vi "1820_TC_GUI.vi"() -> ()   [LabVIEW 2016]
uses:
  Leiden-TC/trunk/1. Sources TC/lib/Lib.llb/CS.lvclass
  Leiden-TC/trunk/1. Sources TC/lib/Lib.llb/TCS.lvclass
  C:/user/patrick/Leiden-TC/1. Sources TC/lib/Lib.llb/CS.lvclass
  Leiden-TC/trunk/1. Sources TC/lib/Lib.llb/QCS.lvclass
  Leiden-TC/trunk/1. Sources TC/lib/Lib.llb/CS Emulation.lvclass
  Leiden-TC/trunk/1. Sources TC/lib/Lib.llb/PCS.lvclass
panel:
  out "Name":string
  out "SetControl":T1
  out "ControlNames":string[](array[string])
  out "VIRef":T2 {"Array DataType" format="%.0x"; "WaveForm Type" format="%.0x"; "RefNum Type" format="%.0x"; "DataType" format="%.0x"}
  out "Scan Parameters":cluster{string, "Freq":dbl, "V_exc":dbl}
  out "zConfig":path=path "C:/Users/Sasha/Dropbox/Labview/LC Software/ImpSoft-V5.2.2-multithreaded/ImpBridgeLabview/ImpBridgeDll.dll"
  out "TempStabilized":refnum<user-event>
  out "Actual I":dbl[](array[numeric])
  out "VI called?":bool=TRUE
  out "Error code":u8
  out "UpdateChannelInfo":refnum<user-event>
  out "zBridge set nr.":u8
  out "zDll":path=path "C:/Users/Sasha/Dropbox/Labview/LC Software/ImpSoft-V5.2.2-multithreaded/ImpBridgeLabview/ImpBridgeDll.dll"
  in  "String":string="^ Click the Run button to start the program "
  in  "Toolbar":enum32{"Page 1", "Page 2"}(tab)
  in  "Load config":bool
  in  "Start":bool
  in  "Load Data":bool
  in  "Pause":bool
  in  "Stop":bool
  in  "Copy to Clipboard":bool
  in  "Save to Cal Log":bool
  in  "Save config":bool
  in  "Save Data":bool
  in  "Clear all plots":bool
  in  "ColorBox":enum32{"Page 1", "Page 2"}(tab)
  in  "Colors":picture
  out "Color":u32(colorbox)
  in  "LogFileCreationTime":timestamp=timestamp(2742897600 s since 1904-01-01)
  out "UpdateLogFilePath":refnum<user-event>
  out "Calib path":path=path "C:/avs-47/aaaa"
  out "Log path":path
  out "TCS port":i32(ring)=3 items=["COM1", "COM2", "COM3", "COM4", "COM5", "COM6", "COM7", "COM8", "COM9", "PRN1", "PRN2", "PRN3", "PRN4"]
  out "UpdateCalibrations":refnum<user-event>
  out "AVS VISA session":refnum<visa-resource-name>="COM3"
  in  "Minimize 2":bool
  out "Revision":string="TC" caption="V"
  in  "Minimize":bool
  out "Current1flow":bool
  out "Current2flow":bool
  in  "Tab Control":enum32{"AVS"}(tab)
  in  "Channel Controls":T3(tab)=enum."All"
  out "T0":dbl=nan caption="T" format="%#.2p"
  out "R0":dbl caption="R" format="%.3p"
  out "R-Plot 0":cluster{dbl[], dbl[]}(graph) caption="R-Plot"
  out "T1":dbl=nan caption="T" format="%#.2p"
  out "R1":dbl caption="R" format="%.3p"
  out "R-Plot 1":cluster{dbl[], dbl[]}(graph) caption="R-Plot"
  out "T2":dbl=nan caption="T" format="%#.2p"
  out "R2":dbl caption="R" format="%.3p"
  out "R-Plot 2":cluster{dbl[], dbl[]}(graph) caption="R-Plot"
  out "T3":dbl=nan caption="T" format="%#.2p"
  out "R3":dbl caption="R" format="%.3p"
  out "R-Plot 3":cluster{dbl[], dbl[]}(graph) caption="R-Plot"
  out "T4":dbl=nan caption="T" format="%#.2p"
  out "R4":dbl caption="R" format="%.3p"
  out "R-Plot 4":cluster{dbl[], dbl[]}(graph) caption="R-Plot"
  out "T5":dbl=nan caption="T" format="%#.2p"
  out "R5":dbl caption="R" format="%.3p"
  out "R-Plot 5":cluster{dbl[], dbl[]}(graph) caption="R-Plot"
  out "T6":dbl=nan caption="T" format="%#.2p"
  out "R6":dbl caption="R" format="%.3p"
  out "R-Plot 6":cluster{dbl[], dbl[]}(graph) caption="R-Plot"
  out "T7":dbl=nan caption="T" format="%#.2p"
  out "R7":dbl caption="R" format="%.3p"
  out "R-Plot 7":cluster{dbl[], dbl[]}(graph) caption="R-Plot"
  out "T8":dbl=nan caption="T" format="%#.2p"
  out "R8":dbl caption="R" format="%.3p"
  out "R-Plot 8":cluster{dbl[], dbl[]}(graph) caption="R-Plot"
  out "T9":dbl=nan caption="T" format="%#.2p"
  out "R9":dbl caption="R" format="%.3p"
  out "R-Plot 9":cluster{dbl[], dbl[]}(graph) caption="R-Plot"
  out "T":T4 {"T0 3" format="%.2p"; "T0 2" format="%.2p"; "T0" format="%.2p"; "T0" format="%.2p"; "T0" format="%.2p"; "T0" format="%.2p"; "T0" format="%.2p"; "T0" format="%.2p"; "T0" format="%.2p"; "T0" format="%.2p"}
  in  "AVS names":T5={"AVS Name 0"="3K", "AVS Name 1"="Still", "AVS Name 2"="50 mK", "AVS Name 3"="MC", "AVS Name 4"="MC", "AVS Name 5"="", "AVS Name 6"="", "AVS Name 7"="", "AVS Name 8"="", "AVS Name 9"=""}
  in  "Edit Calibrations":T6
  in  "Thermometer":T7 {"Select sensor 10" items=["No Calibration.vi"]; "Select sensor 9" items=["No Calibration.vi"]; "Select sensor 8" items=["No Calibration.vi"]; "Select sensor 7" items=["No Calibration.vi"]; "Select sensor 6" items=["No Calibration.vi"]; "Select sensor 5" items=["No Calibration.vi"]; "Select sensor 4" items=["No Calibration.vi"]; "Select sensor 3" items=["No Calibration.vi"]; "Select sensor 2" items=["No Calibration.vi"]; "Select sensor 1" items=["No Calibration.vi"]}
  out "Units":T5
  out "R":T8={"R0"=0.0, "R1"=0.0, "R2"=-0.0, "R3"=0.0, "R4"=0.0, "R5"=0.0, "R6"=0.0, "R7"=0.0, "R6 2"=0.0, "R7 2"=0.0} {"R7 2" format="%.3p"; "R6 2" format="%.3p"; "R7" format="%.3p"; "R6" format="%.3p"; "R5" format="%.3p"; "R4" format="%.3p"; "R3" format="%.3p"; "R2" format="%.3p"; "R1" format="%.3p"; "R0" format="%.3p"}
  in  "Scan Parameters":enum32{"Page 1", "Page 2"}(tab)
  in  "Exc&Ranges":T9={"Excitationl 0"=4, "Excitationl 0"=4, "Excitationl 0"=3, "Excitationl 0"=3, "Excitationl 0"=3, "Excitationl 0"=3, "Excitationl 0"=3, "Excitationl 0"=3, "Range 0"=5, "Range 0"=5, "Range 0"=5, "Range 0"=5, "Range 0"=5, "Range 0"=5, "Range 0"=5, "Range 0"=5} {"Range 0" items=["n.a."=-1, "open"=0, "2 Ohm"=1, "20 Ohm"=2, "200 Ohm"=3, "2k Ohm"=4, "20k Ohm"=5, "200k Ohm"=6, "2M Ohm"=7]; "Range 0" items=["n.a."=-1, "open"=0, "2 Ohm"=1, "20 Ohm"=2, "200 Ohm"=3, "2k Ohm"=4, "20k Ohm"=5, "200k Ohm"=6, "2M Ohm"=7]; "Range 0" items=["n.a."=-1, "open"=0, "2 Ohm"=1, "20 Ohm"=2, "200 Ohm"=3, "2k Ohm"=4, "20k Ohm"=5, "200k Ohm"=6, "2M Ohm"=7]; "Range 0" items=["n.a."=-1, "open"=0, "2 Ohm"=1, "20 Ohm"=2, "200 Ohm"=3, "2k Ohm"=4, "20k Ohm"=5, "200k Ohm"=6, "2M Ohm"=7]; "Range 0" items=["n.a."=-1, "open"=0, "2 Ohm"=1, "20 Ohm"=2, "200 Ohm"=3, "2k Ohm"=4, "20k Ohm"=5, "200k Ohm"=6, "2M Ohm"=7]; "Range 0" items=["n.a."=-1, "open"=0, "2 Ohm"=1, "20 Ohm"=2, "200 Ohm"=3, "2k Ohm"=4, "20k Ohm"=5, "200k Ohm"=6, "2M Ohm"=7]; "Range 0" items=["n.a."=-1, "open"=0, "2 Ohm"=1, "20 Ohm"=2, "200 Ohm"=3, "2k Ohm"=4, "20k Ohm"=5, "200k Ohm"=6, "2M Ohm"=7]; "Range 0" items=["n.a."=-1, "open"=0, "2 Ohm"=1, "20 Ohm"=2, "200 Ohm"=3, "2k Ohm"=4, "20k Ohm"=5, "200k Ohm"=6, "2M Ohm"=7]; "Excitationl 0" items=["none", "3 µV", "10 µV", "30 µV", "100 µV", "300 µV", "1 mV", "3 mV"]; "Excitationl 0" items=["none", "3 µV", "10 µV", "30 µV", "100 µV", "300 µV", "1 mV", "3 mV"]; "Excitationl 0" items=["none", "3 µV", "10 µV", "30 µV", "100 µV", "300 µV", "1 mV", "3 mV"]; "Excitationl 0" items=["none", "3 µV", "10 µV", "30 µV", "100 µV", "300 µV", "1 mV", "3 mV"]; "Excitationl 0" items=["none", "3 µV", "10 µV", "30 µV", "100 µV", "300 µV", "1 mV", "3 mV"]; "Excitationl 0" items=["none", "3 µV", "10 µV", "30 µV", "100 µV", "300 µV", "1 mV", "3 mV"]; "Excitationl 0" items=["none", "3 µV", "10 µV", "30 µV", "100 µV", "300 µV", "1 mV", "3 mV"]; "Excitationl 0" items=["none", "3 µV", "10 µV", "30 µV", "100 µV", "300 µV", "1 mV", "3 mV"]}
  out "Status":T10
  out "zBridge params":T5
  out "uPlots":T11
  in  "Autorange":bool=TRUE
  out "Active":T12={"active Channel 0"=TRUE, "active Channel 1"=TRUE, "active Channel 2"=TRUE, "active Channel 3"=FALSE, "active Channel 4"=FALSE, "active Channel 5"=FALSE, "active Channel 6"=FALSE, "active Channel 7"=FALSE, "active Channel 8"=FALSE, "active Channel 9"=FALSE}
  out "PID-Plot":cluster{"Numeric":dbl, "R/T":dbl}(graph)
  in  "HW Address":u32
  in  "Edit calibration":bool
  in  "Convert":bool
  out "T7":dbl caption="T=" format="%#.2p"
  in  "QuickR":dbl caption="R=" format="%_6g"
  in  "Select sensor 1":u16(ring) items=["No Calibration.vi"]
  out "I_list[i]":dbl[](array[numeric]) min=-1.0
  out "I_in":dbl[](array[numeric]) min=-1.0
  in  "Tab Control 5":enum32{"Page 1", "Page 2"}(tab)
  in  "Data History":enum32{"History", "Settings"}(tab)=enum."Settings"
  in  "Mode Buttons":T13(radio)
  in  "Erase All":bool
  out "AVS names small":T5={"AVS Name 0"="3K", "AVS Name 1"="Still", "AVS Name 2"="50 mK", "AVS Name 3"="MC", "AVS Name 4"="MC", "AVS Name 5"="", "AVS Name 6"="", "AVS Name 7"="", "AVS Name 8"="", "AVS Name 9"=""}
  out "Active channel":T14
  out "Small T":T15 caption="T" {"R1" format="%#.2p"; "R1" format="%#.2p"; "R1" format="%#.2p"; "R1" format="%#.2p"; "R1" format="%#.2p"; "R1" format="%#.2p"; "R1" format="%#.2p"; "R1" format="%#.2p"; "R1" format="%#.2p"; "R1" format="%#.2p"}
  out "Small R":T16 caption="R" {"R1 2" format="%#_5p"; "R1 2" format="%#_5p"; "R1 2" format="%#_5p"; "R1 2" format="%#_5p"; "R1 2" format="%#_5p"; "R1 2" format="%#_5p"; "R1 2" format="%#_5p"; "R1 2" format="%#_5p"; "R1 2" format="%#_5p"; "R1 2" format="%#_5p"}
  out "Time":dbl format="%<%X\n%x>T"
  in  "AVS Runtime Settings":T17={"Read AVS channels from"=0, "Last Channel"=7, "Delay Between Scans"=0, "Stabilisation Delay"=0.5, "Averages"=2, "Data Memory"=5000, "Filter graphs:"=FALSE, "Y_min"=0.0, "Y_max"=2000000.0, "Plot type"=enum."T vs Time", "Allow neg R"=TRUE, "Data Memory 2"=30.0} {"Data Memory 2" min=0.0; "Delay Between Scans" format="%.0f s"; "Averages" min=1 max=1000; "Stabilisation Delay" min=0.5; "Last Channel" min=0 max=7 step=1; "Read AVS channels from" min=0 max=7 step=1; "Y_max" format="%#_6f"; "Y_min" min=0.0 format="%#_6f"; "Data Memory" min=3 max=30000}
  out "I":dbl[](array[numeric])
  in  "Data":cluster{"R":dbl[], "T":dbl[], "Time":dbl[]}[](array[cluster])=[{"R"=[], "T"=[], "Time"=[]}, {"R"=[0.0, 2.0], "T"=[], "Time"=[]}]
  out "Int":dbl=10.0 format="%#.2f"
  out "T_array":dbl[](array[numeric])
  in  "Data array":dbl[](array[numeric])
  out "I3_SetPnt":dbl
  out "Currents changed":bool
  in  "Excitations":T18={"Excitationl 0"=4, "Excitation 1"=4, "Excitation 2"=3, "Excitation 3"=3, "Excitation 4"=3, "Excitation 5"=3, "Excitation 6"=3, "Excitation 7"=3} {"Excitation 7" items=["none", "3 µV", "10 µV", "30 µV", "100 µV", "300 µV", "1 mV", "3 mV"]; "Excitation 6" items=["none", "3 µV", "10 µV", "30 µV", "100 µV", "300 µV", "1 mV", "3 mV"]; "Excitation 5" items=["none", "3 µV", "10 µV", "30 µV", "100 µV", "300 µV", "1 mV", "3 mV"]; "Excitation 4" items=["none", "3 µV", "10 µV", "30 µV", "100 µV", "300 µV", "1 mV", "3 mV"]; "Excitation 3" items=["none", "3 µV", "10 µV", "30 µV", "100 µV", "300 µV", "1 mV", "3 mV"]; "Excitation 2" items=["none", "3 µV", "10 µV", "30 µV", "100 µV", "300 µV", "1 mV", "3 mV"]; "Excitation 1" items=["none", "3 µV", "10 µV", "30 µV", "100 µV", "300 µV", "1 mV", "3 mV"]; "Excitationl 0" items=["none", "3 µV", "10 µV", "30 µV", "100 µV", "300 µV", "1 mV", "3 mV"]}
  in  "Ranges":T18={"Excitationl 0"=5, "Excitation 1"=5, "Excitation 2"=5, "Excitation 3"=5, "Excitation 4"=5, "Excitation 5"=5, "Excitation 6"=5, "Excitation 7"=5} {"Excitation 7" items=["n.a."=-1, "open"=0, "2 Ohm"=1, "20 Ohm"=2, "200 Ohm"=3, "2k Ohm"=4, "20k Ohm"=5, "200k Ohm"=6, "2M Ohm"=7]; "Excitation 6" items=["n.a."=-1, "open"=0, "2 Ohm"=1, "20 Ohm"=2, "200 Ohm"=3, "2k Ohm"=4, "20k Ohm"=5, "200k Ohm"=6, "2M Ohm"=7]; "Excitation 5" items=["n.a."=-1, "open"=0, "2 Ohm"=1, "20 Ohm"=2, "200 Ohm"=3, "2k Ohm"=4, "20k Ohm"=5, "200k Ohm"=6, "2M Ohm"=7]; "Excitation 4" items=["n.a."=-1, "open"=0, "2 Ohm"=1, "20 Ohm"=2, "200 Ohm"=3, "2k Ohm"=4, "20k Ohm"=5, "200k Ohm"=6, "2M Ohm"=7]; "Excitation 3" items=["n.a."=-1, "open"=0, "2 Ohm"=1, "20 Ohm"=2, "200 Ohm"=3, "2k Ohm"=4, "20k Ohm"=5, "200k Ohm"=6, "2M Ohm"=7]; "Excitation 2" items=["n.a."=-1, "open"=0, "2 Ohm"=1, "20 Ohm"=2, "200 Ohm"=3, "2k Ohm"=4, "20k Ohm"=5, "200k Ohm"=6, "2M Ohm"=7]; "Excitation 1" items=["n.a."=-1, "open"=0, "2 Ohm"=1, "20 Ohm"=2, "200 Ohm"=3, "2k Ohm"=4, "20k Ohm"=5, "200k Ohm"=6, "2M Ohm"=7]; "Excitationl 0" items=["n.a."=-1, "open"=0, "2 Ohm"=1, "20 Ohm"=2, "200 Ohm"=3, "2k Ohm"=4, "20k Ohm"=5, "200k Ohm"=6, "2M Ohm"=7]}
  out "CS ref":refnum<class "CS.lvclass">
  out "start 2":bool
  in  "Current indicators":enum32{"Page 1", "Page 2"}(tab)
  out "Automatic mode 0":bool
  out "Automatic mode 1":bool
  out "Map Channel 0 to 2":T19(ring) caption="Output to"
  in  "uA 0":u32
  in  "CS Names":T20={"CS Name 0"="N.C.", "CS Name 1"="3K", "CS Name 2"="Still", "CS Name 3"="MC"}
  out "I0":T21={"uA"="000", "ON"=FALSE, "Gated"=FALSE, "current flows"=FALSE, "Error"=FALSE} caption="Ch0 -"
  in  "uA 3":u32
  in  "uA 2":u32
  in  "uA 1":u32
  out "Automatic mode 3":bool
  out "Automatic mode 2":bool
  out "I3":T21={"uA"="000", "ON"=FALSE, "Gated"=FALSE, "current flows"=FALSE, "Error"=FALSE} caption="Chn 3"
  out "I2":T21={"uA"="000", "ON"=FALSE, "Gated"=FALSE, "current flows"=FALSE, "Error"=FALSE} caption="Chn 2"
  out "I1":T21={"uA"="000", "ON"=FALSE, "Gated"=FALSE, "current flows"=FALSE, "Error"=FALSE} caption="Chn 1"
  out "I_0":dbl=10.0
  out "vi reference":refnum<vi>
  in  "Show PID graph?":bool
  in  "Set Color":bool
  in  "Save Screen Data":bool
  in  "CS Ch3 mode":enum32{"Page 1", "Page 2"}(tab)=enum."Page 2"
  in  "T Sweep":T22={"Start value"=200.0, "End value"=250.0, "Step"=10.0, "Current"=0.0, "I_next"=FALSE, "I_prev"=FALSE, "Interrrupt Sweep"=FALSE, "Start"=FALSE, "Boolean"=TRUE} {"Step" min=0.0; "End value" min=0.0; "Start value" min=0.0}
  out "CallExtVI":refnum<user-event>
  out "Unit":string
  out "UpdateValuesAVS":refnum<user-event>
  out "DoPID":refnum<user-event>
  out "UpdateValuesZBridge":refnum<user-event>
  out "zBridge params/Error":string
  out "CurCalibrations":T23
  out "LMB Down":bool
  out "T controlled":dbl
  out "ResetPIDloop":refnum<user-event>
  in  "Tab Control 2":T24(tab)=enum."Current source control"
  in  "Refresh Calibrations":bool
  in  "Save Screen Data 2":bool
  out "ID":string
  out "Bridge status":errorcluster
  out "CS status":errorcluster
  out "General":errorcluster caption="General status"
  in  "Bridge settings":T25={"AVS type"=enum."AVS47A (GPIB interface)", "AVS_SPort"="COM5", "Address"="GPIB0::20::INSTR", "AVS_CalFolder"=path "E:/Dropbox/Labview/LC Software/All Calibrations"}
  in  "Current source settings":T26={"TCS_Port"="COM1", "TCS_Imax"=5, "CS type"=enum."TCS", "QCS/PCS Device"=0}
  in  "Data logging":T27={"AVS_Path"=path "C:/avs-47", "AVS_FName"="LogAVS", "CAL_FName"="calibration", "Filenames suffix"="_%Y-%m-%d-%H-%M-%S", "Delimeter"="\t", "NewFevery"=7, "Time Units"=enum."Days", "Date/Time Format"="%Y-%m-%d %H:%M:%S", "External VI path"=path "C:/Users/User1/Dropbox/Labview/LC Software/TempControl/OnTempStabilized Ext VI Laurens.vi", "VI state:"=enum."Bad", "Ask on start?"=FALSE, "Run description"="\n"}
  in  "I_list":dbl[][](array[numeric]) min=-1.0
  out "T Channel":bool[](array[boolean])
  in  "Trigger other running TC instances":bool
  in  "I_Clear":bool
  in  "I3 as temp":cluster{"I3 as temp 2":bool}
  in  "C_I3":T28={"Toggle ON/OFF"=FALSE, "Toggle Gated"=FALSE, "I"=0, "Range"=enum."x1 uA"} caption="I3" {"I" max=100000 step=1}
  in  "C_I2":T28={"Toggle ON/OFF"=FALSE, "Toggle Gated"=FALSE, "I"=0, "Range"=enum."x1 uA"} caption="I2" {"I" max=100000 step=1}
  in  "C_I1":T28={"Toggle ON/OFF"=FALSE, "Toggle Gated"=FALSE, "I"=0, "Range"=enum."x1 uA"} caption="I1" {"I" max=100000 step=1}
  in  "C_I0":T28={"Toggle ON/OFF"=FALSE, "Toggle Gated"=FALSE, "I"=0, "Range"=enum."x1 uA"} caption="I0" {"I" max=100000 step=1}
  in  "I0 output to":T29(ring) caption="Set QCS Channel 0 output to"
  in  "CS Mode":enum16{"Manual", "Automatic"}(ring) caption="CS control mode"
  in  "Write to log":bool
  in  "Load from file":bool
  in  "Save to file":bool
  in  "I_tofirst":bool
  in  "I_next":bool
  in  "I_prev":bool
  out "VI state:":T30(ring)
  out "I_selection":bool[](array[boolean])=[TRUE, FALSE, FALSE, FALSE, FALSE, FALSE, FALSE, FALSE, FALSE, FALSE]
  in  "Call external VI":bool
  out "Time Old":dbl format="%#_16g"
  in  "Automode Settings 2":T31={"AVS Channel"=0, "N averages"=10, "Delay Time"=10.0, "T stability"=0.3, "FB on"=enum."Temperature"} {"Delay Time" min=0.0 format="%#_g min"; "AVS Channel" min=-1 max=9 step=1}
  in  "Automode 2":bool=TRUE caption="Enable automatic sweeping/list iteration"
  in  "PID setup 2":T32={"Current limit, [uA]"=10000.0, "Proportional Gain"=3.0, "Integral Gain"=3.0, "Derivative Gain"=1.0, "SP tolerance"=0.1, "Feed Fwd Gain [uA/mK]"=0.0, "Integral Gain Bandwidth"=10.0, "Integral Gain Background"=1.0, "FB on 2"=enum."1"} {"Integral Gain Background" format="%#.6g"; "Integral Gain Bandwidth" format="%#.6g"; "Feed Fwd Gain [uA/mK]" format="%#.5g"; "SP tolerance" format="%#.5g"; "Derivative Gain" format="%#.6g"; "Integral Gain" format="%#.6g"; "Proportional Gain" format="%#.6g"; "Current limit, [uA]" format="%#.5g"}
  in  "Reset PID":bool
  in  "Next step":bool
  out "I_list_idx":i32=10 caption="Point #"
  out "I_list_idx_max":i32=10 caption="of"
  out "Timer":dbl format="%<%H:%M:%S>t"
  out "Slope":dbl format="%#_3g %"
  out "Error":dbl=10.0 format="%#_6f"
  out "SP reached?":bool
  # "Quick convert R->T:"
  # "Ohm"
  # "mK"
  # "Ch#"
  # "Miniplot"
  # "Channel parameters"
  # "Impedance"
  # "Unit"
  # "Type of sensor"
  # "T [mK]"
  # "Description"
  # "0"
  # "1"
  # "2"
  # "3"
  # "4"
  # "5"
  # "6"
  # "7"
  # "8"
  # "9"
  # "0"
  # "1"
  # "2"
  # "3"
  # "4"
  # "5"
  # "7"
  # "8"
  # "9"
  # "6"
  # "auto"
  # "auto"
  # "auto"
  # "auto"
  # "gated"
  # "gated"
  # "gated"
  # "gated"
  # "Ch3"
  # "Current source mode"
  # "Current source manual control"
  # "Automatic mode or current source"
  # "Currents List"
  # "Settings"
  # "I0"
  # "I1"
  # "I2"
  # "I3"
  # "Status"
  # "On temperature stabilized"
types:
  T1 = cluster{"Name":string, "Scalar":string, "Array":string[][]}
  T2 = cluster{"Control Ref ID":refnum<vi>[], "Full Name":string[], "ClassID":enum16{"<Null>", "1", "2", "Generic", "Decoration", "Text", "Control", "ColorBox", "Boolean", "RefNum", "Variant", "Path", "ListBox", "Table", "Array", "Picture", "ActiveXContainer", "Numeric", "Digital", "NamedNumeric", "ColorRamp", "Slide", "GraphOrChart", "WaveformChart", "WaveformGraph", "IntensityChart", "IntensityGraph", "String", "IOName", "ComboBox", "Cluster", "Panel", "Knob", "NumWithScale", "Ring", "Enum", "GObject", "Plot", "Cursor", "NumericText", "Scale", "ColorScale", "GraphScale", "ColorGraphScale", "TypedRefNum", "OldKnobScale", "MCListbox", "MeasureData", "BVTag", "DAQName", "VISAName", "IVIName", "SlideScale", "TabControl", "Page", "TabArrayTabControl", "ConPane", "57", "58", "59", "60", "61", "62", "63", "64", "SubPanel", "TreeControl", "67", "68", "69", "70", "71", "72", "73", "74", "75", "SplitterBar"}[], "Short Name":string[], "DataType":enum8{"<Null>", "I8", "I16", "I32", "I64", "U8", "U16", "U32", "U64", "SGL", "DBL", "EXT", "CSG", "CDB", "CXT", "0x0F", "0x10", "0x11", "0x12", "0x13", "0x14", "Enum U8", "Enum U16", "Enum U32", "Enum U64", "SGL PQ", "DBL PQ", "EXT PQ", "CSG PQ", "CDB PQ", "CXT PQ", "0x1F", "0x20", "Boolean", "0x22", "0x23", "0x24", "0x25", "0x26", "0x27", "0x28", "0x29", "0x2A", "0x2B", "0x2C", "0x2D", "0x2E", "0x2F", "String", "0x31", "Path", "Pict", "0x34", "0x35", "0x36", "DAQ", "0x38", "0x39", "0x3A", "0x3B", "0x3C", "0x3D", "0x3E", "0x3F", "Array", "0x41", "0x42", "0x43", "0x44", "0x45", "0x46", "0x47", "0x48", "0x49", "0x4A", "0x4B", "0x4C", "0x4D", "0x4E", "0x4F", "Cluster", "0x51", "0x52", "Variant", "Waveform", "0x55", "0x56", "0x57", "0x58", "0x59", "0x5A", "0x5B", "0x5C", "0x5D", "0x5E", "0x5F", "0x60", "0x61", "0x62", "0x63", "0x64", "0x65", "0x66", "0x67", "0x68", "0x69", "0x6A", "0x6B", "0x6C", "0x6D", "0x6E", "0x6F", "Refnum"}[], "RefNum Type":enum8{"Generic", "Datalog File Refnum", "Byte Stream File Refnum", "Device Refnum", "Occurence Refnum", "TCP Connection Refnum", "VISA Refnum (Obsolete)", "Automation Renum", "VI Server Refnum", "Menu Refnum", "IVI Refnum (Obsolete)", "IMAQ Session", "0x0C", "Datasocket Refnum", "VISA Resource", "IVI Logical Name", "UDP Connection Refnum", "Notifier Refnum", "Queue Refnum", "IrDA Refnum", "Hardware Plugin Refnum", "Hardware Plugin Tag Refnum", "DAQmx Refnum", "Event Registration Refnum", ".NET Refnum", "User Event Refnum", "0x1A", "Event Callback", "0x1C", "0x1D", "Only Used Internal to LabVIEW", "Bluetooth", "Data Value References", "RT FIFO", "TDM Streaming"}[], "WaveForm Type":enum8{"<Not a Waveform Type>", "0x01", "Analog 16-bit signed", "Analog Double-Precision", "0x04", "Analog Single Precision", "Timestamp", "Digital Data", "Digital Waveform", "Dynamic Data", "Analog Extended-Precision", "Analog 8-bit unsigned", "Analog 16-bit unsigned", "Analog 32-bit unsigned", "Analog 8-bit signed", "Analog 32-bit signed", "Analog Complex Single-Precision", "Analog Complex Double-Precision", "Analog Complex Extended Precision", "Analog 64-bit signed", "Analog 64-bit unsigned"}[], "Parent":i32[], "Array DataType":enum8{"<Null>", "I8", "I16", "I32", "I64", "U8", "U16", "U32", "U64", "SGL", "DBL", "EXT", "CSG", "CDB", "CXT", "0x0F", "0x10", "0x11", "0x12", "0x13", "0x14", "Enum U8", "Enum U16", "Enum U32", "Enum U64", "SGL PQ", "DBL PQ", "EXT PQ", "CSG PQ", "CDB PQ", "CXT PQ", "0x1F", "0x20", "Boolean", "0x22", "0x23", "0x24", "0x25", "0x26", "0x27", "0x28", "0x29", "0x2A", "0x2B", "0x2C", "0x2D", "0x2E", "0x2F", "String", "0x31", "Path", "Pict", "0x34", "0x35", "0x36", "DAQ", "0x38", "0x39", "0x3A", "0x3B", "0x3C", "0x3D", "0x3E", "0x3F", "Array", "0x41", "0x42", "0x43", "0x44", "0x45", "0x46", "0x47", "0x48", "0x49", "0x4A", "0x4B", "0x4C", "0x4D", "0x4E", "0x4F", "Cluster", "0x51", "0x52", "Variant", "Waveform", "0x55", "0x56", "0x57", "0x58", "0x59", "0x5A", "0x5B", "0x5C", "0x5D", "0x5E", "0x5F", "0x60", "0x61", "0x62", "0x63", "0x64", "0x65", "0x66", "0x67", "0x68", "0x69", "0x6A", "0x6B", "0x6C", "0x6D", "0x6E", "0x6F", "Refnum"}[], "Owning VI":refnum<vi>[], "Active?":bool[]}
  T3 = enum32{"0", "1", "2", "3", "4", "5", "6", "7", "8", "9", "All", "PID loop"}
  T4 = cluster{"T0":dbl, "T0":dbl, "T0":dbl, "T0":dbl, "T0":dbl, "T0":dbl, "T0":dbl, "T0":dbl, "T0 2":dbl, "T0 3":dbl}
  T5 = cluster{"AVS Name 0":string, "AVS Name 1":string, "AVS Name 2":string, "AVS Name 3":string, "AVS Name 4":string, "AVS Name 5":string, "AVS Name 6":string, "AVS Name 7":string, "AVS Name 8":string, "AVS Name 9":string}
  T6 = cluster{"Boolean":bool, "Boolean 2":bool, "Boolean 3":bool, "Boolean 4":bool, "Boolean 5":bool, "Boolean 6":bool, "Boolean 7":bool, "Boolean 8":bool, "Boolean 9":bool, "Boolean 10":bool}
  T7 = cluster{"Select sensor 1":u16, "Select sensor 2":u16, "Select sensor 3":u16, "Select sensor 4":u16, "Select sensor 5":u16, "Select sensor 6":u16, "Select sensor 7":u16, "Select sensor 8":u16, "Select sensor 9":u16, "Select sensor 10":u16}
  T8 = cluster{"R0":dbl, "R1":dbl, "R2":dbl, "R3":dbl, "R4":dbl, "R5":dbl, "R6":dbl, "R7":dbl, "R6 2":dbl, "R7 2":dbl}
  T9 = cluster{"Excitationl 0":i16, "Excitationl 0":i16, "Excitationl 0":i16, "Excitationl 0":i16, "Excitationl 0":i16, "Excitationl 0":i16, "Excitationl 0":i16, "Excitationl 0":i16, "Range 0":i16, "Range 0":i16, "Range 0":i16, "Range 0":i16, "Range 0":i16, "Range 0":i16, "Range 0":i16, "Range 0":i16}
  T10 = cluster{"Numeric":dbl, "Numeric":dbl, "Numeric":dbl, "Numeric":dbl, "Numeric":dbl, "Numeric":dbl, "Numeric":dbl, "Numeric":dbl, "Numeric":dbl, "Numeric":dbl}
  T11 = cluster{"uPlot 0":cluster{dbl[], dbl[]}, "uPlot 1":cluster{dbl[], dbl[]}, "uPlot 2":cluster{dbl[], dbl[]}, "uPlot 3":cluster{dbl[], dbl[]}, "uPlot 4":cluster{dbl[], dbl[]}, "uPlot 5":cluster{dbl[], dbl[]}, "uPlot 6":cluster{dbl[], dbl[]}, "uPlot 7":cluster{dbl[], dbl[]}, "uPlot 8":cluster{dbl[], dbl[]}, "uPlot 9":cluster{dbl[], dbl[]}}
  T12 = cluster{"active Channel 0":bool, "active Channel 1":bool, "active Channel 2":bool, "active Channel 3":bool, "active Channel 4":bool, "active Channel 5":bool, "active Channel 6":bool, "active Channel 7":bool, "active Channel 8":bool, "active Channel 9":bool}
  T13 = enum32{"No Selection", "Cursor Mode", "Erase point", "Erase Range"}
  T14 = cluster{"Boolean 5":bool, "Boolean 5":bool, "Boolean 5":bool, "Boolean 5":bool, "Boolean 5":bool, "Boolean 5":bool, "Boolean 5":bool, "Boolean 5":bool, "Boolean 5":bool, "Boolean 5":bool}
  T15 = cluster{"R1":dbl, "R1":dbl, "R1":dbl, "R1":dbl, "R1":dbl, "R1":dbl, "R1":dbl, "R1":dbl, "R1":dbl, "R1":dbl}
  T16 = cluster{"R1 2":dbl, "R1 2":dbl, "R1 2":dbl, "R1 2":dbl, "R1 2":dbl, "R1 2":dbl, "R1 2":dbl, "R1 2":dbl, "R1 2":dbl, "R1 2":dbl}
  T17 = cluster{"Read AVS channels from":i8, "Last Channel":i8, "Delay Between Scans":u32, "Stabilisation Delay":dbl, "Averages":u16, "Data Memory":u16, "Filter graphs:":bool, "Y_min":dbl, "Y_max":dbl, "Plot type":enum16{"R vs Time", "T vs Time"}, "Allow neg R":bool, "Data Memory 2":dbl}
  T18 = cluster{"Excitationl 0":i16, "Excitation 1":i16, "Excitation 2":i16, "Excitation 3":i16, "Excitation 4":i16, "Excitation 5":i16, "Excitation 6":i16, "Excitation 7":i16}
  T19 = enum16{"Chn 0", "Aux 0", "Aux 1", "Aux 2", "Aux 3"}
  T20 = cluster{"CS Name 0":string, "CS Name 1":string, "CS Name 2":string, "CS Name 3":string}
  T21 = cluster{"uA":string, "ON":bool, "Gated":bool, "current flows":bool, "Error":bool}
  T22 = cluster{"Start value":dbl, "End value":dbl, "Step":dbl, "Current":dbl, "I_next":bool, "I_prev":bool, "Interrrupt Sweep":bool, "Start":bool, "Boolean":bool}
  T23 = cluster{"[0]":string, "[1]":string, "[2]":string, "[3]":string, "[4]":string, "[5]":string, "[6]":string, "[7]":string, "[8]":string, "[9]":string}
  T24 = enum32{"Devices Settings", "Current source control"}
  T25 = cluster{"AVS type":enum16{"AVS47A (GPIB interface)", "AVS47B (RS232 interface)", "AVS48", "AVS Emulation", "Impedance Bridge", "Disabled"}, "AVS_SPort":refnum<visa-resource-name>, "Address":refnum<visa-resource-name>, "AVS_CalFolder":path}
  T26 = cluster{"TCS_Port":refnum<visa-resource-name>, "TCS_Imax":i32, "CS type":enum16{"TCS", "QCS v1", "PCS (n.a.)", "CS Emulation", "Disabled"}, "QCS/PCS Device":u16}
  T27 = cluster{"AVS_Path":path, "AVS_FName":string, "CAL_FName":string, "Filenames suffix":string, "Delimeter":string, "NewFevery":u32, "Time Units":enum16{"Minutes", "Hours", "Days"}, "Date/Time Format":string, "External VI path":path, "VI state:":enum32{"Bad", "Idle", "Run top level", "Running"}, "Ask on start?":bool, "Run description":string}
  T28 = cluster{"Toggle ON/OFF":bool, "Toggle Gated":bool, "I":u32, "Range":enum8{"Auto", "x1 uA", "x10 uA", "x100 uA", "x1 mA"}}
  T29 = enum16{"Channel 0", "Aux 0", "Aux 1", "Aux 2", "Aux 3"}
  T30 = enum32{"Bad", "Idle", "Run top level", "Running"}
  T31 = cluster{"AVS Channel":i32, "N averages":i32, "Delay Time":dbl, "T stability":dbl, "FB on":enum16{"Resistance", "Temperature"}}
  T32 = cluster{"Current limit, [uA]":dbl, "Proportional Gain":dbl, "Integral Gain":dbl, "Derivative Gain":dbl, "SP tolerance":dbl, "Feed Fwd Gain [uA/mK]":dbl, "Integral Gain Bandwidth":dbl, "Integral Gain Background":dbl, "FB on 2":enum16{"0", "1", "2", "3"}}
  T33 = cluster{"error":bool, "code":i32, "source":string}
  T34 = enum32{"No Selection", "Erase Data", "Erase Range", "Cursor Mode"}
  T35 = enum16{"AVS47A (GPIB interface)", "AVS47B (RS232 interface)", "AVS48", "AVS Emulation", "Impedance Bridge", "Disabled"}
  T36 = enum16{"TCS", "QCS v1", "PCS (n.a.)", "CS Emulation", "Disabled"}
  T37 = enum8{"Auto", "x1 uA", "x10 uA", "x100 uA", "x1 mA"}
  T38 = cluster{"Cluster":cluster{"Time":dbl[], "T":dbl[]}, "Cluster":cluster{"Time":dbl[], "T":dbl[]}, "Cluster":cluster{"Time":dbl[], "T":dbl[]}, "Cluster":cluster{"Time":dbl[], "T":dbl[]}, "Cluster":cluster{"Time":dbl[], "T":dbl[]}, "Cluster":cluster{"Time":dbl[], "T":dbl[]}, "Cluster":cluster{"Time":dbl[], "T":dbl[]}, "Cluster":cluster{"Time":dbl[], "T":dbl[]}, "Cluster":cluster{"Time":dbl[], "T":dbl[]}, "Cluster":cluster{"Time":dbl[], "T":dbl[]}}
  T39 = enum32{"HKEY_CLASSES_ROOT", "HKEY_CURRENT_USER", "HKEY_LOCAL_MACHINE", "HKEY_USERS", "HKEY_PERFORMANCE_DATA", "HKEY_CURRENT_CONFIG", "HKEY_DYN_DATA"}
  T40 = enum32{"invalid app kind", "Development System", "Run Time System", "Student Edition", "Embedded LabVIEW", "Evaluation", "Custom"}
  T41 = cluster{"[0]":dbl, "[1]":dbl, "[2]":dbl, "[3]":dbl, "[4]":dbl, "[5]":dbl, "[6]":dbl, "[7]":dbl, "[8]":dbl, "[9]":dbl}
  T42 = cluster{"Temperature[0]":dbl, "Temperature[1]":dbl, "Temperature[2]":dbl, "Temperature[3]":dbl, "Temperature[4]":dbl, "Temperature[5]":dbl, "Temperature[6]":dbl, "Temperature[7]":dbl, "Temperature[8]":dbl, "Temperature[9]":dbl}
  T43 = cluster{"type":string, "creator":string, "permissions":i32, "data size":i32, "res size":i32, "creation date":u32, "modification date":u32, "bFolder":bool, "bInvisible":bool, "location":cluster{"vertical":i16, "horizontal":i16}, "owner":string, "group":string}
  T44 = cluster{"Units[0]":string, "Units[1]":string, "Units[2]":string, "Units[3]":string, "Units[4]":string, "Units[5]":string, "Units[6]":string, "Units[7]":string, "Units[8]":string, "Units[9]":string}
  T45 = cluster{"zBridge params[0]":string, "zBridge params[1]":string, "zBridge params[2]":string, "zBridge params[3]":string, "zBridge params[4]":string, "zBridge params[5]":string, "zBridge params[6]":string, "zBridge params[7]":string, "zBridge params[8]":string, "zBridge params[9]":string}
  T46 = cluster{"date/time string":string, "Value":dbl[], "Value":dbl[], "Value":dbl[]}
  T47 = typedef "imagedata.ctl" = cluster{"image type":i32, "image depth":i32, "image":u8[], "mask":u8[], "colors":u32[], "Rectangle":cluster{"left":i16, "top":i16, "right":i16, "bottom":i16}}
  T48 = typedef "LVPoint32TypeDef.ctl" = cluster{"Horizontal":i32, "Vertical":i32}
  T49 = cluster{"Output Array":dbl[], "array w/ subset deleted":dbl[], "array w/ subset deleted":dbl[]}
  T50 = typedef "LVRectTypeDef.ctl" = cluster{"Left":i16, "Top":i16, "Right":i16, "Bottom":i16}
  T51 = cluster{"Excitationl 0":i16, "Excitation 1":i16, "Excitation 2":i16, "Excitation 3":i16, "Excitation 4":i16, "Excitation 5":i16, "Excitation 6":i16, "Excitation 7":i16, "Range 0":i16, "Range 1":i16, "Range 2":i16, "Range 3":i16, "Range 4":i16, "Range 5":i16, "Range 6":i16, "Range 7":i16}
  T52 = enum8{"Active", "Channel Type", "Channel No", "Reference No", "RLC select", "Save Data", "L Inverted", "Menu Active"}
  T53 = typedef "LVPositionTypeDef.ctl" = cluster{"Left":i32, "Top":i32}
  T54 = cluster{"Range 0":i16, "Range 1":i16, "Range 2":i16, "Range 3":i16, "Range 4":i16, "Range 7":i16, "Range 5":i16, "Range 6":i16}
  T55 = cluster{"Range 0":i16, "Range 1":i16, "Range 2":i16, "Range 3":i16, "Range 4":i16, "Range 5":i16, "Range 6":i16, "Range 7":i16}
  T56 = cluster{"RANGE 0":u16, "RANGE 1":u16, "RANGE 2":u16, "RANGE 3":u16, "RANGE 4":u16, "RANGE 5":u16, "RANGE 6":u16, "RANGE 7":u16}
  T57 = cluster{"Range":u8, "Current":dbl, "Current (string)":string, "On?":bool, "G?":bool, "I?":bool, "Err?":bool}
  T58 = cluster{"uA":string, " ON":bool, "Gated":bool, "current flows":bool, "Error":bool}
  T59 = cluster{"Toggle ON/OFF":bool, "Toggle Gated":bool}
  T60 = cluster{"Current":u32, "Range":enum16{"Auto", "x1 uA", "x10 uA", "x100 uA", "x1 mA"}}
  T61 = cluster{"Toggle ON/OFF":bool, "Toggle Gated":bool, "Current":u32, "Range":enum8{"Auto", "x1 uA", "x10 uA", "x100 uA", "x1 mA"}}
  T62 = cluster{"Status[0]":i32, "Status[1]":i32, "Status[2]":i32, "Status[3]":i32, "Status[4]":i32, "Status[5]":i32, "Status[6]":i32, "Status[7]":i32, "Status[8]":i32, "Status[9]":i32}
  T63 = cluster{"Active":bool, "Active":bool, "Active":bool, "Active":bool, "Active":bool, "Active":bool, "Active":bool, "Active":bool, "Active":bool, "Active":bool}
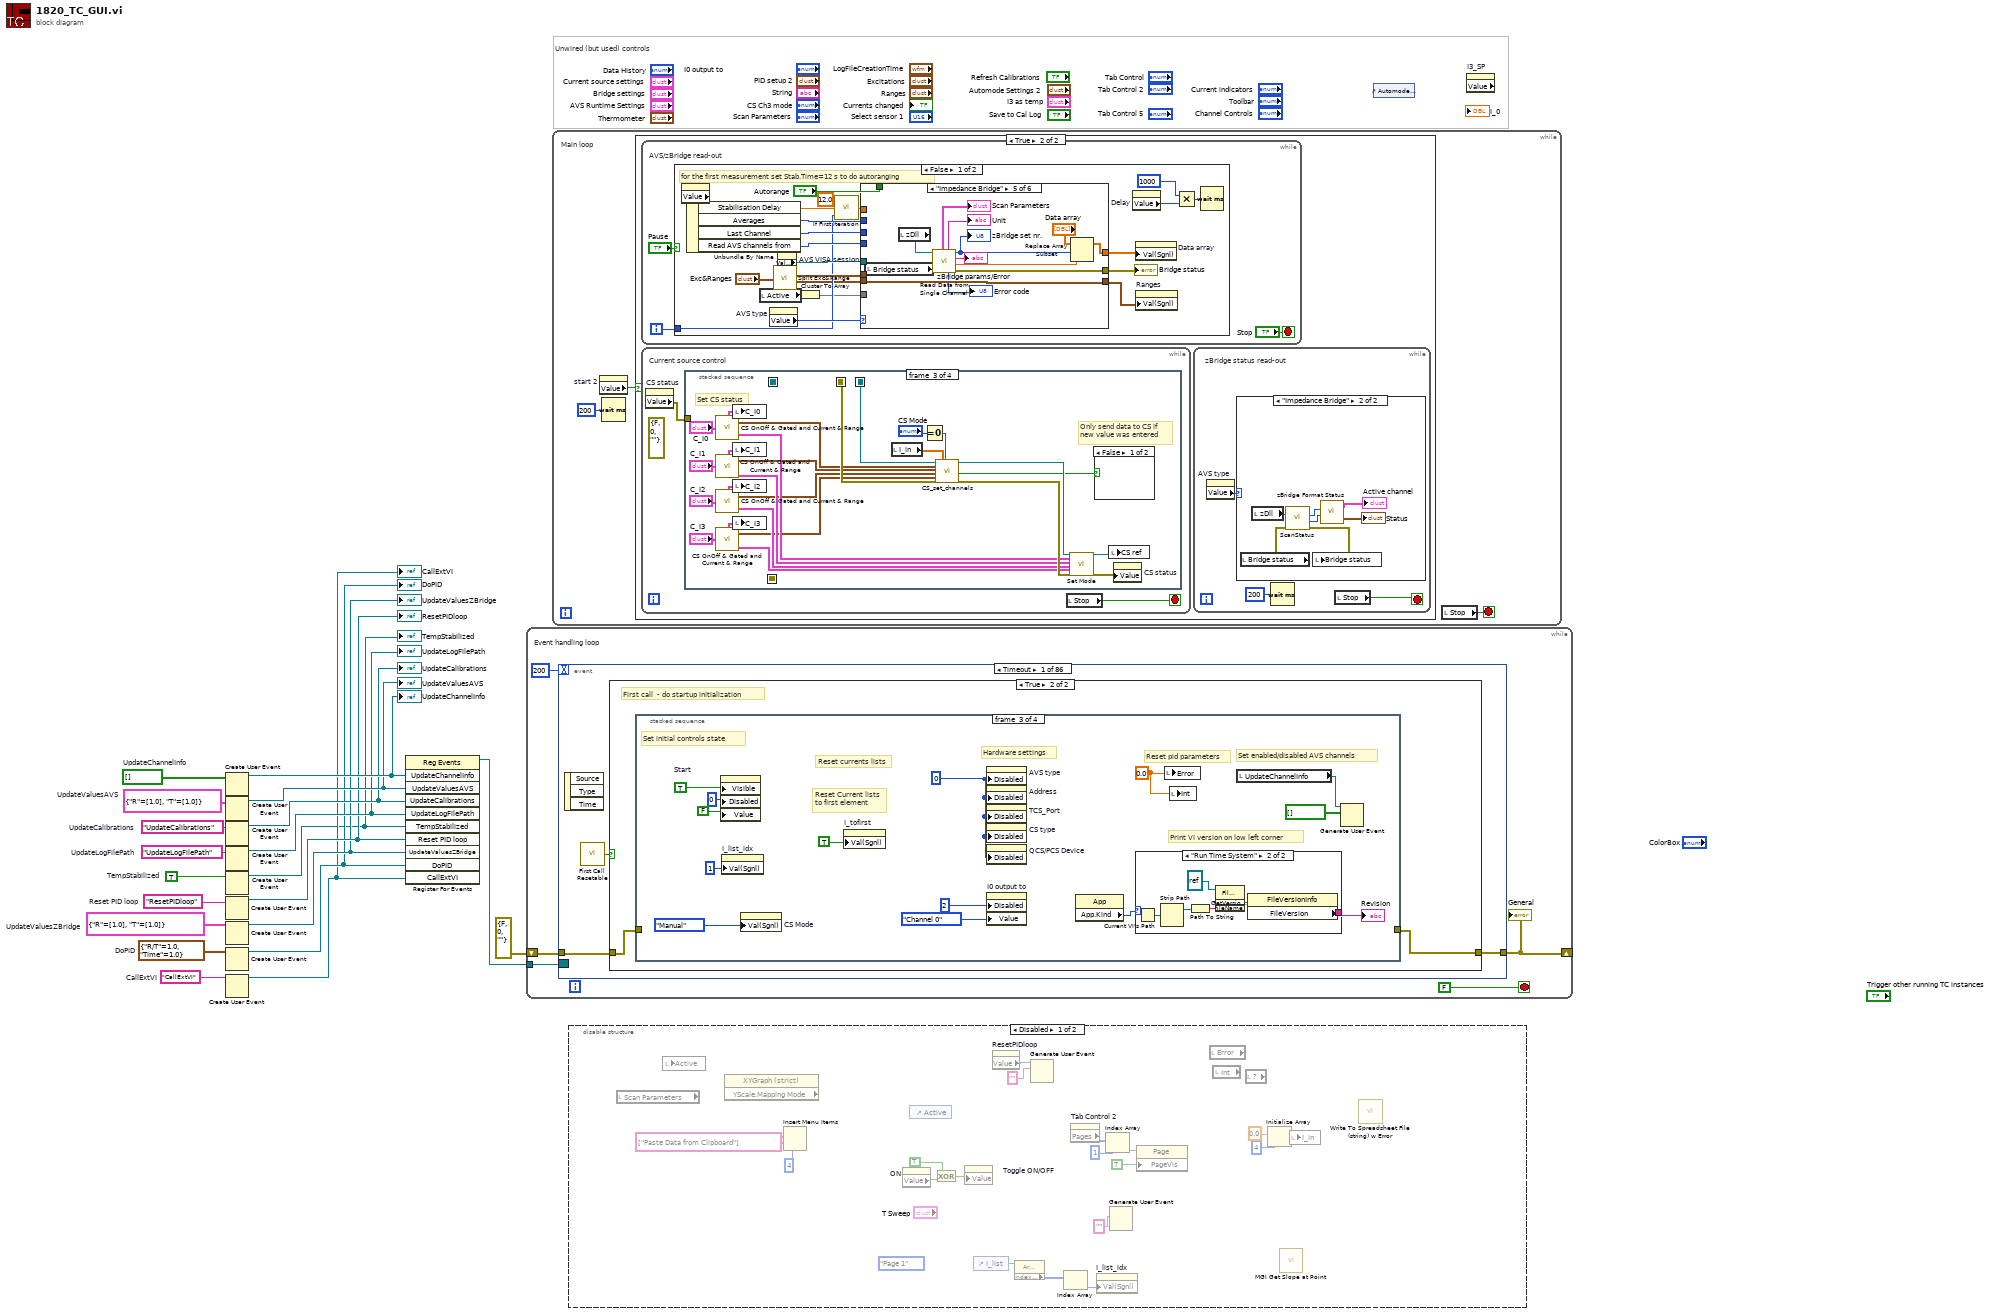
[diagram p0: block diagram]
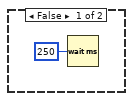
[diagram p3: hidden frame]
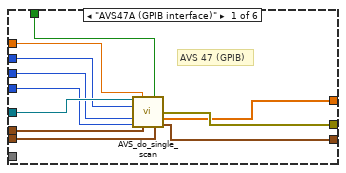
[diagram p5: hidden frame]
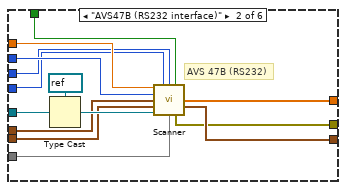
[diagram p6: hidden frame]
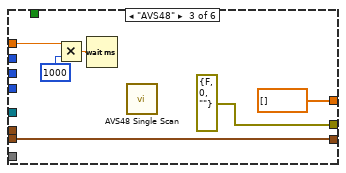
[diagram p7: hidden frame]
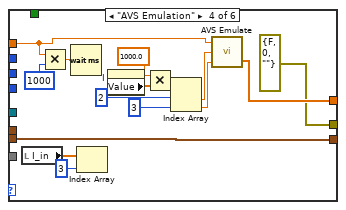
[diagram p8: hidden frame]
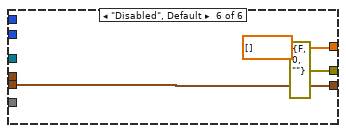
[diagram p9: hidden frame]
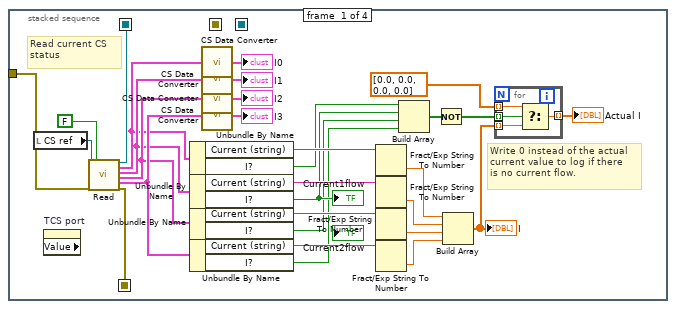
[diagram p11: hidden frame]
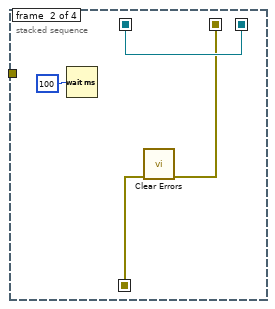
[diagram p12: hidden frame]
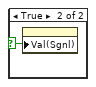
[diagram p13: hidden frame]
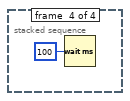
[diagram p14: hidden frame]
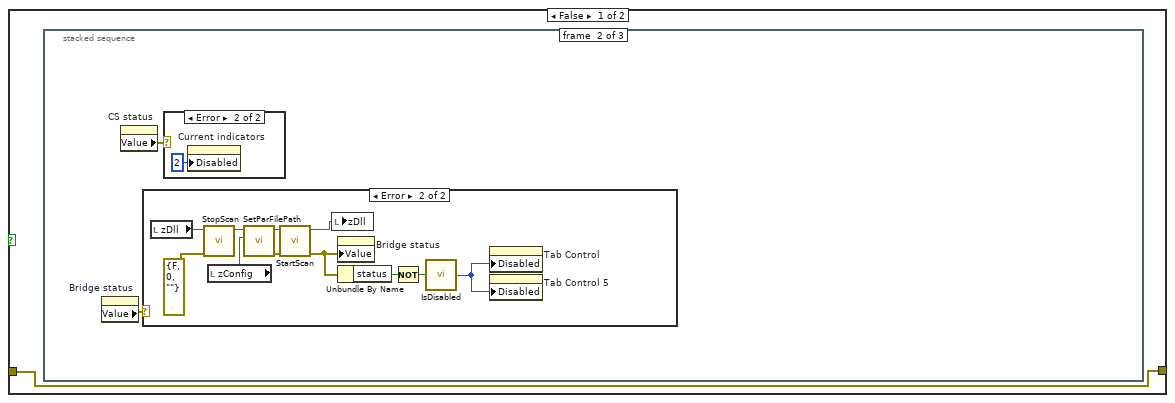
[diagram p15: hidden frame]
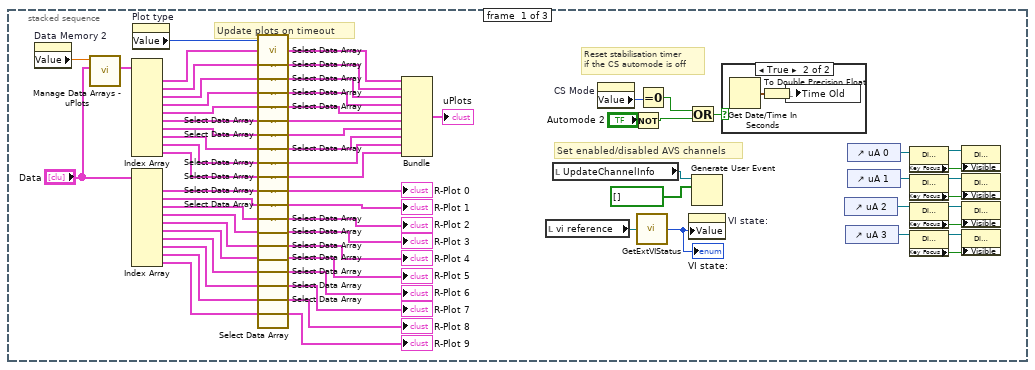
[diagram p16: hidden frame]
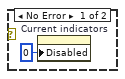
[diagram p18: hidden frame]
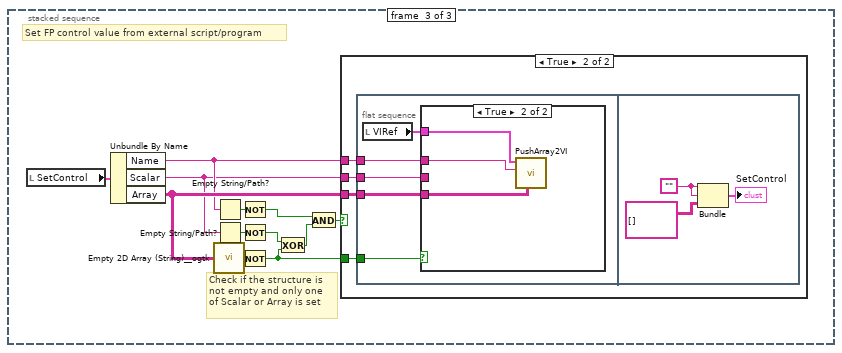
[diagram p20: hidden frame]
diagram:
  w2 = "CallExtVI"  # CallExtVI
  w4 = bool[] []  # UpdateChannelInfo
  w7 = cluster{"R/T":dbl, "Time":dbl} {"R/T"=1.0, "Time"=1.0}  # DoPID
  w8 = cluster{"R":dbl[], "T":dbl[]} {"R"=[1.0], "T"=[1.0]}  # UpdateValuesAVS
  w9 = cluster{"R":dbl[], "T":dbl[]} {"R"=[1.0], "T"=[1.0]}  # UpdateValuesZBridge
  w11 = "ResetPIDloop"  # Reset PID loop
  w13 = TRUE  # TempStabilized
  w14 = "UpdateLogFilePath"  # UpdateLogFilePath
  w17 = "UpdateCalibrations"  # UpdateCalibrations
  # "Unwired (but used) controls"
  n1 = Create User Event(user event datatype=w4) -> (user event=w20:refnum<user-event>)  [unwired: 1 in, 1 out]
  "UpdateChannelInfo" <- w20
  n2 = Create User Event(user event datatype=w8) -> (user event=w19:refnum<user-event>)  [unwired: 1 in, 1 out]
  "UpdateValuesAVS" <- w19
  n3 = Create User Event(user event datatype=w17) -> (user event=w16:refnum<user-event>)  [unwired: 1 in, 1 out]
  "UpdateCalibrations" <- w16
  n4 = Create User Event(user event datatype=w14) -> (user event=w15:refnum<user-event>)  [unwired: 1 in, 1 out]
  "UpdateLogFilePath" <- w15
  n5 = Create User Event ("TempStabilized")(user event datatype=w13) -> (user event=w1:refnum<user-event>)  [unwired: 1 in, 1 out]
  "TempStabilized" <- w1
  n6 = Create User Event(user event datatype=w11) -> (user event=w10:refnum<user-event>)  [unwired: 1 in, 1 out]
  "ResetPIDloop" <- w10
  n7 = Create User Event(user event datatype=w9) -> (user event=w6:refnum<user-event>)  [unwired: 1 in, 1 out]
  "UpdateValuesZBridge" <- w6
  n8 = Create User Event(user event datatype=w7) -> (user event=w5:refnum<user-event>)  [unwired: 1 in, 1 out]
  "DoPID" <- w5
  n9 = Create User Event(user event datatype=w2) -> (user event=w3:refnum<user-event>)  [unwired: 1 in, 1 out]
  "CallExtVI" <- w3
  n10 = register-events(w20, w19, w16, w15, w1, w10, w6, w5, w3) -> (reference out=w18:refnum<event-registration>)  [unwired: 2 in, 1 out]
  n11 = while {
    tunnel: w18 -> [w24]
    shift-right: [w21] -> _
    shift-left: errorcluster {"status"=FALSE, "code"=0, "source"=""} ("error in (no error)") -> [w22]
    stop <- FALSE stop-if-true
    # "Event handling loop"
    n12 = event shown="[0] Timeout" {
      selector: w24 -> [_ _ _ _ _ _ _ _ _ _ _ _ _ _ _ _ _ _ _ _ _ _ _ _ _ _ _ _ _ _ _ _ _ _ _ _ _ _ _ _ _ _ _ _ _ _ _ _ _ _ _ _ _ _ _ _ _ _ _ _ _ _ _ _ _ _ _ _ _ _ _ _ _ _ _ _ _ _ _ _ _ _ _ _ _ _]
      dyn-events: _ -> [_ _ _ _ _ _ _ _ _ _ _ _ _ _ _ _ _ _ _ _ _ _ _ _ _ _ _ _ _ _ _ _ _ _ _ _ _ _ _ _ _ _ _ _ _ _ _ _ _ _ _ _ _ _ _ _ _ _ _ _ _ _ _ _ _ _ _ _ _ _ _ _ _ _ _ _ _ _ _ _ _ _ _ _ _ _]
      timeout: 200 -> [_ _ _ _ _ _ _ _ _ _ _ _ _ _ _ _ _ _ _ _ _ _ _ _ _ _ _ _ _ _ _ _ _ _ _ _ _ _ _ _ _ _ _ _ _ _ _ _ _ _ _ _ _ _ _ _ _ _ _ _ _ _ _ _ _ _ _ _ _ _ _ _ _ _ _ _ _ _ _ _ _ _ _ _ _ _]
      tunnel: w22 -> [w28 _ _ w420 w467 w550 _ _ w717 _ _ w814 w822 _ _ _ _ _ _ _ _ _ _ _ w1111 _ w1118 _ _ _ _ _ _ _ _ _ w1201 _ _ _ _ _ _ _ _ _ _ _ _ _ _ _ _ _ _ _ _ _ _ _ _ _ w1610 w1627 _ _ _ _ _ w1751 _ _ _ _ _ _ _ _ _ _ _ _ _ _ _ _]
      tunnel: [w27 _ _ w423 w466 w547 _ _ w716 _ _ w813 w822 _ _ _ _ _ _ _ _ _ _ _ w1111 _ w1118 _ _ _ _ _ _ _ _ _ w1201 _ _ _ _ _ _ _ _ _ _ _ _ _ _ _ _ _ _ _ _ _ _ _ _ _ w1609 w1626 _ _ _ _ _ w1751 _ _ _ _ _ _ _ _ _ _ _ _ _ _ _ _] -> w21
      event Timeout {
        n13 = event-data() -> ()  [unwired: 1 in, 3 out]
        n14 = call "First Call Resetable.vi"() -> ("First Call?"=w26:bool)
        n15 = case shown="True" w26 {
          tunnel: w28 -> [w29 w144]
          tunnel: [w29 w143] -> w27
          frame False {
            n16 = stacked-sequence {
              frame #0 {
                # "Update plots on timeout"
                # "Set enabled/disabled AVS channels"
                # "Reset stabilisation timer\nif the CS automode is off"
                n17 = property on="Data Memory 2" class="DigNum (strict)"() -> ("Value"=w91:dbl)  [unwired: 2 in, 2 out]
                n18 = call "Manage Data Arrays - uPlots.vi"("Data In"="Data", "Data Memory"=w91) -> ("Data Out"=w46:cluster{"R":dbl[], "T":dbl[], "Time":dbl[]}[])  [unwired: 7 in]
                n19 = Index Array(array=w46) -> (element #1=w61:cluster{"R":dbl[], "T":dbl[], "Time":dbl[]}, element #2=w62:cluster{"R":dbl[], "T":dbl[], "Time":dbl[]}, element #3=w63:cluster{"R":dbl[], "T":dbl[], "Time":dbl[]}, element #4=w64:cluster{"R":dbl[], "T":dbl[], "Time":dbl[]}, element #5=w65:cluster{"R":dbl[], "T":dbl[], "Time":dbl[]}, element #6=w66:cluster{"R":dbl[], "T":dbl[], "Time":dbl[]}, element #7=w67:cluster{"R":dbl[], "T":dbl[], "Time":dbl[]}, element #8=w68:cluster{"R":dbl[], "T":dbl[], "Time":dbl[]}, element #9=w69:cluster{"R":dbl[], "T":dbl[], "Time":dbl[]}, element #10=w70:cluster{"R":dbl[], "T":dbl[], "Time":dbl[]})  [unwired: 10 in]
                n20 = Index Array(array="Data") -> (element #1=w90:cluster{"R":dbl[], "T":dbl[], "Time":dbl[]}, element #2=w89:cluster{"R":dbl[], "T":dbl[], "Time":dbl[]}, element #3=w88:cluster{"R":dbl[], "T":dbl[], "Time":dbl[]}, element #4=w87:cluster{"R":dbl[], "T":dbl[], "Time":dbl[]}, element #5=w86:cluster{"R":dbl[], "T":dbl[], "Time":dbl[]}, element #6=w85:cluster{"R":dbl[], "T":dbl[], "Time":dbl[]}, element #7=w84:cluster{"R":dbl[], "T":dbl[], "Time":dbl[]}, element #8=w83:cluster{"R":dbl[], "T":dbl[], "Time":dbl[]}, element #9=w82:cluster{"R":dbl[], "T":dbl[], "Time":dbl[]}, element #10=w81:cluster{"R":dbl[], "T":dbl[], "Time":dbl[]})  [unwired: 10 in]
                n21 = property on="Plot type" class="Enum (strict)"() -> ("Value"=w49:enum16{"R vs Time", "T vs Time"})  [unwired: 2 in, 2 out]
                n22 = call "Select Data Array.vi"("Cluster 2"=w61, "Value"=w49) -> ("Cluster"=w71:cluster{"Time":dbl[], "T":dbl[]})
                n23 = call "Select Data Array.vi"("Cluster 2"=w62, "Value"=w49) -> ("Cluster"=w72:cluster{"Time":dbl[], "T":dbl[]})
                n24 = call "Select Data Array.vi"("Cluster 2"=w63, "Value"=w49) -> ("Cluster"=w73:cluster{"Time":dbl[], "T":dbl[]})
                n25 = call "Select Data Array.vi"("Cluster 2"=w64, "Value"=w49) -> ("Cluster"=w74:cluster{"Time":dbl[], "T":dbl[]})
                n26 = call "Select Data Array.vi"("Cluster 2"=w65, "Value"=w49) -> ("Cluster"=w80:cluster{"Time":dbl[], "T":dbl[]})
                n27 = call "Select Data Array.vi"("Cluster 2"=w66, "Value"=w49) -> ("Cluster"=w75:cluster{"Time":dbl[], "T":dbl[]})
                n28 = call "Select Data Array.vi"("Cluster 2"=w67, "Value"=w49) -> ("Cluster"=w76:cluster{"Time":dbl[], "T":dbl[]})
                n29 = call "Select Data Array.vi"("Cluster 2"=w68, "Value"=w49) -> ("Cluster"=w77:cluster{"Time":dbl[], "T":dbl[]})
                n30 = call "Select Data Array.vi"("Cluster 2"=w69, "Value"=w49) -> ("Cluster"=w78:cluster{"Time":dbl[], "T":dbl[]})
                n31 = call "Select Data Array.vi"("Cluster 2"=w70, "Value"=w49) -> ("Cluster"=w79:cluster{"Time":dbl[], "T":dbl[]})
                n32 = call "Select Data Array.vi"("Cluster 2"=w90, "Value"=w49) -> ("Cluster"=→"R-Plot 0":cluster{"Time":dbl[], "T":dbl[]})
                n33 = call "Select Data Array.vi"("Cluster 2"=w89, "Value"=w49) -> ("Cluster"=→"R-Plot 1":cluster{"Time":dbl[], "T":dbl[]})
                n34 = call "Select Data Array.vi"("Cluster 2"=w88, "Value"=w49) -> ("Cluster"=→"R-Plot 2":cluster{"Time":dbl[], "T":dbl[]})
                n35 = call "Select Data Array.vi"("Cluster 2"=w87, "Value"=w49) -> ("Cluster"=→"R-Plot 3":cluster{"Time":dbl[], "T":dbl[]})
                n36 = call "Select Data Array.vi"("Cluster 2"=w86, "Value"=w49) -> ("Cluster"=→"R-Plot 4":cluster{"Time":dbl[], "T":dbl[]})
                n37 = call "Select Data Array.vi"("Cluster 2"=w85, "Value"=w49) -> ("Cluster"=→"R-Plot 5":cluster{"Time":dbl[], "T":dbl[]})
                n38 = call "Select Data Array.vi"("Cluster 2"=w84, "Value"=w49) -> ("Cluster"=→"R-Plot 6":cluster{"Time":dbl[], "T":dbl[]})
                n39 = call "Select Data Array.vi"("Cluster 2"=w83, "Value"=w49) -> ("Cluster"=→"R-Plot 7":cluster{"Time":dbl[], "T":dbl[]})
                n40 = call "Select Data Array.vi"("Cluster 2"=w82, "Value"=w49) -> ("Cluster"=→"R-Plot 8":cluster{"Time":dbl[], "T":dbl[]})
                n41 = call "Select Data Array.vi"("Cluster 2"=w81, "Value"=w49) -> ("Cluster"=→"R-Plot 9":cluster{"Time":dbl[], "T":dbl[]})
                n42 = Bundle("Cluster"=w71, "Cluster"=w72, "Cluster"=w73, "Cluster"=w74, "Cluster"=w80, "Cluster"=w75, "Cluster"=w76, "Cluster"=w77, "Cluster"=w78, "Cluster"=w79) -> (→"uPlots":T38)  [unwired: 1 in]
                n43 = local read "vi reference"() -> (w45:refnum<vi>)
                n44 = local read "UpdateChannelInfo"() -> (w44:refnum<user-event>)
                n45 = property on="CS Mode" class="Enum (strict)"() -> ("Value"=w94:enum16{"Manual", "Automatic"})  [unwired: 2 in, 2 out]
                n46 = Not(x="Automode 2") -> (.not. x?=w93:bool)
                n47 = call "GetExtVIStatus.vi"("vi reference in"=w45) -> ("Exec.State"=w43:T30)  [unwired: 2 out]
                "VI state:" <- w43
                n48 = Equal To 0?(x=w94) -> (x = 0?=w42:bool)
                n49 = Or(x=w42, y=w93) -> (x .or. y?=w92:bool)
                n50 = property on="VI state:" class="Enum (strict)"("Value"=w43) -> ()  [unwired: 2 in, 2 out]
                n51 = Generate User Event(user event=w44, event data cluster=bool[] [] ("event data")) -> ()  [unwired: 2 in, 2 out]
                n52 = case shown="True" w92 {
                  frame False {
                  }
                  frame True {
                    n53 = Get Date/Time In Seconds() -> (seconds since 1Jan1904=w96:timestamp)
                    n54 = To Double Precision Float(number=w96) -> (double precision float=w97:dbl)
                    n55 = local write "Time Old"(w97) -> ()
                  }
                }
                n56 = control-ref of="uA 2"() -> (w30:refnum<vi>)
                n57 = control-ref of="uA 3"() -> (w31:refnum<vi>)
                n58 = control-ref of="uA 0"() -> (w41:refnum<vi>)
                n59 = control-ref of="uA 1"() -> (w37:refnum<vi>)
                n60 = property class="DigNum (strict)"(reference=w41) -> (reference out=w40:refnum<vi>, "Key Focus"=w39:bool)  [unwired: 1 in, 1 out]
                n61 = property class="DigNum (strict)"(reference=w37) -> (reference out=w38:refnum<vi>, "Key Focus"=w36:bool)  [unwired: 1 in, 1 out]
                n62 = property class="DigNum (strict)"(reference=w30) -> (reference out=w32:refnum<vi>, "Key Focus"=w33:bool)  [unwired: 1 in, 1 out]
                n63 = property class="DigNum (strict)"(reference=w31) -> (reference out=w34:refnum<vi>, "Key Focus"=w35:bool)  [unwired: 1 in, 1 out]
                n64 = property class="DigNum (strict)"(reference=w40, "Visible"=w39) -> ()  [unwired: 1 in, 2 out]
                n65 = property class="DigNum (strict)"(reference=w38, "Visible"=w36) -> ()  [unwired: 1 in, 2 out]
                n66 = property class="DigNum (strict)"(reference=w32, "Visible"=w33) -> ()  [unwired: 1 in, 2 out]
                n67 = property class="DigNum (strict)"(reference=w34, "Visible"=w35) -> ()  [unwired: 1 in, 2 out]
              }
              frame #1 {
                n68 = property on="Bridge status" class="Clust (strict)"() -> ("Value"=w99:errorcluster)  [unwired: 2 in, 2 out]
                n69 = property on="CS status" class="Clust (strict)"() -> ("Value"=w98:errorcluster)  [unwired: 2 in, 2 out]
                n70 = case shown="Error" w99 {
                  frame No Error {
                  }
                  frame Error {
                    n71 = local read "zDll"() -> (w112:path)
                    n72 = call "StopScan.vi"("error in (no error)"=errorcluster {"status"=FALSE, "code"=0, "source"=""}, "path in"=w112) -> ("path out"=w108:path)  [unwired: 8 in, 1 out]
                    n73 = local read "zConfig"() -> (w111:path)
                    n74 = call "SetParFilePath.vi"("path"=w111, "zDll"=w108) -> ("error out"=w110:errorcluster, "zDll out"=w109:path)  [unwired: 8 in]
                    n75 = call "StartScan.vi"("error in (no error)"=w110, "path in"=w109) -> ("error out"=w105:errorcluster, "path out"=w106:path)  [unwired: 8 in]
                    n76 = local write "zDll"(w106) -> ()
                    n77 = property on="Bridge status" class="Clust (strict)"("Value"=w105) -> ()  [unwired: 2 in, 2 out]
                    n78 = Unbundle By Name(w105) -> ("status"=w103:bool)
                    n79 = Not(x=w103) -> (.not. x?=w104:bool)
                    n80 = call "IsDisabled.vi"("Enabled?"=w104) -> ("Numeric"=w102:i16)
                    n81 = property on="Tab Control" class="TabCtl (strict)"("Disabled"=w102) -> ()  [unwired: 2 in, 2 out]
                    n82 = property on="Tab Control 5" class="TabCtl (strict)"("Disabled"=w102) -> ()  [unwired: 2 in, 2 out]
                  }
                }
                n83 = case shown="Error" w98 {
                  frame No Error {
                    n84 = property on="Current indicators" class="TabCtl (strict)"("Disabled"=u8 0) -> ()  [unwired: 2 in, 2 out]
                  }
                  frame Error {
                    n85 = property on="Current indicators" class="TabCtl (strict)"("Disabled"=u8 2) -> ()  [unwired: 2 in, 2 out]
                  }
                }
              }
              frame #2 {
                # "Check if the structure is \nnot empty and only one\nof Scalar or Array is set"
                # "Set FP control value from external script/program"
                n86 = local read "SetControl"() -> (w113:T1)
                n87 = Unbundle By Name(w113) -> ("Name"=w115:string, "Scalar"=w114:string, "Array"=w123:string[][])
                n88 = call "Empty 2D Array (String)__ogtk.vi"("Array"=w123) -> ("Empty Array?"=w120:bool)  [unwired: 8 in]
                n89 = Empty String/Path?(string/path=w115) -> (empty?=w119:bool)
                n90 = Empty String/Path?(string/path=w114) -> (empty?=w118:bool)
                n91 = Not(x=w119) -> (.not. x?=w117:bool)
                n92 = Not(x=w118) -> (.not. x?=w121:bool)
                n93 = Not(x=w120) -> (.not. x?=w124:bool)
                n94 = Exclusive Or(1:w124, 2:w121) -> (0:w122:bool)
                n95 = And(x=w117, y=w122) -> (x .and. y?=w116:bool)
                n96 = case shown="True" w116 {
                  tunnel: w115 -> [_ w128]
                  tunnel: w114 -> [_ w127]
                  tunnel: w123 -> [_ w126]
                  tunnel: w124 -> [_ w125]
                  frame False {
                  }
                  frame True {
                    n97 = flat-sequence {
                      tunnel: w128 -> [w132]
                      tunnel: w127 -> [w131]
                      tunnel: w126 -> [w129]
                      tunnel: w125 -> [w130]
                      frame #0 {
                        n98 = local read "VIRef"() -> (w133:T2)
                        n99 = case shown="True" w130 {
                          tunnel: w133 -> [w136 w139]
                          tunnel: w132 -> [w135 w138]
                          tunnel: w131 -> [w134 _]
                          tunnel: w129 -> [_ w137]
                          frame False {
                            n100 = call "Push2VI.vi"("New Value"=w134, "element"=w135, "VIRef"=w136) -> ()  [unwired: 8 in, 1 out]
                          }
                          frame True {
                            n101 = call "PushArray2VI.vi"("Str"=w137, "element"=w138, "VIRef"=w139) -> ()  [unwired: 8 in, 1 out]
                          }
                        }
                      }
                      frame #1 {
                        w141 = ""
                        n102 = Bundle(w141, w141, "Array"=string[][] []) -> (→"SetControl":cluster{string, string, "Array":string[][]})  [unwired: 1 in]
                      }
                    }
                  }
                }
              }
            }
          }
          frame True {
            # "First call  - do startup initialization"
            n103 = stacked-sequence {
              tunnel: w144 -> [_ w169 _ _]
              tunnel: [_ w160 _ _] -> w143
              frame #0 {
                w157 = u8 0 ("Disabled")
                n104 = property on="Tab Control 5" class="TabCtl (strict)"("Disabled"=w157) -> ()  [unwired: 2 in, 2 out]
                n105 = property on="Toolbar" class="TabCtl (strict)"("Disabled"=w157) -> ()  [unwired: 2 in, 2 out]
                n106 = property on="Tab Control" class="TabCtl (strict)"("Disabled"=w157) -> ()  [unwired: 2 in, 2 out]
                n107 = property on="Current indicators" class="TabCtl (strict)"("Disabled"=w157) -> ()  [unwired: 2 in, 2 out]
                n108 = property on="Tab Control 2" class="TabCtl (strict)"("Disabled"=w157) -> ()  [unwired: 2 in, 2 out]
                n109 = property on="String" class="Str"("Visible"=FALSE) -> ()  [unwired: 2 in, 2 out]
                n110 = property on="I_0" class="DigNum (strict)"("Value"=0.0 ("I3")) -> ()  [unwired: 2 in, 2 out]
                n111 = call "Current VIs Reference__ogtk.vi"() -> ("Current VI's reference"=w147:refnum<vi>)  [unwired: 5 in]
                n112 = call "Current VIs Parent Directory__ogtk.vi"("Relative path (.)"=path "Calibrations" ("Library Path")) -> ("Parent Directory (+ Relative)"=w153:path)  [unwired: 4 in]
                n113 = call "Current VIs Parent Directory__ogtk.vi"("Relative path (.)"=path "data/Temp Control.lvlib" ("Library Path")) -> ("Parent Directory (+ Relative)"=w155:path)  [unwired: 4 in]
                n114 = call "Current VIs Parent Directory__ogtk.vi"("Relative path (.)"=path "data/ImpBridgeDll.dll" ("Library Path")) -> ("Parent Directory (+ Relative)"=→"zDll":path)  [unwired: 4 in]
                n115 = call "Current VIs Parent Directory__ogtk.vi"("Relative path (.)"=path "data" ("Library Path")) -> ("Parent Directory (+ Relative)"=→"zConfig":path)  [unwired: 4 in]
                n116 = call "GetFrontPanelControls.vi"("Ref to VI"=w147) -> ("VIRef"=w146:T2)  [unwired: 9 in, 1 out]
                "VIRef" <- w146
                n117 = property on="AVS_CalFolder" class="Path"("Value"=w153) -> ()  [unwired: 2 in, 2 out]
                n118 = invoke class="App" method="Library.Deploy Library"("libPath"=w155) -> ()  [unwired: 4 in, 5 out]
                n119 = Unbundle By Name(w146) -> ("Full Name"=→"ControlNames":string[])
                n120 = property on="Minimize" class="Bool (strict)"("Val(Sgnl)"=FALSE ("Value (Signaling)")) -> ()  [unwired: 2 in, 2 out]
              }
              frame #1 {
                # "Read settings from registry"
                n121 = flat-sequence {
                  tunnel: [w184] -> w168
                  tunnel: w169 -> [w183]
                  tunnel: [w181] -> w167
                  tunnel: w168 -> [w189]
                  tunnel: [w189] -> w166
                  tunnel: [w187] -> w165
                  tunnel: w167 -> [w187]
                  tunnel: [w194] -> w164
                  tunnel: w166 -> [w193]
                  tunnel: [w191] -> w163
                  tunnel: w165 -> [w191]
                  tunnel: w164 -> [w200]
                  tunnel: [w200] -> w162
                  tunnel: [w198] -> w161
                  tunnel: w163 -> [w198]
                  tunnel: w162 -> [w203]
                  tunnel: [w202] -> w160
                  tunnel: w161 -> [w201]
                  frame #0 {
                    n122 = call "Current VIs Parent Directory__ogtk.vi"("Relative path (.)"=path "data/config.ini") -> ("Parent Directory (+ Relative)"=w181:path)  [unwired: 4 in]
                    n123 = control-ref of="Active"() -> (w173:refnum<vi>)
                    n124 = control-ref of="Automode Settings 2"() -> (w171:refnum<vi>)
                    n125 = control-ref of="Current source settings"() -> (w174:refnum<vi>)
                    n126 = control-ref of="Bridge settings"() -> (w185:refnum<vi>)
                    n127 = control-ref of="AVS Runtime Settings"() -> (w180:refnum<vi>)
                    n128 = control-ref of="I3 as temp"() -> (w172:refnum<vi>)
                    n129 = control-ref of="Data logging"() -> (w179:refnum<vi>)
                    n130 = control-ref of="PID setup 2"() -> (w178:refnum<vi>)
                    n131 = control-ref of="CS Names"() -> (w177:refnum<vi>)
                    n132 = control-ref of="CurCalibrations"() -> (w175:refnum<vi>)
                    n133 = control-ref of="AVS names"() -> (w176:refnum<vi>)
                    n134 = Build Array(w173, w174, w185, w180, w179, w178, w177, w176, w175, w172, w171) -> (w186:refnum<vi>[])
                    n135 = call "Save Load Settings to File by Ref with path.vi"("Array of Cluster References"=w186, "Action"=enum8{"Load", "Save"}."Load", "error in (no error)"=w183, "configuration file path"=w181) -> ("error out"=w184:errorcluster)  [unwired: 5 in]
                  }
                  frame #1 {
                    n136 = Wait (ms)(milliseconds to wait=250) -> ()  [unwired: 1 out]
                  }
                  frame #2 {
                    n137 = control-ref of="Thermometer"() -> (w192:refnum<vi>)
                    n138 = control-ref of="CurCalibrations"() -> (w190:refnum<vi>)
                    n139 = control-ref of="CurCalibrations"() -> ()  [unwired: 1 out]
                    n140 = control-ref of="AVS_CalFolder"() -> (w196:refnum<vi>)
                    n141 = control-ref of="Select sensor 1"() -> (w197:refnum<vi>)
                    n142 = control-ref of="Select sensor 1"() -> (w195:refnum<vi>)
                    n143 = call "ReloadCalibrations.vi"("error in (no error)"=w193, "Quick convert sensors"=w195, "CurCalibrations"=w190, "Calibration files path"=w196, "Channel1 sensors"=w197, "Channels list"=w192) -> ("error out"=w194:errorcluster)  [unwired: 1 in]
                  }
                  frame #3 {
                    n144 = Wait (ms)(milliseconds to wait=250) -> ()  [unwired: 1 out]
                  }
                  frame #4 {
                    n145 = disable-structure shown="Enabled" {
                      disable-tunnel: w203 -> [w206 w213]
                      disable-tunnel: [w205 w211] -> w202
                      disable-tunnel: w201 -> [w204 _]
                      frame Disabled {
                        (unwired) "SOFTWARE\\Leiden Cryogenics\\TC" ("subkey 2")
                        (unwired) T39."HKEY_CURRENT_USER" ("root key (HKEY_LOCAL_MACHINE) 2")
                        n146 = control-ref of="Thermometer"() -> (w208:refnum<vi>)
                        n147 = Build Array(w208) -> (w207:refnum<vi>[])
                        n148 = call "Save Load Settings to File by Ref with path.vi"("Array of Cluster References"=w207, "Action"=enum8{"Load", "Save"}."Load", "error in (no error)"=w206, "configuration file path"=w204) -> ("error out"=w205:errorcluster)  [unwired: 5 in]
                      }
                      frame Enabled {
                        n149 = property on="UpdateCalibrations" class="TypRef (strict)"(error in=w213) -> (error out=w212:errorcluster, "Value"=w214:refnum<user-event>)  [unwired: 1 in, 1 out]
                        n150 = Generate User Event(user event=w214, event data cluster="" ("event data"), error in=w212) -> (error out=w211:errorcluster)  [unwired: 1 in, 1 out]
                      }
                    }
                  }
                }
              }
              frame #2 {
                w224 = 0.0 ("T_error")
                w225 = u8 0 ("Disabled")
                # "Set enabled/disabled AVS channels"
                # "Print VI version on low left corner"
                # "Reset Current lists\nto first element"
                # "Reset pid parameters"
                # "Hardware settings"
                # "Reset currents lists"
                # "Set initial controls state"
                n151 = property on="Start" class="Bool (strict)"("Visible"=TRUE, "Disabled"=u8 0, "Value"=FALSE ("start")) -> ()  [unwired: 2 in, 2 out]
                n152 = property on="I_list_idx" class="DigNum (strict)"("Val(Sgnl)"=1 ("Value (Signaling)")) -> ()  [unwired: 2 in, 2 out]
                n153 = property on="CS Mode" class="Enum (strict)"("Val(Sgnl)"=enum16{"Manual", "Automatic"}."Manual" ("Value (Signaling)")) -> ()  [unwired: 2 in, 2 out]
                n154 = property on="I_tofirst" class="Bool (strict)"("Val(Sgnl)"=TRUE ("Value (Signaling)")) -> ()  [unwired: 2 in, 2 out]
                n155 = property on="AVS type" class="Enum (strict)"("Disabled"=w225) -> ()  [unwired: 2 in, 2 out]
                n156 = property on="Address" class="VISAName"("Disabled"=w225) -> ()  [unwired: 2 in, 2 out]
                n157 = property on="TCS_Port" class="VISAName"("Disabled"=w225) -> ()  [unwired: 2 in, 2 out]
                n158 = property on="CS type" class="Enum (strict)"("Disabled"=w225) -> ()  [unwired: 2 in, 2 out]
                n159 = property on="QCS/PCS Device" class="DigNum (strict)"("Disabled"=w225) -> ()  [unwired: 2 in, 2 out]
                n160 = property on="I0 output to" class="Enum (strict)"("Disabled"=u8 2, "Value"=T29."Channel 0" ("Map Channel 0 to")) -> ()  [unwired: 2 in, 2 out]
                n161 = property class="App"() -> ("App.Kind"=w220:T40)  [unwired: 2 in, 2 out]
                n162 = case shown="\"Run Time System\"" w220 {
                  tunnel: [w230 w241] -> w221
                  frame "invalid app kind", Default {
                    n163 = control-ref of="This VI"() -> (w237:refnum<vi>)
                    n164 = property class="VI"(reference=w237) -> ("Hist.Revision"=w236:u32)  [unwired: 1 in, 2 out]
                    n165 = Divide(x=w236, y=1000.0 ("x")) -> (x/y=w232:dbl)
                    n166 = Number To Fractional String(use system decimal point (T)=FALSE, number=w232, precision (6)=i16 2) -> (F-format string=w231:string)  [unwired: 1 in]
                    n167 = Concatenate Strings("" ("string"), w231) -> (w230:string)
                  }
                  frame "Run Time System" {
                    n168 = Current VI's Path() -> (path=w243:path)
                    n169 = Strip Path(path=w243) -> (stripped path=w242:path)  [unwired: 1 out]
                    n170 = Path To String(path=w242) -> (string=w240:string)
                    n171 = invoke class="FileVersionInfo" method="GetVersionInfo"(reference=refnum<k24> refnum (".NET object"), "fileName"=w240) -> ("GetVersionInfo"=w239:refnum<k24>)  [unwired: 2 in, 3 out]
                    n172 = property class="FileVersionInfo"(reference=w239) -> ("FileVersion"=w241:string)  [unwired: 1 in, 2 out]
                  }
                }
                "Revision" <- w221
                n173 = local write "Error"(w224) -> ()
                n174 = local write "Int"(w224) -> ()
                n175 = local read "UpdateChannelInfo"() -> (w219:refnum<user-event>)
                n176 = Generate User Event(user event=w219, event data cluster=bool[] [] ("event data")) -> ()  [unwired: 2 in, 2 out]
              }
              frame #3 {
                n177 = call <userlib>:"GetLocalComputerName.vi"() -> ("Name"=→"Name":string)  [unwired: 10 in, 1 out]
              }
            }
          }
        }
      }
      event "Start": Value Change {
        # "\"Start\" button clicked -> start measuring"
        n178 = event-data() -> ()  [unwired: 1 in, 6 out]
        n179 = stacked-sequence {
          frame #0 {
            n180 = property on="Run description" class="Str"() -> ("Value"=w247:string)  [unwired: 2 in, 2 out]
            n181 = property on="Ask on start?" class="Bool (strict)"() -> ("Value"=w246:bool)  [unwired: 2 in, 2 out]
            n182 = Not(x=w246) -> (.not. x?=w245:bool)
            n183 = call "Run Reference DLG.vi"("Enable"=w246, "Run Reference"=w247, "Dont' ask again"=w245) -> ("Dont' ask again"=w249:bool, "Run Reference"=w250:string, "OK"=w251:bool)  [unwired: 13 in, 1 out]
            n184 = Not(x=w249) -> (.not. x?=w248:bool)
            n185 = case shown="True" w251 {
              tunnel: w250 -> [_ w253]
              tunnel: w248 -> [_ w252]
              frame False {
              }
              frame True {
                n186 = property on="Run description" class="Str"("Val(Sgnl)"=w253) -> ()  [unwired: 2 in, 2 out]
                n187 = property on="Ask on start?" class="Bool (strict)"("Val(Sgnl)"=w252) -> ()  [unwired: 2 in, 2 out]
              }
            }
          }
          frame #1 {
            (unwired) T39."HKEY_CURRENT_USER" ("root key (HKEY_LOCAL_MACHINE) 2")
            # "Save new settings to config file"
            n188 = control-ref of="Active"() -> (w258:refnum<vi>)
            n189 = control-ref of="I3 as temp"() -> (w257:refnum<vi>)
            n190 = control-ref of="Automode Settings 2"() -> (w256:refnum<vi>)
            n191 = control-ref of="Automode Settings 2"() -> (w255:refnum<vi>)
            n192 = control-ref of="CS Names"() -> (w263:refnum<vi>)
            n193 = control-ref of="AVS names"() -> (w262:refnum<vi>)
            n194 = control-ref of="CurCalibrations"() -> (w259:refnum<vi>)
            n195 = control-ref of="Bridge settings"() -> (w268:refnum<vi>)
            n196 = control-ref of="AVS Runtime Settings"() -> (w269:refnum<vi>)
            n197 = control-ref of="Current source settings"() -> (w267:refnum<vi>)
            n198 = control-ref of="Thermometer"() -> (w270:refnum<vi>)
            n199 = control-ref of="PID setup 2"() -> (w271:refnum<vi>)
            n200 = control-ref of="Data logging"() -> (w266:refnum<vi>)
            n201 = Build Array(w258, w268, w269, w267, w266, w270, w271, w263, w262, w259, w257, w256, w255) -> (w265:refnum<vi>[])
            n202 = call "Current VIs Parent Directory__ogtk.vi"("Relative path (.)"=path "data/config.ini") -> ("Parent Directory (+ Relative)"=w260:path)  [unwired: 4 in]
            n203 = call "Save Load Settings to File by Ref with path.vi"("Array of Cluster References"=w265, "subkey"="SOFTWARE\\Leiden Cryogenics\\TC" ("subkey 2"), "Action"=enum8{"Load", "Save"}."Save", "configuration file path"=w260) -> ()  [unwired: 5 in, 1 out]
          }
          frame #2 {
            w284 = u8 2 ("Disabled")
            # "Reset stop button"
            # "Hide Disable Start button"
            # "Load external calibration VI"
            # "Set controls\nInitialize data for run"
            # "Lock hardware settings"
            n204 = property on="AVS type" class="Enum (strict)"("Disabled"=w284) -> ()  [unwired: 2 in, 2 out]
            n205 = property on="Address" class="VISAName"("Disabled"=w284) -> ()  [unwired: 2 in, 2 out]
            n206 = property on="AVS_SPort" class="VISAName"("Disabled"=w284) -> ()  [unwired: 2 in, 2 out]
            n207 = property on="TCS_Port" class="VISAName"("Disabled"=w284) -> ()  [unwired: 2 in, 2 out]
            n208 = property on="CS type" class="Enum (strict)"("Disabled"=w284) -> ()  [unwired: 2 in, 2 out]
            n209 = property on="QCS/PCS Device" class="DigNum (strict)"("Disabled"=w284) -> ()  [unwired: 2 in, 2 out]
            n210 = property on="I0 output to" class="Enum (strict)"("Disabled"=u8 0) -> ()  [unwired: 2 in, 2 out]
            n211 = Get Date/Time In Seconds() -> (seconds since 1Jan1904=w283:timestamp)
            n212 = To Double Precision Float(number=w283) -> (double precision float=w282:dbl)
            n213 = local write "Time Old"(w282) -> ()
            n214 = property on="External VI path" class="Path"() -> ("Value"=w281:path)  [unwired: 2 in, 2 out]
            n215 = vi-ref "OnTempStabilizedRef.vi"() -> (w280:refnum<vi>)
            n216 = Open VI Reference(type specifier VI Refnum (for type only)=w280, vi path=w281) -> (vi reference=→"vi reference":refnum<vi>)  [unwired: 4 in, 1 out]
            n217 = local write "VI called?"(FALSE ("VI called?")) -> ()
            n218 = property on="Start" class="Bool (strict)"("Visible"=TRUE, "Disabled"=u8 2) -> ()  [unwired: 2 in, 2 out]
            n219 = Initialize Array(cluster{"R":dbl[], "T":dbl[], "Time":dbl[]} {"R"=[], "T"=[], "Time"=[]}, 10 ("dimension size")) -> (w275:cluster{"R":dbl[], "T":dbl[], "Time":dbl[]}[])
            n220 = disable-structure shown="Enabled" {
              frame Enabled {
                n221 = property on="Stop" class="Bool (strict)"("Value"=FALSE ("MainStopButton")) -> ()  [unwired: 2 in, 2 out]
              }
              frame Disabled {
              }
            }
            n222 = local write "Data"(w275) -> ()
          }
          frame #3 {
            # "Initialize CS"
            n223 = local read "CS ref"() -> (w296:refnum<class "CS.lvclass">)
            n224 = call-dynamic "Initialize.vi"("CS in"=w296, "HW Address"="HW Address", "error in (no error)"=T33 {"error"=FALSE, "code"=0, "source"=""} ("error in")) -> ("CS out"=w289:refnum<class "CS.lvclass">, "Instrument ID"=→"ID":string, "error out"=w288:errorcluster)  [unwired: 10 in]
            n225 = call-dynamic "Get Currents & Ranges.vi"("CS.lvclass in"=w289, "error in (no error)"=w288) -> ("CS.lvclass out"=w297:refnum<class "CS.lvclass">, "I0"=w298:cluster{"Value":dbl, "Range":dbl}, "I1"=w290:cluster{"Value":dbl, "Range":dbl}, "I2"=w291:cluster{"Value":dbl, "Range":dbl}, "I3"=w292:cluster{"Value":dbl, "Range":dbl}, "error out"=w294:errorcluster)  [unwired: 12 in]
            "CS status" <- w294
            n226 = local write "CS ref"(w297) -> ()
            n227 = Unbundle By Name(w294) -> ("status"=w286:bool)
            n228 = case shown="False" w286 {
              tunnel: w290 -> [w310 _]
              tunnel: w291 -> [w309 _]
              tunnel: w292 -> [w308 _]
              tunnel: w298 -> [w302 _]
              frame False {
                n229 = Unbundle By Name(w302) -> ("Value"=w301:dbl, "Range"=w300:dbl)
                n230 = Unbundle By Name(w310) -> ("Value"=w307:dbl, "Range"=w306:dbl)
                n231 = Unbundle By Name(w309) -> ("Value"=w305:dbl, "Range"=w304:dbl)
                n232 = Unbundle By Name(w308) -> ("Value"=w299:dbl, "Range"=w303:dbl)
                n233 = property on="I" class="DigNum (strict)"("Value"=w301) -> ()  [unwired: 2 in, 2 out]
                n234 = property on="I" class="DigNum (strict)"("Value"=w307) -> ()  [unwired: 2 in, 2 out]
                n235 = property on="I" class="DigNum (strict)"("Value"=w305) -> ()  [unwired: 2 in, 2 out]
                n236 = property on="I" class="DigNum (strict)"("Value"=w299) -> ()  [unwired: 2 in, 2 out]
                n237 = property on="Range" class="Enum (strict)"("Value"=w300) -> ()  [unwired: 2 in, 2 out]
                n238 = property on="Range" class="Enum (strict)"("Value"=w306) -> ()  [unwired: 2 in, 2 out]
                n239 = property on="Range" class="Enum (strict)"("Value"=w304) -> ()  [unwired: 2 in, 2 out]
                n240 = property on="Range" class="Enum (strict)"("Value"=w303) -> ()  [unwired: 2 in, 2 out]
                n241 = property on="I_0" class="DigNum (strict)"("Value"=w299) -> ()  [unwired: 2 in, 2 out]
              }
              frame True {
              }
            }
          }
          frame #4 {
            # "Initialize AVS/zBridge"
            n242 = property on="AVS type" class="Enum (strict)"() -> ("Value"=w314:T35)  [unwired: 2 in, 2 out]
            n243 = case shown="\"Impedance Bridge\"" w314 {
              tunnel: [w322 w331 w348 refnum<visa-resource-name> refnum ("dup VISA session") refnum<visa-resource-name> refnum ("dup VISA session")] -> w313
              tunnel: [w321 w334 _ w357 errorcluster {"status"=FALSE, "code"=0, "source"=""} ("error out")] -> w312
              tunnel: [TRUE ("start 2") TRUE ("start 2") TRUE ("start 2") TRUE ("start 2") TRUE ("start 2")] -> w315
              tunnel: [_ _ w347 _ _] -> _
              frame "AVS47A (GPIB interface)" {
                # "Set default Parameters,\n enable Autoranging"
                n244 = property on="Address" class="VISAName"() -> ("Value"=w316:refnum<visa-resource-name>)  [unwired: 2 in, 2 out]
                n245 = call "AVS47IB Initialize.vi"("Instr. Descriptor (GPIB::)"=w316) -> ("VISA session"=w330:refnum<visa-resource-name>, "error out"=w317:errorcluster)  [unwired: 13 in]
                n246 = call "AVS47IB Stop.vi"("VISA session"=w330, "error in (no error)"=w317) -> ("dup VISA session"=w328:refnum<visa-resource-name>, "error out"=w320:errorcluster)  [unwired: 12 in]
                n247 = call "AVS47IB Go Remote.vi"("VISA session"=w328, "error in (no error)"=w320) -> ("dup VISA session"=w329:refnum<visa-resource-name>, "error out"=w319:errorcluster)  [unwired: 12 in]
                n248 = call "AVS47IB Configure 47IB.vi"("VISA session"=w329, "Printer Enabled (-1:no change)"=i8 0, "Buffer Enabled (-1:no change)"=i8 0, "Message Headers Included  (-1:no change)"=i8 0, "Autoranging Enabled (-1:no change)"=i8 1, "Stabilisation Delay (-1:no change)"=i8 15, "error in (no error)"=w319) -> ("dup VISA session"=w322:refnum<visa-resource-name>, "error out"=w321:errorcluster)  [unwired: 7 in]
              }
              frame "AVS47B (RS232 interface)" {
                n249 = property on="Bridge settings" class="Clust (strict)"() -> ("Value"=w339:T25)  [unwired: 2 in, 2 out]
                n250 = Unbundle By Name(w339) -> ("AVS_SPort"=w338:refnum<visa-resource-name>)
                n251 = call "InitPort_b.vi"("VISA resource"=w338) -> ("error out"=w333:errorcluster, "dup VISA resource"=w337:refnum<visa-resource-name>)  [unwired: 5 in]
                n252 = Type Cast(type=refnum<visa-resource-name> refnum ("dup VISA session"), x=w337) -> (*(type *) &x=w332:refnum<visa-resource-name>)
                n253 = case shown="Error" w333 {
                  selector: w333 -> [w340 w343]
                  tunnel: w332 -> [w341 w345]
                  tunnel: [w340 w344] -> w334
                  tunnel: [w341 refnum<visa-resource-name> refnum ("dup VISA session")] -> w331
                  frame No Error {
                  }
                  frame Error {
                    n254 = VISA Close(VISA resource name=w345, error in (no error)=w343) -> (error out=w344:errorcluster)
                  }
                }
              }
              frame "AVS48" {
                n255 = property on="Bridge settings" class="Clust (strict)"() -> ("Value"=w352:T25)  [unwired: 2 in, 2 out]
                n256 = Unbundle By Name(w352) -> ("AVS_SPort"=w349:refnum<visa-resource-name>)
                n257 = call "Configure Hardware.vi"("VISA RESOURCE NAME"=w349) -> ("THREAD OUT"=w346:string)  [unwired: 14 in]
                n258 = call "Configure Sensor Wiring of CHs.vi"("THREAD IN"=w346) -> ("THREAD OUT"=w347:string)  [unwired: 10 in]
                n259 = Type Cast(type=refnum<visa-resource-name> refnum ("dup VISA session"), x=w349) -> (*(type *) &x=w348:refnum<visa-resource-name>)
              }
              frame "Impedance Bridge" {
                n260 = local read "zConfig"() -> (w356:path)
                n261 = local read "zDll"() -> (w353:path)
                n262 = call "SetParFilePath.vi"("path"=w356, "zDll"=w353) -> ("error out"=w355:errorcluster, "zDll out"=w354:path)  [unwired: 8 in]
                n263 = call "StartScan.vi"("error in (no error)"=w355, "path in"=w354) -> ("error out"=w357:errorcluster)  [unwired: 8 in, 1 out]
              }
              frame "Disabled", Default {
              }
            }
            "AVS VISA session" <- w313
            "start 2" <- w315
            n264 = property on="Bridge status" class="Clust (strict)"("Value"=w312) -> ()  [unwired: 2 in, 2 out]
            n265 = property on="Data array" class="Arr (strict)"("Value"=dbl[] [0.0, 0.0, 0.0, 0.0, 0.0, 0.0, 0.0, 0.0, 0.0, 0.0] ("R_array")) -> ()  [unwired: 2 in, 2 out]
          }
          frame #5 {
            # "Generate paths for log files"
            n266 = Unbundle By Name("Data logging") -> ("Run description"=w366:string, "Filenames suffix"=w367:string, "AVS_Path"=w364:path, "AVS_FName"=w370:string, "CAL_FName"=w369:string)
            n267 = call "Create Dir if Non-Existant__ogtk.vi"("Directory Path"=w364) -> ("dup Directory Path"=w363:path)  [unwired: 8 in, 2 out]
            n268 = call "MGI Make String Filesafe.vi"("String In"=w366) -> ("Filesafe String Out"=w365:string)
            n269 = call "GeneratePaths.vi"("Filename Suffix"=w367, "Run description"=w365, "AVS_Path"=w363, "AVS_FName"=w370, "CAL_Path"=w363, "CAL_FName"=w369) -> ("Generated Log path"=w368:path, "Generated Calib path"=→"Calib path":path)  [unwired: 8 in]
            n270 = property on="Log path" class="Path"("Val(Sgnl)"=w368) -> ()  [unwired: 2 in, 2 out]
          }
        }
      }
      event "Stop": Value Change; Application Instance Close {
        # "\"Stop\" button pressed -> Stop measuring."
        n271 = event-data() -> ()  [unwired: 1 in, 3 out]
        n272 = flat-sequence {
          frame #0 {
            (unwired) T39."HKEY_CURRENT_USER" ("root key (HKEY_LOCAL_MACHINE) 2")
            # "Save settings to config file"
            n273 = control-ref of="Active"() -> (w375:refnum<vi>)
            n274 = control-ref of="Bridge settings"() -> (w384:refnum<vi>)
            n275 = control-ref of="AVS Runtime Settings"() -> (w383:refnum<vi>)
            n276 = control-ref of="Current source settings"() -> (w385:refnum<vi>)
            n277 = control-ref of="Data logging"() -> (w386:refnum<vi>)
            n278 = control-ref of="Thermometer"() -> (w382:refnum<vi>)
            n279 = control-ref of="PID setup 2"() -> (w381:refnum<vi>)
            n280 = control-ref of="CS Names"() -> (w380:refnum<vi>)
            n281 = control-ref of="AVS names"() -> (w379:refnum<vi>)
            n282 = control-ref of="CurCalibrations"() -> (w376:refnum<vi>)
            n283 = control-ref of="I3 as temp"() -> (w374:refnum<vi>)
            n284 = control-ref of="Automode Settings 2"() -> (w373:refnum<vi>)
            n285 = call "Current VIs Parent Directory__ogtk.vi"("Relative path (.)"=path "data/config.ini") -> ("Parent Directory (+ Relative)"=w377:path)  [unwired: 4 in]
            n286 = Build Array(w375, w384, w383, w385, w386, w382, w381, w380, w379, w376, w374, w373) -> (w388:refnum<vi>[])
            n287 = call "Save Load Settings to File by Ref with path.vi"("Array of Cluster References"=w388, "subkey"="SOFTWARE\\Leiden Cryogenics\\TC" ("subkey 2"), "Action"=enum8{"Load", "Save"}."Save", "configuration file path"=w377) -> ()  [unwired: 5 in, 1 out]
          }
          frame #1 {
            # "Free serial ports"
            n288 = control-ref of="AVS VISA session"() -> (w391:refnum<vi>)
            n289 = control-ref of="TCS_Port"() -> (w396:refnum<vi>)
            n290 = local read "zDll"() -> (w390:path)
            n291 = call "StopScan.vi"("path in"=w390) -> ()  [unwired: 9 in, 2 out]
            n292 = property class="VISAName"(reference=w391) -> (error out=w393:errorcluster, "Value"=w392:refnum<visa-resource-name>)  [unwired: 1 in, 1 out]
            n293 = property class="VISAName"(reference=w396) -> (error out=w394:errorcluster, "Value"=w395:refnum<visa-resource-name>)  [unwired: 1 in, 1 out]
            n294 = VISA Close(VISA resource name=w392, error in (no error)=w393) -> ()  [unwired: 1 out]
            n295 = VISA Close(VISA resource name=w395, error in (no error)=w394) -> ()  [unwired: 1 out]
          }
          frame #2 {
            w399 = u8 0 ("Disabled")
            # "Reset controls state"
            n296 = property on="Start" class="Bool (strict)"("Visible"=TRUE, "Disabled"=u8 0, "Value"=FALSE ("start")) -> ()  [unwired: 2 in, 2 out]
            n297 = property on="Stop" class="Bool (strict)"("Value"=FALSE ("MainStopButton")) -> ()  [unwired: 2 in, 2 out]
            n298 = property on="start 2" class="Bool (strict)"("Value"=FALSE ("start 2")) -> ()  [unwired: 2 in, 2 out]
            n299 = property on="AVS type" class="Enum (strict)"("Disabled"=w399) -> ()  [unwired: 2 in, 2 out]
            n300 = property on="Address" class="VISAName"("Disabled"=w399) -> ()  [unwired: 2 in, 2 out]
            n301 = property on="AVS_SPort" class="VISAName"("Disabled"=w399) -> ()  [unwired: 2 in, 2 out]
            n302 = property on="TCS_Port" class="VISAName"("Disabled"=w399) -> ()  [unwired: 2 in, 2 out]
            n303 = property on="CS type" class="Enum (strict)"("Disabled"=w399) -> ()  [unwired: 2 in, 2 out]
            n304 = property on="QCS/PCS Device" class="DigNum (strict)"("Disabled"=w399) -> ()  [unwired: 2 in, 2 out]
          }
          frame #3 {
            w403 = u8 2 ("Disabled")
            # "Disable UI"
            n305 = property on="Toolbar" class="TabCtl (strict)"("Disabled"=w403) -> ()  [unwired: 2 in, 2 out]
            n306 = property on="Tab Control" class="TabCtl (strict)"("Disabled"=w403) -> ()  [unwired: 2 in, 2 out]
            n307 = property on="Current indicators" class="TabCtl (strict)"("Disabled"=w403) -> ()  [unwired: 2 in, 2 out]
            n308 = property on="Tab Control 2" class="TabCtl (strict)"("Disabled"=w403) -> ()  [unwired: 2 in, 2 out]
            n309 = property on="Tab Control 5" class="TabCtl (strict)"("Disabled"=w403) -> ()  [unwired: 2 in, 2 out]
            n310 = property on="String" class="Str"("Visible"=TRUE) -> ()  [unwired: 2 in, 2 out]
          }
          frame #4 {
            # "Stop execution"
            n311 = Stop(stop? (T)=TRUE) -> ()
          }
        }
      }
      event "Data array": Value Change {
        # "Convert 8 elements AVS\narray to 10 elements"
        # "Received new data from AVS/zBridge. Do general tasks - update indicators, calculate temperature and pass the data further to \nAVS/zBridge specific processing"
        n312 = event-data() -> ("NewVal"=w417:dbl[])  [unwired: 1 in, 4 out]
        n313 = for {
          tunnel: w417 -> [w447] mode=indexing
          tunnel: [w445] -> w413 mode=indexing
          n314 = Less?(x=w447, y=1e+25) -> (x < y?=w448:bool)
          n315 = Select(t=w447, s=w448, f=inf) -> (s? t:f=w445:dbl)
        }
        n316 = Index Array(array=w413) -> (element #1=→"R0":dbl, element #2=→"R1":dbl, element #3=→"R2":dbl, element #4=→"R3":dbl, element #5=→"R4":dbl, element #6=→"R5":dbl, element #7=→"R6":dbl, element #8=→"R7":dbl, element #9=→"R8":dbl, element #10=→"R9":dbl)  [unwired: 10 in]
        n317 = Array To Cluster(array=w413) -> (cluster=w407:T41)
        "R" <- w407
        n318 = Cluster To Array(cluster=w407) -> (array=w406:dbl[])
        n319 = Absolute Value(x=w406) -> (abs(x)=w414:dbl[])
        n320 = property on="Allow neg R" class="Bool (strict)"() -> ("Value"=w412:bool)  [unwired: 2 in, 2 out]
        n321 = Select(t=w406, s=w412, f=w414) -> (s? t:f=w411:dbl[])
        n322 = local read "CurCalibrations"() -> (w419:T23)
        n323 = property on="AVS_CalFolder" class="Path"() -> ("Value"=w427:path)  [unwired: 2 in, 2 out]
        n324 = Cluster To Array(cluster=w419) -> (array=w418:string[])
        n325 = call "Resistance to Temp no Ext.vi"("error in"=w420, "Path"=w427, "CurCalibrations"=w418, "Resistance"=w411) -> ("Temperature"=w409:dbl[])  [unwired: 1 in, 3 out]
        "T_array" <- w409
        n326 = Array To Cluster(array=w409) -> (cluster=w425:T42)
        "T" <- w425
        n327 = Unbundle(w425) -> ("Temperature[0]"=→"T0":dbl, "Temperature[1]"=→"T1":dbl, "Temperature[2]"=→"T2":dbl, "Temperature[3]"=→"T3":dbl, "Temperature[4]"=→"T4":dbl, "Temperature[5]"=→"T5":dbl, "Temperature[6]"=→"T6":dbl, "Temperature[7]"=→"T7":dbl, "Temperature[8]"=→"T8":dbl, "Temperature[9]"=→"T9":dbl)
        n328 = property on="Mode Buttons" class="RadioBtnsControl (strict)"() -> ("Value"=w424:T13)  [unwired: 2 in, 2 out]
        n329 = Array To Cluster(array=w411) -> (cluster=w410:T41)
        n330 = Array To Cluster(array=w409) -> (cluster=w408:T42)
        n331 = case shown="\"No Selection\", Default" w424 {
          tunnel: w408 -> [w459 _]
          tunnel: w410 -> [w460 _]
          frame "No Selection", Default {
            n332 = Get Date/Time In Seconds() -> (seconds since 1Jan1904=w462:timestamp)
            n333 = To Double Precision Float(number=w462) -> (double precision float=→"Time":dbl)
            "Small R" <- w460
            "Small T" <- w459
          }
          frame "Cursor Mode" {
          }
        }
        n334 = Bundle(w411, "Temperature"=w409) -> (w422:cluster{dbl[], "Temperature":dbl[]})  [unwired: 1 in]
        n335 = property on="AVS type" class="Enum (strict)"() -> ("Value"=w421:T35)  [unwired: 2 in, 2 out]
        n336 = case shown="\"AVS47B (RS232 interface)\", Default" w421 {
          tunnel: [w453 w454 w457] -> w423
          tunnel: w420 -> [w452 w454 w458]
          tunnel: w422 -> [w450 _ w456]
          frame "AVS47B (RS232 interface)", Default {
            n337 = local read "UpdateValuesAVS"() -> (w451:refnum<user-event>)
            n338 = Generate User Event(user event=w451, event data cluster=w450, error in=w452) -> (error out=w453:errorcluster)  [unwired: 1 in, 1 out]
          }
          frame "Disabled" {
          }
          frame "Impedance Bridge" {
            n339 = local read "UpdateValuesZBridge"() -> (w455:refnum<user-event>)
            n340 = Generate User Event(user event=w455, event data cluster=w456, error in=w458) -> (error out=w457:errorcluster)  [unwired: 1 in, 1 out]
          }
        }
      }
      event User Event {
        # "Process data from the AVS bridge"
        n341 = event-data() -> ("R"=w464:dbl[], "T"=w463:dbl[])  [unwired: 1 in]
        n342 = property on="Actual I" class="Arr (strict)"() -> ("Value"=w465:dbl[])  [unwired: 2 in, 2 out]
        n343 = stacked-sequence {
          tunnel: w467 -> [_ w498]
          tunnel: [_ w512] -> w466
          tunnel: w465 -> [_ w495]
          tunnel: w464 -> [w486 w497]
          tunnel: w463 -> [w487 w496]
          frame #0 {
            # "Filter data and add it to the data array. \nDo PID"
            n344 = property on="AVS Runtime Settings" class="Clust (strict)"() -> ("Value"=w475:T17)  [unwired: 2 in, 2 out]
            n345 = Unbundle By Name(w475) -> ("Y_max"=w478:dbl, "Y_min"=w477:dbl, "Filter graphs:"=w476:bool)
            n346 = local read "Data"() -> (w472:cluster{"R":dbl[], "T":dbl[], "Time":dbl[]}[])
            n347 = property on="Data Memory" class="DigNum (strict)"() -> ("Value"=w480:u16)  [unwired: 2 in, 2 out]
            n348 = Get Date/Time In Seconds() -> (seconds since 1Jan1904=w474:timestamp)
            n349 = To Double Precision Float(number=w474) -> (double precision float=w471:dbl)
            n350 = call "Manage Data Arrays - AVS.vi"("Y_max"=w478, "Y_min"=w477, "Filter Graph Results"=w476, "Append New Data"=TRUE, "Data In"=w472, "Curr R"=w486, "Curr T"=w487, "Curr Time"=w471, "Data Memory"=w480) -> ("Data Out"=w473:cluster{"R":dbl[], "T":dbl[], "Time":dbl[]}[])  [unwired: 10 in]
            n351 = property on="FB on" class="Enum (strict)"() -> ("Value"=w468:enum16{"Resistance", "Temperature"})  [unwired: 2 in, 2 out]
            n352 = local write "Data"(w473) -> ()
            n353 = property on="AVS Channel" class="DigNum (strict)"() -> ("Value"=w469:i32)  [unwired: 2 in, 2 out]
            n354 = Index Array(array=w486, index=w469) -> (element=w485:dbl)
            n355 = Index Array(array=w487, index=w469) -> (element=w484:dbl)
            n356 = case shown="\"Temperature\"" w468 {
              tunnel: w485 -> [w488 _]
              tunnel: [w488 w489] -> w482
              tunnel: w484 -> [_ w489]
              frame "Resistance", Default {
              }
              frame "Temperature" {
              }
            }
            "T controlled" <- w482
            n357 = local read "DoPID"() -> (w483:refnum<user-event>)
            n358 = Bundle(w482, w471) -> (w481:cluster{dbl, dbl})  [unwired: 1 in]
            n359 = Generate User Event(user event=w483, event data cluster=w481) -> ()  [unwired: 2 in, 2 out]
            n360 = local write "Units"(T5 {"AVS Name 0"="O\u0000h\u0000m\u0000\u0000\u0000\u0000\u0000\u0000\u0000\u0000\u0000\u0000\u0000\u0000\u0000\u0000\u0000", "AVS Name 1"="O\u0000h\u0000m\u0000\u0000\u0000\u0000\u0000\u0000\u0000\u0000\u0000\u0000\u0000\u0000\u0000\u0000\u0000", "AVS Name 2"="O\u0000h\u0000m\u0000\u0000\u0000\u0000\u0000\u0000\u0000\u0000\u0000\u0000\u0000\u0000\u0000\u0000\u0000", "AVS Name 3"="O\u0000h\u0000m\u0000\u0000\u0000\u0000\u0000\u0000\u0000\u0000\u0000\u0000\u0000\u0000\u0000\u0000\u0000", "AVS Name 4"="O\u0000h\u0000m\u0000\u0000\u0000\u0000\u0000\u0000\u0000\u0000\u0000\u0000\u0000\u0000\u0000\u0000\u0000", "AVS Name 5"="O\u0000h\u0000m\u0000\u0000\u0000\u0000\u0000\u0000\u0000\u0000\u0000\u0000\u0000\u0000\u0000\u0000\u0000", "AVS Name 6"="O\u0000h\u0000m\u0000\u0000\u0000\u0000\u0000\u0000\u0000\u0000\u0000\u0000\u0000\u0000\u0000\u0000\u0000", "AVS Name 7"="O\u0000h\u0000m\u0000\u0000\u0000\u0000\u0000\u0000\u0000\u0000\u0000\u0000\u0000\u0000\u0000\u0000\u0000", "AVS Name 8"="O\u0000h\u0000m\u0000\u0000\u0000\u0000\u0000\u0000\u0000\u0000\u0000\u0000\u0000\u0000\u0000\u0000\u0000", "AVS Name 9"="O\u0000h\u0000m\u0000\u0000\u0000\u0000\u0000\u0000\u0000\u0000\u0000\u0000\u0000\u0000\u0000\u0000\u0000"} ("Units")) -> ()
          }
          frame #1 {
            # "Save data to log file"
            n361 = local read "Calib path"() -> (w511:path)
            n362 = local read "Log path"() -> (w510:path)
            n363 = call <vilib>:"Check if File or Folder Exists.vi"("path"=w510) -> ("file or folder exists?"=w502:bool, "dup path"=w503:path)  [unwired: 8 in, 1 out]
            n364 = case shown="False" w502 {
              tunnel: w503 -> [w539 w546]
              tunnel: [w539 w546] -> w504
              frame False {
                n365 = control-ref of="Thermometer"() -> (w542:refnum<vi>)
                n366 = property on="Run description" class="Str"() -> ("Value"=w538:string)  [unwired: 2 in, 2 out]
                n367 = Cluster To Array(cluster="AVS names") -> (array=w544:string[])
                n368 = Cluster To Array(cluster="CS Names") -> (array=w545:string[])
                n369 = call "Format log file header Z.vi"("Thermometer"=w542, "AVS names"=w544, "CS Names"=w545, "Run description"=w538) -> ("String"=w540:string)  [unwired: 1 in]
                n370 = Write to Text File(file (use dialog)=w539, text=w540) -> ()  [unwired: 2 in, 3 out]
              }
              frame True {
              }
            }
            n371 = property on="Data logging" class="Clust (strict)"() -> ("Value"=w525:T27)  [unwired: 2 in, 2 out]
            n372 = Unbundle By Name(w525) -> ("Delimeter"=w526:string, "Date/Time Format"=w524:string)
            n373 = Get Date/Time In Seconds() -> (seconds since 1Jan1904=w517:timestamp)
            n374 = To Double Precision Float(number=w517) -> (double precision float=w515:dbl)
            n375 = call "File Info__ogtk.vi"("file"=w504) -> ("file info"=w500:T43, "file out"=w509:path)  [unwired: 5 in, 1 out]
            n376 = Unbundle By Name(w500) -> ("creation date"=w501:u32)
            n377 = Number To Exponential String(number=w515, precision (6)=i16 10) -> (E-format string=w516:string)  [unwired: 2 in]
            n378 = Format Date/Time String(time format string (%c)=w524, seconds (now)=w517) -> (date/time string=w521:string)  [unwired: 1 in]
            n379 = Number To Fractional String(number=w497) -> (F-format string=w523:string[])  [unwired: 3 in]
            n380 = Number To Fractional String(number=w496) -> (F-format string=w522:string[])  [unwired: 3 in]
            n381 = Number To Fractional String(number=w495) -> (F-format string=w520:string[])  [unwired: 3 in]
            n382 = property on="NewFevery" class="DigNum (strict)"() -> ("Value"=w505:u32)  [unwired: 2 in, 2 out]
            n383 = property on="Time Units" class="Enum (strict)"() -> ("Value"=w506:enum16{"Minutes", "Hours", "Days"})  [unwired: 2 in, 2 out]
            n384 = To Time Stamp(1:w501) -> (0:w507:timestamp)
            n385 = Build Array (concatenate)(w521, w516, w523, w522, w520) -> (w519:string[])
            n386 = call "Time Elapsed time.vi"("Time Units"=w506, "Delay Time"=w505, "Time Old In"=w507) -> ("T>dT?"=w508:bool)  [unwired: 2 out]
            n387 = case shown="True" w508 {
              tunnel: [w528 w531] -> w499
              tunnel: [w527 w532] -> _
              tunnel: w509 -> [w528 _]
              tunnel: w511 -> [w527 _]
              frame False {
              }
              frame True {
                n388 = local read "Data logging"() -> (w533:T27)
                n389 = Unbundle By Name(w533) -> ("Run description"=w529:string, "AVS_Path"=w537:path, "AVS_FName"=w535:string, "CAL_FName"=w536:string, "Filenames suffix"=w534:string)
                n390 = call "MGI Make String Filesafe.vi"("String In"=w529) -> ("Filesafe String Out"=w530:string)
                n391 = call "GeneratePaths.vi"("Filename Suffix"=w534, "Run description"=w530, "AVS_Path"=w537, "AVS_FName"=w535, "CAL_Path"=w537, "CAL_FName"=w536) -> ("Generated Log path"=w531:path, "Generated Calib path"=w532:path)  [unwired: 8 in]
                n392 = local write "Calib path"(w532) -> ()
                n393 = property on="Log path" class="Path"("Val(Sgnl)"=w531) -> ()  [unwired: 2 in, 2 out]
              }
            }
            n394 = property on="Thermometer" class="Clust (strict)"() -> ("Controls[]"=w494:refnum<vi>[])  [unwired: 2 in, 2 out]
            n395 = local read "Bridge settings"() -> (w492:T25)
            n396 = Unbundle By Name(w492) -> ("AVS type"=w491:T35)
            n397 = local read "Name"() -> (w490:string)
            n398 = call "Write To Spreadsheet File (string) w Error.vi"("delimiter (\\t)"=w526, "append to file? (new file:F)"=TRUE, "1D data"=w519, "file path (dialog if empty)"=w499) -> ("error out"=w513:errorcluster)  [unwired: 6 in, 1 out]
            n399 = property on="AVS names" class="Clust (strict)"() -> ("Value"=w493:T5)  [unwired: 2 in, 2 out]
            n400 = call <userlib>:"TC_to_DSC.vi"("computer name"=w490, "AVS names"=w493, "AVS type"=w491, "Array"=w494, "I"=w495, "T"=w496, "R"=w497) -> ()  [unwired: 5 in]
            n401 = Merge Errors(w513, w498) -> (w512:errorcluster)
          }
        }
      }
      event User Event {
        # "Process data from the zBridge bridge"
        n402 = event-data() -> ("R"=w553:dbl[], "T"=w552:dbl[])  [unwired: 1 in, 4 out]
        n403 = local read "zBridge params/Error"() -> (w548:string)
        n404 = local read "zBridge set nr."() -> (w554:u8)
        n405 = property on="Actual I" class="Arr (strict)"() -> ("Value"=w551:dbl[])  [unwired: 2 in, 2 out]
        n406 = local read "Unit"() -> (w549:string)
        n407 = stacked-sequence {
          tunnel: w548 -> [w580 _]
          tunnel: w554 -> [w563 w598]
          tunnel: w553 -> [w562 w595]
          tunnel: w552 -> [w561 w594]
          tunnel: w551 -> [_ w593]
          tunnel: w550 -> [_ w621]
          tunnel: [_ w620] -> w547
          tunnel: w549 -> [w566 _]
          frame #0 {
            # "Only do PID after measuring\non selected channel"
            n408 = local read "zBridge params"() -> (w565:T5)
            n409 = local read "Units"() -> (w567:T5)
            n410 = Cluster To Array(cluster=w567) -> (array=w570:string[])
            n411 = Cluster To Array(cluster=w565) -> (array=w581:string[])
            n412 = Replace Array Subset(array=w570, new element=w566, index=w563) -> (w569:string[])
            n413 = Replace Array Subset(array=w581, new element=w580, index=w563) -> (w582:string[])
            n414 = Array To Cluster(array=w569) -> (cluster=→"Units":T44)
            n415 = Array To Cluster(array=w582) -> (cluster=→"zBridge params":T45)
            n416 = property on="AVS Runtime Settings" class="Clust (strict)"() -> ("Value"=w574:T17)  [unwired: 2 in, 2 out]
            n417 = Unbundle By Name(w574) -> ("Y_max"=w577:dbl, "Y_min"=w576:dbl, "Filter graphs:"=w575:bool)
            n418 = local read "Data"() -> (w571:cluster{"R":dbl[], "T":dbl[], "Time":dbl[]}[])
            n419 = property on="FB on" class="Enum (strict)"() -> ("Value"=w555:enum16{"Resistance", "Temperature"})  [unwired: 2 in, 2 out]
            n420 = property on="AVS Channel" class="DigNum (strict)"() -> ("Value"=w556:i32)  [unwired: 2 in, 2 out]
            n421 = property on="Data Memory" class="DigNum (strict)"() -> ("Value"=w579:u16)  [unwired: 2 in, 2 out]
            n422 = Get Date/Time In Seconds() -> (seconds since 1Jan1904=w573:timestamp)
            n423 = To Double Precision Float(number=w573) -> (double precision float=w558:dbl)
            n424 = Index Array(array=w562, index=w556) -> (element=w559:dbl)
            n425 = Index Array(array=w561, index=w556) -> (element=w560:dbl)
            n426 = call "Manage Data Arrays - zBridge.vi"("Y_max"=w577, "Y_min"=w576, "Filter Graph Results"=w575, "Append New Data"=TRUE, "Data In"=w571, "Curr R"=w562, "Curr T"=w561, "Curr Time"=w558, "Channel"=w563, "Data Memory"=w579) -> ("Data Out"=w572:cluster{"R":dbl[], "T":dbl[], "Time":dbl[]}[])  [unwired: 9 in]
            n427 = case shown="\"Resistance\", Default" w555 {
              tunnel: w560 -> [_ w585]
              tunnel: w559 -> [w584 _]
              tunnel: [w584 w585] -> w557
              frame "Resistance", Default {
              }
              frame "Temperature" {
              }
            }
            n428 = local write "Data"(w572) -> ()
            n429 = Equal?(x=w563, y=w556) -> (x = y?=w564:bool)
            n430 = case shown="True" w564 {
              tunnel: w557 -> [_ w587]
              tunnel: w558 -> [_ w586]
              frame False {
              }
              frame True {
                n431 = local read "DoPID"() -> (w589:refnum<user-event>)
                n432 = Bundle(w587, w586) -> (w588:cluster{dbl, dbl})  [unwired: 1 in]
                n433 = Generate User Event(user event=w589, event data cluster=w588) -> ()  [unwired: 2 in, 2 out]
              }
            }
            n434 = property on="T controlled" class="DigNum (strict)"("Value"=w557) -> ()  [unwired: 2 in, 2 out]
          }
          frame #1 {
            n435 = local read "Log path"() -> (w601:path)
            n436 = local read "Data logging"() -> (w619:T27)
            n437 = call "Strip Path Extension - Path__ogtk.vi"("path"=w601) -> ("root"=w602:string, "extension"=w605:string)
            n438 = Format Into String(format string="_%d", initial string=w602, w598) -> (resulting string=w603:string)  [unwired: 1 in, 1 out]
            n439 = Unbundle By Name(w619) -> ("Delimeter"=w634:string, "Date/Time Format"=w633:string)
            n440 = Concatenate Strings(w603, "." ("string"), w605) -> (w600:string)
            n441 = String To Path(string=w600) -> (path=w599:path)
            n442 = call <vilib>:"Check if File or Folder Exists.vi"("path"=w599) -> ("file or folder exists?"=w610:bool, "dup path"=w611:path)  [unwired: 8 in, 1 out]
            n443 = case shown="False" w610 {
              tunnel: w611 -> [w651 w654]
              tunnel: [w651 w654] -> w612
              frame False {
                n444 = local read "AVS names"() -> (w650:T5)
                n445 = local read "CS Names"() -> (w649:T20)
                n446 = control-ref of="Thermometer"() -> (w653:refnum<vi>)
                n447 = property on="Run description" class="Str"() -> ("Value"=w646:string)  [unwired: 2 in, 2 out]
                n448 = Cluster To Array(cluster=w650) -> (array=w647:string[])
                n449 = Cluster To Array(cluster=w649) -> (array=w648:string[])
                n450 = call "Format log file header Z.vi"("Thermometer"=w653, "AVS names"=w647, "CS Names"=w648, "Run description"=w646) -> ("String"=w652:string)  [unwired: 1 in]
                n451 = Write to Text File(file (use dialog)=w651, text=w652) -> ()  [unwired: 2 in, 3 out]
              }
              frame True {
              }
            }
            n452 = Get Date/Time In Seconds() -> (seconds since 1Jan1904=w626:timestamp)
            n453 = To Double Precision Float(number=w626) -> (double precision float=w624:dbl)
            n454 = Number To Exponential String(number=w624, precision (6)=i16 10) -> (E-format string=w625:string)  [unwired: 2 in]
            n455 = Format Date/Time String(time format string (%c)=w633, seconds (now)=w626) -> (date/time string=w630:string)  [unwired: 1 in]
            n456 = Number To Exponential String(number=w595) -> (E-format string=w632:string[])  [unwired: 3 in]
            n457 = Number To Engineering String(4:w594) -> (0:w631:string[])  [unwired: 3 in]
            n458 = Number To Fractional String(number=w593) -> (F-format string=w629:string[])  [unwired: 3 in]
            n459 = call "File Info__ogtk.vi"("file"=w612) -> ("file info"=w608:T43, "file out"=w617:path)  [unwired: 5 in, 1 out]
            n460 = Unbundle By Name(w608) -> ("creation date"=w609:u32)
            n461 = Build Array (concatenate)(w630, w625, w632, w631, w629) -> (w628:string[])
            n462 = local read "Calib path"() -> (w618:path)
            n463 = property on="NewFevery" class="DigNum (strict)"() -> ("Value"=w613:u32)  [unwired: 2 in, 2 out]
            n464 = property on="Time Units" class="Enum (strict)"() -> ("Value"=w614:enum16{"Minutes", "Hours", "Days"})  [unwired: 2 in, 2 out]
            n465 = property on="Thermometer" class="Clust (strict)"() -> ("Controls[]"=w592:refnum<vi>[])  [unwired: 2 in, 2 out]
            n466 = To Time Stamp(1:w609) -> (0:w615:timestamp)
            n467 = call "Time Elapsed time.vi"("Time Units"=w614, "Delay Time"=w613, "Time Old In"=w615) -> ("T>dT?"=w616:bool)  [unwired: 2 out]
            n468 = local read "Bridge settings"() -> (w596:T25)
            n469 = case shown="True" w616 {
              tunnel: [w636 w639] -> w607
              tunnel: [w635 w641] -> _
              tunnel: w617 -> [w636 _]
              tunnel: w618 -> [w635 _]
              frame False {
              }
              frame True {
                n470 = local read "Data logging"() -> (w642:T27)
                n471 = Unbundle By Name(w642) -> ("Run description"=w638:string, "Filenames suffix"=w640:string, "AVS_Path"=w645:path, "AVS_FName"=w643:string, "CAL_FName"=w644:string)
                n472 = call "MGI Make String Filesafe.vi"("String In"=w638) -> ("Filesafe String Out"=w637:string)
                n473 = call "GeneratePaths.vi"("Filename Suffix"=w640, "Run description"=w637, "AVS_Path"=w645, "AVS_FName"=w643, "CAL_Path"=w645, "CAL_FName"=w644) -> ("Generated Log path"=w639:path, "Generated Calib path"=w641:path)  [unwired: 8 in]
                n474 = local write "Calib path"(w641) -> ()
                n475 = property on="Log path" class="Path"("Val(Sgnl)"=w639) -> ()  [unwired: 2 in, 2 out]
              }
            }
            n476 = local read "Name"() -> (w591:string)
            n477 = Unbundle By Name(w596) -> ("AVS type"=w590:T35)
            n478 = call "Write To Spreadsheet File (string) w Error.vi"("delimiter (\\t)"=w634, "append to file? (new file:F)"=TRUE, "1D data"=w628, "file path (dialog if empty)"=w607) -> ("error out"=w622:errorcluster)  [unwired: 6 in, 1 out]
            n479 = property on="AVS names" class="Clust (strict)"() -> ("Value"=w597:T5)  [unwired: 2 in, 2 out]
            n480 = call <userlib>:"TC_to_DSC.vi"("computer name"=w591, "AVS names"=w597, "AVS type"=w590, "Array"=w592, "I"=w593, "T"=w594, "R"=w595) -> ()  [unwired: 5 in]
            n481 = Merge Errors(w622, w621) -> (w620:errorcluster)
          }
        }
      }
      event User Event {
        # "Current source automatic mode"
        # "Check if PID error (SP-PV)==0"
        # "Check if temperature\nis stabilized"
        # "Check if any channel\nis in automatic mode"
        # "Check if stabilization delay time \nis elapsed"
        # "T sabilized?"
        # "If TCS auto mode enabled and temperature is not changing => fire TempStabilized event to save log and set new CS point. Otherwise do PID (if enabled)."
        n482 = event-data() -> ("R/T"=w664:dbl, "Time"=w665:dbl)  [unwired: 1 in, 4 out]
        n483 = local read "I_list[i]"() -> (w658:dbl[])
        n484 = local read "Error"() -> (w668:dbl)
        n485 = property on="N averages" class="DigNum (strict)"() -> ("Value"=w661:i32)  [unwired: 2 in, 2 out]
        n486 = property on="FB to" class="Enum (strict)"() -> ("Value"=w657:enum16{"0", "1", "2", "3"})  [unwired: 2 in, 2 out]
        n487 = local read "Time Old"() -> (w674:dbl)
        n488 = local read "CS Mode"() -> (w656:enum16{"Manual", "Automatic"})
        n489 = property on="T stability" class="DigNum (strict)"() -> ("Value"=w659:dbl)  [unwired: 2 in, 2 out]
        n490 = Equal To 0?(x=w668) -> (x = 0?=w666:bool)
        n491 = property on="Delay Time" class="DigNum (strict)"() -> ("Value"=w660:dbl)  [unwired: 2 in, 2 out]
        n492 = Index Array(array=w658, index=w657) -> (element=w675:dbl)
        n493 = Not Equal To 0?(x=w656) -> (x != 0?=w655:bool)
        n494 = call "Derivatives Pt by Pt.vi"("Points to avg"=w661, "accuracy (%)"=w659, "Time"=w665, "Data"=w664) -> ("Stable?"=w667:bool, "Stability (%)"=→"Slope":dbl, "dt (s)"=w671:dbl)  [unwired: 3 in]
        n495 = call "Time Elapsed dbl.vi"("Delay Time"=w660, "Time Old In"=w674) -> ("T>dT?"=w663:bool, "Delta T"=→"Timer":dbl, "Time New Out"=w673:dbl)  [unwired: 1 in]
        n496 = Compound Arithmetic op=AND(w663, w655, w666, w667) -> (w669:bool)
        "SP reached?" <- w669
        n497 = property on="Enable PID" class="Bool (strict)"() -> ("Value"=w662:bool)  [unwired: 2 in, 2 out]
        n498 = case shown="False" w669 {
          tunnel: w673 -> [_ w692]
          tunnel: w671 -> [w690 _]
          tunnel: w664 -> [w684 _]
          tunnel: w662 -> [w682 _]
          tunnel: w675 -> [w683 _]
          tunnel: w658 -> [w679 _]
          tunnel: w657 -> [w678 _]
          tunnel: w655 -> [w676 _]
          frame False {
            # "Temperature is not stable. If enabled, do PID regulation"
            n499 = And(x=w682, y=w676) -> (x .and. y?=w677:bool)
            n500 = local read "PID setup 2"() -> (w687:T32)
            n501 = property on="I_0" class="DigNum (strict)"() -> ("Value"=w688:dbl)  [unwired: 2 in, 2 out]
            n502 = call "PID control incremental.vi"("Process Variable"=w684, "dt"=w690, "Setpoint"=w683, "PID Settings"=w687, "I in"=w688, "PID Enabled"=w677) -> ("err out"=→"Error":dbl, "int out"=→"Int":dbl, "I out"=w681:dbl)  [unwired: 10 in, 1 out]
            n503 = Bundle("Numeric"=w683, "R/T"=w684) -> (→"PID-Plot":cluster{"Numeric":dbl, "R/T":dbl})  [unwired: 1 in]
            n504 = Replace Array Subset(array=w679, new element=w681, index=w678) -> (→"I_in":dbl[])
          }
          frame True {
            # "Temperature is stable & automode is on"
            n505 = case shown="False" "Call external VI" {
              tunnel: w692 -> [w695 _]
              frame False {
                # "External VI call disabled -> proceed\nwith automode"
                n506 = local write "Time Old"(w695) -> ()
                n507 = property on="TempStabilized" class="TypRef (strict)"() -> ("Value"=w694:refnum<user-event>)  [unwired: 2 in, 2 out]
                n508 = Generate User Event(user event=w694, event data cluster=TRUE ("event data")) -> ()  [unwired: 2 in, 2 out]
              }
              frame True {
                # "Call external VI"
                n509 = property on="CallExtVI" class="TypRef (strict)"() -> ("Value"=w696:refnum<user-event>)  [unwired: 2 in, 2 out]
                n510 = Generate User Event(user event=w696, event data cluster="" ("event data")) -> ()  [unwired: 2 in, 2 out]
              }
            }
          }
        }
      }
      event User Event {
        n511 = event-data() -> ()  [unwired: 1 in, 5 out]
        n512 = local read "vi reference"() -> (w701:refnum<vi>)
        n513 = call "GetExtVIStatus.vi"("vi reference in"=w701) -> ("vi reference out"=w698:refnum<vi>, "Exec.State"=w700:T30, "Finished?"=w699:bool)
        n514 = case shown="\"Idle\"" w700 {
          tunnel: w699 -> [_ _]
          tunnel: w698 -> [_ w702]
          frame "Bad", Default {
          }
          frame "Idle" {
            n515 = local read "VI called?"() -> (w703:bool)
            n516 = case shown="True" w703 {
              tunnel: w702 -> [w705 _]
              frame False {
                n517 = property on="Data array" class="Arr (strict)"() -> ("Value"=w708:dbl[])  [unwired: 2 in, 2 out]
                n518 = property on="T_array" class="Arr (strict)"() -> ("Value"=w709:dbl[])  [unwired: 2 in, 2 out]
                n519 = property on="I" class="Arr (strict)"() -> ("Value"=w710:dbl[])  [unwired: 2 in, 2 out]
                n520 = Format Date/Time String() -> (date/time string=w707:string)  [unwired: 3 in]
                n521 = Bundle("date/time string"=w707, "Value"=w708, "Value"=w709, "Value"=w710) -> (w706:T46)  [unwired: 1 in]
                n522 = call "CallExtVI.vi"("vi reference in"=w705, "Cluster"=w706) -> ()  [unwired: 1 out]
                "VI called?" <- TRUE ("VI called?")
              }
              frame True {
                n523 = property on="TempStabilized" class="TypRef (strict)"() -> ("Value"=w712:refnum<user-event>)  [unwired: 2 in, 2 out]
                n524 = Get Date/Time In Seconds() -> (seconds since 1Jan1904=w713:timestamp)
                n525 = To Double Precision Float(number=w713) -> (double precision float=w714:dbl)
                n526 = Generate User Event(user event=w712, event data cluster=TRUE ("event data")) -> ()  [unwired: 2 in, 2 out]
                n527 = local write "Time Old"(w714) -> ()
              }
            }
          }
        }
      }
      event User Event {
        # "CS automode\nT is stabilized"
        n528 = event-data() -> ("TempStabilized"=w715:bool)  [unwired: 1 in, 4 out]
        n529 = stacked-sequence {
          tunnel: w717 -> [w723 _]
          tunnel: [w724 _] -> w716
          tunnel: w715 -> [_ w744]
          frame #0 {
            # "Step1: Save R,T,I values to calibration file. Make screenshot when creating the calibration file."
            n530 = property on="Calib path" class="Path"() -> ("Value"=w719:path)  [unwired: 2 in, 2 out]
            n531 = call "File Exists__ogtk.vi"("file path"=w719) -> ("exists"=w720:bool)  [unwired: 6 in, 1 out]
            n532 = case shown="False" w720 {
              tunnel: w719 -> [w733 w743]
              tunnel: [w733 w743] -> w718
              frame False {
                n533 = local read "AVS names"() -> (w740:T5)
                n534 = local read "CS Names"() -> (w739:T20)
                n535 = control-ref of="Thermometer"() -> (w742:refnum<vi>)
                n536 = property on="Run description" class="Str"() -> ("Value"=w736:string)  [unwired: 2 in, 2 out]
                n537 = Cluster To Array(cluster=w740) -> (array=w737:string[])
                n538 = Cluster To Array(cluster=w739) -> (array=w738:string[])
                n539 = call "Format log file header Z.vi"("Thermometer"=w742, "AVS names"=w737, "CS Names"=w738, "Run description"=w736) -> ("String"=w741:string)  [unwired: 1 in]
                n540 = Write to Text File(file (use dialog)=w733, text=w741) -> ()  [unwired: 2 in, 3 out]
                n541 = control-ref of="This VI"() -> (w735:refnum<vi>)
                n542 = invoke class="VI" method="FP.Get Image"(reference=w735) -> ("image data"=w734:T47)  [unwired: 5 in, 5 out]
                n543 = call "Convert File Extension (Path)__ogtk.vi"("new ending (none)"="png" ("name or relative path"), "file name"=w733) -> ("new filename"=w732:path)  [unwired: 1 out]
                n544 = call <vilib>:"Write PNG File.vi"("image data"=w734, "path to PNG file"=w732) -> ()  [unwired: 8 in, 2 out]
              }
              frame True {
              }
            }
            n545 = local write "VI called?"(FALSE ("VI called?")) -> ()
            n546 = property on="Data logging" class="Clust (strict)"() -> ("Value"=w727:T27)  [unwired: 2 in, 2 out]
            n547 = Unbundle By Name(w727) -> ("Date/Time Format"=w728:string, "Delimeter"=w725:string)
            n548 = property on="R" class="Clust (strict)"() -> ("Value"=w726:T8)  [unwired: 2 in, 2 out]
            n549 = property on="T" class="Clust (strict)"() -> ("Value"=w730:T4)  [unwired: 2 in, 2 out]
            n550 = property on="I" class="Arr (strict)"() -> ("Value"=w729:dbl[])  [unwired: 2 in, 2 out]
            n551 = call "Write to cal log file.vi"("Value 2"=w729, "Date/Time Format"=w728, "Value 3"=w730, "Value"=w726, "Delimeter"=w725, "Value 4"=w718) -> ("error out"=w722:errorcluster)  [unwired: 1 out]
            n552 = Merge Errors(w722, w723) -> (w724:errorcluster)
          }
          frame #1 {
            # "Step 2: Sweep through the currents list"
            n553 = case shown="True" w744 {
              frame False {
              }
              frame True {
                n554 = local read "I_list_idx_max"() -> (w746:i32)
                n555 = local read "I_list_idx"() -> (w747:i32)
                n556 = Less?(x=w747, y=w746) -> (x < y?=w745:bool)
                n557 = case shown="False" w745 {
                  frame False {
                    n558 = property on="CS Mode" class="Enum (strict)"("Val(Sgnl)"=enum16{"Manual", "Automatic"}."Manual" ("Value (Signaling)")) -> ()  [unwired: 2 in, 2 out]
                  }
                  frame True {
                    n559 = property on="I_next" class="Bool (strict)"("Val(Sgnl)"=TRUE) -> ()  [unwired: 2 in, 2 out]
                  }
                }
              }
            }
          }
        }
      }
      event User Event {
        # "Disable controls for disabled channels"
        n560 = event-data() -> ()  [unwired: 1 in, 5 out]
        n561 = property on="AVS type" class="Enum (strict)"() -> ("Value"=w757:T35)  [unwired: 2 in, 2 out]
        n562 = case shown="\"Impedance Bridge\"" w757 {
          tunnel: [w767 w778 w787] -> w756
          frame Default {
            n563 = property on="AVS Runtime Settings" class="Clust (strict)"() -> ("Value"=w771:T17)  [unwired: 2 in, 2 out]
            n564 = Unbundle By Name(w771) -> ("Read AVS channels from"=w769:i8, "Last Channel"=w770:i8)
            n565 = for {
              N: 10 -> [_]
              tunnel: w770 -> [w773]
              tunnel: w769 -> [w774]
              tunnel: [w772] -> w767 mode=indexing
              i -> [w775]
              n566 = Less Or Equal?(x=w774, y=w775) -> (x <= y?=w777:bool)
              n567 = Less Or Equal?(x=w775, y=w773) -> (x <= y?=w776:bool)
              n568 = And(x=w777, y=w776) -> (x .and. y?=w772:bool)
            }
          }
          frame "Impedance Bridge" {
            n569 = local read "zDll"() -> (w779:path)
            n570 = for {
              N: 10 -> [_]
              tunnel: [w782] -> w780 mode=indexing
              tunnel: w779 -> [w783]
              i -> [w785]
              n571 = call "GetByteParam.vi"("ParNo"=u8 0, "SetNo"=w785, "zDll"=w783) -> ("return type"=w782:u8)  [unwired: 6 in, 2 out]
            }
            n572 = Greater Than 0?(x=w780) -> (x > 0?=w778:bool[])
          }
          frame "AVS47B (RS232 interface)" {
            n573 = local read "Active"() -> (w786:T12)
            n574 = Cluster To Array(cluster=w786) -> (array=w787:bool[])
          }
        }
        n575 = control-ref of="Active"() -> (w763:refnum<vi>)
        n576 = control-ref of="Exc&Ranges"() -> (w759:refnum<vi>)
        n577 = control-ref of="R"() -> (w764:refnum<vi>)
        n578 = control-ref of="Thermometer"() -> (w765:refnum<vi>)
        n579 = control-ref of="T"() -> (w766:refnum<vi>)
        n580 = control-ref of="uPlots"() -> (w760:refnum<vi>)
        n581 = control-ref of="AVS names"() -> (w758:refnum<vi>)
        n582 = control-ref of="zBridge params"() -> (w755:refnum<vi>)
        n583 = control-ref of="Status"() -> (w754:refnum<vi>)
        n584 = control-ref of="Units"() -> (w753:refnum<vi>)
        n585 = control-ref of="AVS names small"() -> (w752:refnum<vi>)
        n586 = control-ref of="Small R"() -> (w751:refnum<vi>)
        n587 = control-ref of="Small T"() -> (w750:refnum<vi>)
        n588 = Build Array(w763, w759, w764, w765, w766, w760, w758, w755, w754, w753, w752, w751, w750) -> (w761:refnum<vi>[])
        n589 = Array Size(array=w761) -> (size(s)=w762:i32)
        n590 = for {
          N: w762 -> [_]
          tunnel: w761 -> [w791] mode=indexing
          tunnel: w756 -> [w788]
          n591 = property class="Clust"(reference=w791) -> ("Controls[]"=w789:refnum<vi>[])  [unwired: 1 in, 2 out]
          n592 = Array Size(array=w789) -> (size(s)=w790:i32)
          n593 = for {
            N: w790 -> [_]
            tunnel: w789 -> [w793] mode=indexing
            tunnel: w788 -> [w792] mode=indexing
            n594 = case shown="True" w792 {
              tunnel: w793 -> [w794 w799]
              frame False {
                n595 = property class="Ctl"(reference=w794, "Disabled"=u8 2) -> ("ClassName"=w795:string)  [unwired: 1 in, 2 out]
                n596 = case shown="\"Boolean\"" w795 {
                  tunnel: w794 -> [_ w798 _]
                  frame "False", Default {
                  }
                  frame "Boolean" {
                    n597 = property class="Ctl"(reference=w798, "Value"=FALSE) -> ()  [unwired: 1 in, 2 out]
                  }
                  frame "Ring" {
                  }
                }
              }
              frame True {
                n598 = property class="Ctl"(reference=w799, "Disabled"=u8 0) -> ("ClassName"=w800:string)  [unwired: 1 in, 2 out]
                n599 = case shown="\"Boolean\"" w800 {
                  tunnel: w799 -> [_ w803]
                  frame "False", Default {
                  }
                  frame "Boolean" {
                    n600 = property class="Ctl"(reference=w803, "Value"=TRUE) -> ()  [unwired: 1 in, 2 out]
                  }
                }
              }
            }
          }
        }
      }
      event "Log path": Value Change {
        # "Modify window title to show measurement information"
        n601 = event-data() -> ("NewVal"=w810:path)  [unwired: 1 in, 5 out]
        n602 = property on="Run description" class="Str"() -> ("Value"=w804:string)  [unwired: 2 in, 2 out]
        n603 = property on="AVS type" class="Enum (strict)"() -> ("RingText.Text"=w805:string)  [unwired: 2 in, 2 out]
        n604 = property on="CS type" class="Enum (strict)"() -> ("RingText.Text"=w808:string)  [unwired: 2 in, 2 out]
        n605 = Path To String(path=w810) -> (string=w807:string)
        n606 = Format Into String(format string="%s - %s - %s   (%s)", w804, w805, w808, w807) -> (resulting string=w806:string)  [unwired: 2 in, 1 out]
        n607 = control-ref of="This VI"() -> (w811:refnum<vi>)
        n608 = property class="VI"(reference=w811, "Front Panel.Title"=w806) -> ()  [unwired: 1 in, 2 out]
      }
      event "Refresh Calibrations", "Bridge settings.AVS_CalFolder": Value Change; User Event {
        # "Refresh the list of calibration files"
        n609 = event-data() -> ()  [unwired: 1 in, 3 out]
        n610 = control-ref of="Thermometer"() -> (w818:refnum<vi>)
        n611 = control-ref of="CurCalibrations"() -> (w812:refnum<vi>)
        n612 = control-ref of="AVS_CalFolder"() -> (w816:refnum<vi>)
        n613 = control-ref of="Select sensor 1"() -> (w817:refnum<vi>)
        n614 = control-ref of="Select sensor 1"() -> (w815:refnum<vi>)
        n615 = call "ReloadCalibrations.vi"("error in (no error)"=w814, "Quick convert sensors"=w815, "CurCalibrations"=w812, "Calibration files path"=w816, "Channel1 sensors"=w817, "Channels list"=w818) -> ("error out"=w813:errorcluster)  [unwired: 1 in]
      }
      event "Mode Buttons": Value Change {
        w824 = refnum<vi> refnum  # XYGraph
        # "Show cursor on plot is \"Cursor\" or \"Delete points\" mode is enabled"
        # "!!NOTE:This routine assumes that XY graph is control #0 on tab page!!"
        n616 = event-data() -> ("NewVal"=w820:T13)  [unwired: 1 in, 5 out]
        n617 = property on="Channel Controls" class="TabCtl (strict)"() -> ("Pages"=w828:refnum<vi>[], "Value"=w827:T3)  [unwired: 2 in, 2 out]
        n618 = Index Array(array=w828, index=w827) -> (element=w826:refnum<vi>)
        n619 = property class="Page"(reference=w826) -> ("ControlsOnPage"=w821:refnum<vi>[])  [unwired: 1 in, 2 out]
        n620 = Index Array(array=w821, index=0) -> (element=w825:refnum<vi>)
        n621 = Type Cast(type=w824, x=w825) -> (*(type *) &x=w819:refnum<vi>)
        n622 = case shown="\"Erase Range\"" w820 {
          tunnel: w819 -> [w829 w838 w846 w854]
          frame "No Selection", Default {
            n623 = property class="XYGraph"(reference=w829, "Active Cursor"=u32 0, "Cursor.Visible"=FALSE) -> (reference out=w832:refnum<vi>)  [unwired: 1 in, 1 out]
            n624 = property class="XYGraph"(reference=w832, "Active Cursor"=u32 1, "Cursor.Visible"=FALSE) -> ()  [unwired: 1 in, 2 out]
          }
          frame "Erase Range" {
            n625 = property class="XYGraph"(reference=w838, "Active Cursor"=u32 0, "Cursor.Visible"=TRUE, "Cursor.Cursor Color"=u32 16777062, "Cursor.Cursor Index"=0, "ActPaletteTool"=0 ("Palette:Active Tool")) -> (reference out=w841:refnum<vi>)  [unwired: 1 in, 1 out]
            n626 = property class="XYGraph"(reference=w841, "Active Cursor"=u32 1, "Cursor.Visible"=TRUE, "Cursor.Cursor Color"=u32 6618880) -> ()  [unwired: 1 in, 2 out]
          }
          frame "Cursor Mode" {
            n627 = property class="XYGraph"(reference=w846, "Active Cursor"=u32 0, "Cursor.Visible"=TRUE, "Cursor.Cursor Color"=u32 6618880, "ActPaletteTool"=0 ("Palette:Active Tool")) -> (reference out=w849:refnum<vi>)  [unwired: 1 in, 1 out]
            n628 = property class="XYGraph"(reference=w849, "Active Cursor"=u32 1, "Cursor.Visible"=FALSE) -> ()  [unwired: 1 in, 2 out]
          }
          frame "Erase point" {
            n629 = property class="XYGraph"(reference=w854, "Active Cursor"=u32 0, "Cursor.Visible"=TRUE, "Cursor.Cursor Color"=u32 16777062, "ActPaletteTool"=0 ("Palette:Active Tool")) -> (reference out=w857:refnum<vi>)  [unwired: 1 in, 1 out]
            n630 = property class="XYGraph"(reference=w857, "Active Cursor"=u32 1, "Cursor.Visible"=FALSE) -> ()  [unwired: 1 in, 2 out]
          }
        }
      }
      event "R-Plot 0", "R-Plot 1", "R-Plot 2", "R-Plot 3", "R-Plot 4", "R-Plot 5", "R-Plot 6", "R-Plot 7", "R-Plot 8", "R-Plot 9": Mouse Down? {
        # "Disabled"
        n631 = event-data() -> ("CtlRef"=w862:refnum<vi>, "Button"=w867:u16, "Mods.Double Click"=w864:bool)  [unwired: 1 in, 5 out]
        n632 = Equal?(x=u16 1, y=w867) -> (x = y?=w865:bool)
        n633 = And(x=w865, y=w864) -> (x .and. y?=w863:bool)
        n634 = disable-structure shown="Disabled" {
          disable-tunnel: w863 -> [w870 _]
          disable-tunnel: w862 -> [w869 _]
          disable-tunnel: "Mode Buttons" -> [w868 _]
          frame Disabled {
            n635 = case shown="True" w870 {
              tunnel: w868 -> [_ w872]
              tunnel: w869 -> [_ w871]
              frame False {
              }
              frame True {
                n636 = case shown="\"Erase Range\"" w872 {
                  tunnel: w871 -> [_ w873]
                  frame "No Selection", Default {
                  }
                  frame "Erase Range" {
                    n637 = property class="XYGraph (strict)"(reference=w873, "ActPaletteTool"=0 ("Palette:Active Tool"), "Active Cursor"=u32 0, "Cursor.Visible"=TRUE) -> ()  [unwired: 1 in, 2 out]
                  }
                }
              }
            }
          }
          frame Enabled {
          }
        }
        n638 = event-data() -> ()  [unwired: 5 in, 1 out]
      }
      event "R-Plot 0", "R-Plot 1", "R-Plot 2", "R-Plot 3", "R-Plot 4", "R-Plot 5", "R-Plot 6", "R-Plot 7", "R-Plot 8", "R-Plot 9": Mouse Down {
        # "Process (double) click on plots in special modes (\"Cursor\", \"Erase\")"
        n639 = event-data() -> ("CtlRef"=w878:refnum<vi>, "Coords"=w881:T48, "Button"=w877:u16, "Mods.Double Click"=w880:bool)  [unwired: 1 in, 4 out]
        n640 = property on="Mode Buttons" class="RadioBtnsControl (strict)"() -> ("Value"=w879:T13)  [unwired: 2 in, 2 out]
        n641 = case shown="1" w877 {
          tunnel: w881 -> [_ w915]
          tunnel: w880 -> [_ w914]
          tunnel: w879 -> [w886 w913]
          tunnel: w878 -> [w887 w912]
          frame 0, Default {
            n642 = local read "LMB Down"() -> (w884:bool)
            n643 = Equal?(x=w886, y=T13."Erase Range" ("Mode Buttons")) -> (x = y?=w885:bool)
            n644 = And(x=w884, y=w885) -> (x .and. y?=w883:bool)
            n645 = case shown="True" w883 {
              tunnel: w887 -> [_ w910]
              frame False {
              }
              frame True {
                n646 = property class="XYGraph (strict)"(reference=w910, "Active Cursor"=u32 0, "Active Cursor"=u32 1) -> ("Cursor.Cursor X"=w907:dbl, "Cursor.Cursor X"=w888:dbl)  [unwired: 1 in, 2 out]
                n647 = local read "Channel Controls"() -> (w909:T3)
                n648 = local read "Data"() -> (w904:cluster{"R":dbl[], "T":dbl[], "Time":dbl[]}[])
                n649 = Max & Min(x=w907, y=w888) -> (max(x,y)=w897:dbl, min(x,y)=w890:dbl)
                n650 = Index Array(array=w904, index=w909) -> (element=w900:cluster{"R":dbl[], "T":dbl[], "Time":dbl[]})
                n651 = Unbundle By Name(w900) -> ("R"=w898:dbl[], "T"=w899:dbl[], "Time"=w896:dbl[])
                n652 = Threshold 1D Array(2:w897, 3:w896) -> (0:w894:dbl)  [unwired: 1 in]
                n653 = Threshold 1D Array(2:w890, 3:w896) -> (0:w895:dbl)  [unwired: 1 in]
                n654 = Subtract(x=w894, y=w895) -> (x-y=w893:dbl)
                n655 = Delete From Array(array=w898, length=w893, index=w895) -> (array with subset deleted=w903:dbl[])  [unwired: 1 out]
                n656 = Delete From Array(array=w899, length=w893, index=w895) -> (array with subset deleted=w902:dbl[])  [unwired: 1 out]
                n657 = Delete From Array(array=w896, length=w893, index=w895) -> (array with subset deleted=w901:dbl[])  [unwired: 1 out]
                n658 = Bundle By Name(cluster=w900, "R"=w903, "T"=w902, "Time"=w901) -> (w905:cluster{"R":dbl[], "T":dbl[], "Time":dbl[]})
                n659 = Replace Array Subset(array=w904, new element=w905, index=w909) -> (w906:cluster{"R":dbl[], "T":dbl[], "Time":dbl[]}[])
                n660 = local write "Data"(w906) -> ()
                n661 = property class="XYGraph (strict)"(reference=w910, "Active Cursor"=u32 0, "Cursor.Cursor X"=w890, "Active Cursor"=u32 1, "Cursor.Cursor X"=w890) -> ()  [unwired: 1 in, 2 out]
              }
            }
          }
          frame 1 {
            n662 = case shown="\"Cursor Mode\"" w913 {
              tunnel: w912 -> [_ w918 w939 w947]
              tunnel: w915 -> [_ w917 w938 w949]
              tunnel: w914 -> [_ w916 w940 w948]
              frame "No Selection", Default {
              }
              frame "Cursor Mode" {
                n663 = case shown="True" w916 {
                  tunnel: w918 -> [_ w928]
                  tunnel: w917 -> [_ w926]
                  frame False {
                  }
                  frame True {
                    n664 = invoke class="XYGraph (strict)" method="Map Coords To XY"(reference=w928, "Coords"=w926) -> (reference out=w927:refnum<vi>, "XY"=w925:cluster{"X":dbl, "Y":dbl})  [unwired: 5 in, 5 out]
                    n665 = Unbundle By Name(w925) -> ("X"=w923:dbl)
                    n666 = local read "Data"() -> (w924:cluster{"R":dbl[], "T":dbl[], "Time":dbl[]}[])
                    n667 = property class="XYGraph (strict)"(reference=w927, "Active Cursor"=u32 0, "Cursor.Cursor Position"=w925) -> ()  [unwired: 1 in, 2 out]
                    n668 = for {
                      tunnel: w924 -> [w937] mode=indexing
                      tunnel: w923 -> [w935]
                      tunnel: [w931] -> w922 mode=indexing
                      tunnel: [w930] -> w921 mode=indexing
                      n669 = Unbundle By Name(w937) -> ("R"=w934:dbl[], "T"=w933:dbl[], "Time"=w936:dbl[])
                      n670 = Threshold 1D Array(2:w935, 3:w936) -> (0:w932:dbl)  [unwired: 1 in]
                      n671 = Index Array(array=w934, index=w932) -> (element=w931:dbl)
                      n672 = Index Array(array=w933, index=w932) -> (element=w930:dbl)
                    }
                    n673 = Array To Cluster(array=w921) -> (cluster=w919:T41)
                    n674 = Array To Cluster(array=w922) -> (cluster=w920:T41)
                    n675 = property on="Time" class="DigNum (strict)"("Value"=w923) -> ()  [unwired: 2 in, 2 out]
                    n676 = property on="Small R" class="Clust (strict)"("Value"=w920) -> ()  [unwired: 2 in, 2 out]
                    n677 = property on="Small T" class="Clust (strict)"("Value"=w919) -> ()  [unwired: 2 in, 2 out]
                  }
                }
              }
              frame "Erase Range" {
                n678 = case shown="False" w940 {
                  tunnel: w939 -> [w944 _]
                  tunnel: w938 -> [w943 _]
                  frame False {
                    n679 = invoke class="XYGraph (strict)" method="Map Coords To XY"(reference=w944, "Coords"=w943) -> (reference out=w946:refnum<vi>, "XY"=w941:cluster{"X":dbl, "Y":dbl})  [unwired: 5 in, 5 out]
                    n680 = property class="XYGraph (strict)"(reference=w946, "Active Cursor"=u32 0, "Cursor.Cursor Position"=w941, "Active Cursor"=u32 1, "Cursor.Cursor Position"=w941) -> ()  [unwired: 1 in, 2 out]
                  }
                  frame True {
                  }
                }
              }
              frame "Erase point" {
                n681 = case shown="False" w948 {
                  tunnel: w947 -> [w954 w969]
                  tunnel: w949 -> [w953 _]
                  frame False {
                    n682 = invoke class="XYGraph (strict)" method="Map Coords To XY"(reference=w954, "Coords"=w953) -> (reference out=w952:refnum<vi>, "XY"=w951:cluster{"X":dbl, "Y":dbl})  [unwired: 5 in, 5 out]
                    n683 = property class="XYGraph (strict)"(reference=w952, "Active Cursor"=u32 0, "Cursor.Cursor Position"=w951) -> ()  [unwired: 1 in, 2 out]
                  }
                  frame True {
                    n684 = property class="XYGraph (strict)"(reference=w969, "Active Cursor"=u32 0) -> ("Cursor.Cursor X"=w956:dbl)  [unwired: 1 in, 2 out]
                    n685 = local read "Channel Controls"() -> (w955:T3)
                    n686 = local read "Data"() -> (w965:cluster{"R":dbl[], "T":dbl[], "Time":dbl[]}[])
                    n687 = Index Array(array=w965, index=w955) -> (element=w961:cluster{"R":dbl[], "T":dbl[], "Time":dbl[]})
                    n688 = Unbundle By Name(w961) -> ("R"=w957:dbl[], "T"=w958:dbl[], "Time"=w959:dbl[])
                    n689 = Threshold 1D Array(2:w956, 3:w959) -> (0:w960:dbl)  [unwired: 1 in]
                    n690 = Delete From Array(array=w957, index=w960) -> (array with subset deleted=w964:dbl[])  [unwired: 1 in, 1 out]
                    n691 = Delete From Array(array=w958, index=w960) -> (array with subset deleted=w963:dbl[])  [unwired: 1 in, 1 out]
                    n692 = Delete From Array(array=w959, index=w960) -> (array with subset deleted=w962:dbl[])  [unwired: 1 in, 1 out]
                    n693 = Bundle By Name(cluster=w961, "R"=w964, "T"=w963, "Time"=w962) -> (w966:cluster{"R":dbl[], "T":dbl[], "Time":dbl[]})
                    n694 = Replace Array Subset(array=w965, new element=w966, index=w955) -> (w967:cluster{"R":dbl[], "T":dbl[], "Time":dbl[]}[])
                    n695 = local write "Data"(w967) -> ()
                  }
                }
              }
            }
            "LMB Down" <- TRUE ("Mouse down")
          }
        }
      }
      event "R-Plot 0", "R-Plot 1", "R-Plot 2", "R-Plot 3", "R-Plot 4", "R-Plot 5", "R-Plot 6", "R-Plot 7", "R-Plot 8", "R-Plot 9": Mouse Move {
        # "Process mouse movement over plots in special modes (\"Cursor\", \"Erase\")"
        n696 = event-data() -> ("CtlRef"=w970:refnum<vi>, "Coords"=w971:T48)  [unwired: 1 in, 3 out]
        n697 = property on="Mode Buttons" class="RadioBtnsControl (strict)"() -> ("Value"=w975:T13)  [unwired: 2 in, 2 out]
        n698 = local read "LMB Down"() -> (w976:bool)
        n699 = Equal?(x=w975, y=T34."Erase Range") -> (x = y?=w972:bool)
        n700 = And(x=w976, y=w972) -> (x .and. y?=w973:bool)
        n701 = case shown="True" w973 {
          tunnel: w971 -> [_ w978]
          tunnel: w970 -> [_ w977]
          frame False {
          }
          frame True {
            n702 = invoke class="XYGraph (strict)" method="Map Coords To XY"(reference=w977, "Coords"=w978) -> (reference out=w981:refnum<vi>, "XY"=w980:cluster{"X":dbl, "Y":dbl})  [unwired: 5 in, 5 out]
            n703 = property class="XYGraph (strict)"(reference=w981, "Active Cursor"=u32 1, "Cursor.Cursor Position"=w980) -> ()  [unwired: 1 in, 2 out]
          }
        }
      }
      event "R-Plot 0", "R-Plot 1", "R-Plot 2", "R-Plot 3", "R-Plot 4", "R-Plot 5", "R-Plot 6", "R-Plot 7", "R-Plot 8", "R-Plot 9": Mouse Up {
        n704 = event-data() -> ("CtlRef"=w984:refnum<vi>, "Button"=w982:u16)  [unwired: 1 in, 6 out]
        n705 = property on="Mode Buttons" class="RadioBtnsControl (strict)"() -> ("Value"=w985:T13)  [unwired: 2 in, 2 out]
        n706 = property class="XYGraph (strict)"(reference=w984) -> ("ActPaletteTool"=w983:i32)  [unwired: 1 in, 2 out]
        n707 = case shown="1" w982 {
          tunnel: w985 -> [_ w989]
          tunnel: w984 -> [_ w988]
          tunnel: w983 -> [_ w987]
          frame 0, Default {
          }
          frame 1 {
            n708 = local write "LMB Down"(FALSE ("Mouse down")) -> ()
            n709 = case shown="Default" w987 {
              tunnel: w989 -> [_ _]
              tunnel: w988 -> [_ _]
              frame Default {
                n710 = property on="Mode Buttons" class="RadioBtnsControl (strict)"("Val(Sgnl)"=T13."No Selection" ("Value (Signaling)")) -> ()  [unwired: 2 in, 2 out]
              }
              frame 0 {
              }
            }
          }
        }
      }
      event "R-Plot 0", "R-Plot 1", "R-Plot 2", "R-Plot 3", "R-Plot 4", "R-Plot 5", "R-Plot 6", "R-Plot 7", "R-Plot 8", "R-Plot 9": Mouse Leave {
        n711 = event-data() -> ()  [unwired: 1 in, 4 out]
        n712 = local write "LMB Down"(FALSE ("Mouse down")) -> ()
      }
      event "R-Plot 0", "R-Plot 1", "R-Plot 2", "R-Plot 3", "R-Plot 4", "R-Plot 5", "R-Plot 6", "R-Plot 7", "R-Plot 8", "R-Plot 9": Scale Range Change {
        w993 = u8 0 ("X Scale.Scale Fit")
        # "Disable plot autoscaling if the user has changed the scale of the plot manualy"
        n713 = event-data() -> ("CtlRef"=w992:refnum<vi>)  [unwired: 1 in, 7 out]
        n714 = property class="XYGraph (strict)"(reference=w992, "XScale.ScaleFit"=w993, "YScale.ScaleFit"=w993) -> ()  [unwired: 1 in, 2 out]
      }
      event "R-Plot 0", "R-Plot 1", "R-Plot 2", "R-Plot 3", "R-Plot 4", "R-Plot 5", "R-Plot 6", "R-Plot 7", "R-Plot 8", "R-Plot 9": Shortcut Menu Activation? {
        w1001 = string[] ["Log Y"] ("item names")
        w1003 = string[] ["Zoom In to Last Data", "Autoscale XY"] ("item names")
        # "Add extra options to the plots context menu"
        n715 = event-data() -> ("MenuRef"=w1005:refnum<k9>, "CtlRef"=w997:refnum<vi>)  [unwired: 1 in]
        n716 = Insert Menu Items(4:10, 7:w1003, 8:w1003, 9:w1005) -> (3:w999:refnum<k9>)  [unwired: 2 in, 2 out]
        n717 = property class="XYGraph (strict)"(reference=w997) -> ("YScale.Mapping Mode"=w996:u8)  [unwired: 1 in, 2 out]
        n718 = Insert Menu Items(4:14, 7:w1001, 8:w1001, 9:w999) -> (3:w998:refnum<k9>)  [unwired: 2 in, 2 out]
        n719 = Not Equal To 0?(x=w996) -> (x != 0?=w995:bool)
        n720 = Set Menu Item Info(6:w995, 7:"Log Y", 11:w998) -> ()  [unwired: 4 in, 2 out]
        n721 = local read "LMB Down"() -> (w1002:bool)
        n722 = event-data("Discard?"=w1002) -> ()  [unwired: 1 in, 1 out]
      }
      event "R-Plot 0", "R-Plot 1", "R-Plot 2", "R-Plot 3", "R-Plot 4", "R-Plot 5", "R-Plot 6", "R-Plot 7", "R-Plot 8", "R-Plot 9": Shortcut Menu Selection (User) {
        # "Zoom in to last \"Miniplot points\". Zoom out a bit to have some space around the points"
        n723 = event-data() -> ("CtlRef"=w1009:refnum<vi>, "ItemTag"=w1007:string)  [unwired: 1 in]
        n724 = Type Cast(type=refnum<vi> refnum ("R-Plot 0"), x=w1009) -> (*(type *) &x=w1008:refnum<vi>)
        n725 = case shown="\"Zoom In to Last Data\"" w1007 {
          tunnel: w1008 -> [_ w1011 w1040 w1046]
          frame Default {
          }
          frame "Autoscale XY" {
            w1010 = u8 2 ("X Scale.Scale Fit")
            n726 = property class="XYGraph (strict)"(reference=w1011, "XScale.ScaleFit"=w1010, "YScale.ScaleFit"=w1010) -> ()  [unwired: 1 in, 2 out]
          }
          frame "Zoom In to Last Data" {
            w1036 = u8 0 ("Y Scale.Scale Fit")
            n727 = property on="AVS Runtime Settings" class="Clust (strict)"() -> ("Value"=w1035:T17)  [unwired: 2 in, 2 out]
            n728 = property class="XYGraph (strict)"(reference=w1040) -> (reference out=w1037:refnum<vi>, "Value"=w1039:cluster{dbl[], dbl[]})  [unwired: 1 in, 1 out]
            n729 = Unbundle By Name(w1035) -> ("Data Memory 2"=w1034:dbl)
            n730 = Unbundle(w1039) -> (w1013:dbl[], w1038:dbl[])
            n731 = Multiply(x=w1034, y=60.0) -> (x*y=w1030:dbl)
            n732 = Reverse 1D Array(array=w1013) -> (reversed array=w1018:dbl[])
            n733 = Reverse 1D Array(array=w1038) -> (reversed array=w1026:dbl[])
            n734 = Index Array(array=w1018) -> (element=w1032:dbl)  [unwired: 1 in]
            n735 = Multiply(x=0.5, y=w1030) -> (x*y=w1031:dbl)
            n736 = Add(x=w1031, y=w1032) -> (x+y=w1029:dbl)
            n737 = Subtract(x=w1032, y=w1030) -> (x-y=w1027:dbl)
            n738 = call "Improved Threshold Detector.71.vi"("Threshold"=w1027, "Array"=w1013) -> ("Positive transition indices"=w1014:i32[])  [unwired: 8 in, 1 out]
            n739 = Index Array(array=w1014) -> (element=w1041:i32)  [unwired: 1 in]
            n740 = Array Size(array=w1013) -> (size(s)=w1016:i32)
            n741 = Index Array(array=w1013, index=w1041) -> (element=w1012:dbl)
            n742 = Subtract(x=w1016, y=w1041) -> (x-y=w1015:i32)
            n743 = Array Subset(array=w1026, length=w1015) -> (w1025:dbl[])  [unwired: 1 in]
            n744 = Array Max & Min(array=w1025) -> (max value=w1022:dbl, min value=w1021:dbl)  [unwired: 2 out]
            n745 = Subtract(x=w1022, y=w1021) -> (x-y=w1024:dbl)
            n746 = Divide(x=w1024, y=2.0) -> (x/y=w1020:dbl)
            n747 = Add(x=w1022, y=w1020) -> (x+y=w1017:dbl)
            n748 = Subtract(x=w1021, y=w1020) -> (x-y=w1019:dbl)
            n749 = property class="XYGraph (strict)"(reference=w1037, "XScale.ScaleFit"=w1036, "YScale.ScaleFit"=w1036, "XScale.Maximum"=w1029, "XScale.Minimum"=w1012, "YScale.Maximum"=w1017, "YScale.Minimum"=w1019) -> ()  [unwired: 1 in, 2 out]
          }
          frame "Log Y" {
            n750 = property class="XYGraph (strict)"(reference=w1046) -> (reference out=w1045:refnum<vi>, "YScale.Mapping Mode"=w1044:u8)  [unwired: 1 in, 1 out]
            n751 = Equal To 0?(x=w1044) -> (x = 0?=w1043:bool)
            n752 = Boolean To (0,1)(Boolean=w1043) -> (0, 1=w1042:i16)
            n753 = property class="XYGraph (strict)"(reference=w1045, "YScale.Mapping Mode"=w1042) -> ()  [unwired: 1 in, 2 out]
          }
        }
      }
      event "PID-Plot": Shortcut Menu Activation? {
        w1054 = string[] ["Log Y"] ("item names")
        w1056 = string[] ["Autoscale XY"] ("item names")
        # "Add extra options to the plots context menu"
        n754 = event-data() -> ("MenuRef"=w1058:refnum<k9>, "CtlRef"=w1050:refnum<vi>)  [unwired: 1 in]
        n755 = Insert Menu Items(4:8, 7:w1056, 8:w1056, 9:w1058) -> (3:w1052:refnum<k9>)  [unwired: 2 in, 2 out]
        n756 = property class="WFChart (strict)"(reference=w1050) -> ("YScale.Mapping Mode"=w1049:u8)  [unwired: 1 in, 2 out]
        n757 = Insert Menu Items(4:11, 7:w1054, 8:w1054, 9:w1052) -> (3:w1051:refnum<k9>)  [unwired: 2 in, 2 out]
        n758 = Not Equal To 0?(x=w1049) -> (x != 0?=w1048:bool)
        n759 = Set Menu Item Info(6:w1048, 7:"Log Y", 11:w1051) -> ()  [unwired: 4 in, 2 out]
        n760 = local read "LMB Down"() -> (w1055:bool)
        n761 = event-data("Discard?"=w1055) -> ()  [unwired: 1 in, 1 out]
      }
      event "PID-Plot": Shortcut Menu Selection (User) {
        # "Zoom in to last \"Miniplot points\". Zoom out a bit to have some space around the points"
        n762 = event-data() -> ("CtlRef"=w1061:refnum<vi>, "ItemTag"=w1059:string)  [unwired: 1 in]
        n763 = Type Cast(type=refnum<vi> refnum ("R-Plot 0"), x=w1061) -> (*(type *) &x=w1060:refnum<vi>)
        n764 = case shown="\"Zoom In to Last Data\"" w1059 {
          tunnel: w1060 -> [_ w1064 w1093 w1099]
          frame Default {
          }
          frame "Autoscale XY" {
            w1063 = u8 2 ("X Scale.Scale Fit")
            n765 = property class="XYGraph (strict)"(reference=w1064, "XScale.ScaleFit"=w1063, "YScale.ScaleFit"=w1063) -> ()  [unwired: 1 in, 2 out]
          }
          frame "Zoom In to Last Data" {
            w1089 = u8 0 ("Y Scale.Scale Fit")
            n766 = property on="AVS Runtime Settings" class="Clust (strict)"() -> ("Value"=w1088:T17)  [unwired: 2 in, 2 out]
            n767 = property class="XYGraph (strict)"(reference=w1093) -> (reference out=w1090:refnum<vi>, "Value"=w1092:cluster{dbl[], dbl[]})  [unwired: 1 in, 1 out]
            n768 = Unbundle By Name(w1088) -> ("Data Memory 2"=w1087:dbl)
            n769 = Unbundle(w1092) -> (w1066:dbl[], w1091:dbl[])
            n770 = Multiply(x=w1087, y=60.0) -> (x*y=w1083:dbl)
            n771 = Reverse 1D Array(array=w1066) -> (reversed array=w1071:dbl[])
            n772 = Reverse 1D Array(array=w1091) -> (reversed array=w1079:dbl[])
            n773 = Index Array(array=w1071) -> (element=w1085:dbl)  [unwired: 1 in]
            n774 = Multiply(x=0.5, y=w1083) -> (x*y=w1084:dbl)
            n775 = Add(x=w1084, y=w1085) -> (x+y=w1082:dbl)
            n776 = Subtract(x=w1085, y=w1083) -> (x-y=w1080:dbl)
            n777 = call "Improved Threshold Detector.71.vi"("Threshold"=w1080, "Array"=w1066) -> ("Positive transition indices"=w1067:i32[])  [unwired: 8 in, 1 out]
            n778 = Index Array(array=w1067) -> (element=w1094:i32)  [unwired: 1 in]
            n779 = Array Size(array=w1066) -> (size(s)=w1069:i32)
            n780 = Index Array(array=w1066, index=w1094) -> (element=w1065:dbl)
            n781 = Subtract(x=w1069, y=w1094) -> (x-y=w1068:i32)
            n782 = Array Subset(array=w1079, length=w1068) -> (w1078:dbl[])  [unwired: 1 in]
            n783 = Array Max & Min(array=w1078) -> (max value=w1075:dbl, min value=w1074:dbl)  [unwired: 2 out]
            n784 = Subtract(x=w1075, y=w1074) -> (x-y=w1077:dbl)
            n785 = Divide(x=w1077, y=2.0) -> (x/y=w1073:dbl)
            n786 = Add(x=w1075, y=w1073) -> (x+y=w1070:dbl)
            n787 = Subtract(x=w1074, y=w1073) -> (x-y=w1072:dbl)
            n788 = property class="XYGraph (strict)"(reference=w1090, "XScale.ScaleFit"=w1089, "YScale.ScaleFit"=w1089, "XScale.Maximum"=w1082, "XScale.Minimum"=w1065, "YScale.Maximum"=w1070, "YScale.Minimum"=w1072) -> ()  [unwired: 1 in, 2 out]
          }
          frame "Log Y" {
            n789 = property class="XYGraph (strict)"(reference=w1099) -> (reference out=w1098:refnum<vi>, "YScale.Mapping Mode"=w1097:u8)  [unwired: 1 in, 1 out]
            n790 = Equal To 0?(x=w1097) -> (x = 0?=w1096:bool)
            n791 = Boolean To (0,1)(Boolean=w1096) -> (0, 1=w1095:i16)
            n792 = property class="XYGraph (strict)"(reference=w1098, "YScale.Mapping Mode"=w1095) -> ()  [unwired: 1 in, 2 out]
          }
        }
      }
      event "uPlots.uPlot 0", "uPlots.uPlot 1", "uPlots.uPlot 2", "uPlots.uPlot 3", "uPlots.uPlot 4", "uPlots.uPlot 5", "uPlots.uPlot 6", "uPlots.uPlot 7", "uPlots.uPlot 8", "uPlots.uPlot 9": Mouse Down {
        # "Switch to big plot on double click on small plot"
        n793 = event-data() -> ("Mods.Double Click"=w1101:bool, "CtlRef"=w1100:refnum<vi>)  [unwired: 1 in]
        n794 = case shown="True" w1101 {
          tunnel: w1100 -> [_ w1104]
          frame False {
          }
          frame True {
            n795 = property class="XYGraph (strict)"(reference=w1104) -> ("Label.Text"=w1105:string)  [unwired: 1 in, 2 out]
            n796 = Reverse String(1:w1105) -> (0:w1106:string)
            n797 = Decimal String To Number(string=w1106, default (0L)=8 ("default (0 I32)")) -> (number=w1103:i32)  [unwired: 1 in, 1 out]
            n798 = property on="Channel Controls" class="TabCtl (strict)"("Val(Sgnl)"=w1103) -> ()  [unwired: 2 in, 2 out]
          }
        }
      }
      event "Erase All": Value Change {
        # "Clear data array.\nReset PID."
        n799 = event-data() -> ()  [unwired: 1 in, 6 out]
        n800 = local read "Channel Controls"() -> (w1109:T3)
        n801 = local read "Data"() -> (w1110:cluster{"R":dbl[], "T":dbl[], "Time":dbl[]}[])
        n802 = Replace Array Subset(array=w1110, new element=cluster{"R":dbl[], "T":dbl[], "Time":dbl[]} {"R"=[], "T"=[], "Time"=[]} ("new element/subarray"), index=w1109) -> (w1108:cluster{"R":dbl[], "T":dbl[], "Time":dbl[]}[])
        n803 = local write "Data"(w1108) -> ()
        n804 = disable-structure shown="Disabled" {
          frame Disabled {
            n805 = Initialize Array(cluster{"R":dbl[], "T":dbl[], "Time":dbl[]} {"R"=[], "T"=[], "Time"=[]}, 10 ("dimension size")) -> ()  [unwired: 1 out]
          }
          frame Enabled {
          }
        }
      }
      event "Clear all plots": Value Change {
        n806 = event-data() -> ()  [unwired: 1 in, 6 out]
        n807 = Initialize Array(cluster{"R":dbl[], "T":dbl[], "Time":dbl[]} {"R"=[], "T"=[], "Time"=[]}, 10 ("dimension size")) -> (w1114:cluster{"R":dbl[], "T":dbl[], "Time":dbl[]}[])
        n808 = local write "Data"(w1114) -> ()
      }
      event "Bridge settings.AVS type": Value Change {
        # "Select bridge type (AVS/zBridge). Show/hide corresponding controls."
        n809 = event-data() -> ("NewVal"=w1117:T35)  [unwired: 1 in, 5 out]
        n810 = flat-sequence {
          tunnel: w1117 -> [w1123]
          frame #0 {
            w1119 = u8 0 ("Disabled")
            w1122 = u8 0 ("Disabled")
            w1121 = FALSE ("Visible")
            w1120 = u8 2 ("Disabled")
            n811 = property on="AVS_SPort" class="VISAName"("Visible"=w1121, "Disabled"=w1120) -> ()  [unwired: 2 in, 2 out]
            n812 = property on="Save Screen Data 2" class="Bool"("Visible"=w1121, "Disabled"=w1120) -> ()  [unwired: 2 in, 2 out]
            n813 = property on="Tab Control 5" class="TabCtl (strict)"("Disabled"=w1119) -> ()  [unwired: 2 in, 2 out]
            n814 = property on="Address" class="VISAName"("Visible"=w1121, "Disabled"=w1120) -> ()  [unwired: 2 in, 2 out]
            n815 = property on="Tab Control" class="TabCtl (strict)"("Disabled"=w1119) -> ()  [unwired: 2 in, 2 out]
            n816 = property on="Read AVS channels from" class="DigNum (strict)"("Disabled"=w1122) -> ()  [unwired: 2 in, 2 out]
            n817 = property on="Last Channel" class="DigNum (strict)"("Disabled"=w1122) -> ()  [unwired: 2 in, 2 out]
            n818 = property on="Stabilisation Delay" class="DigNum (strict)"("Disabled"=w1122) -> ()  [unwired: 2 in, 2 out]
            n819 = property on="Averages" class="DigNum (strict)"("Disabled"=w1122) -> ()  [unwired: 2 in, 2 out]
            n820 = property on="Delay Between Scans" class="DigNum (strict)"("Disabled"=w1122) -> ()  [unwired: 2 in, 2 out]
          }
          frame #1 {
            n821 = case shown="\"Disabled\", Default" w1123 {
              frame "AVS47A (GPIB interface)" {
                n822 = local write "Scan Parameters"(enum32{"Page 1", "Page 2"}."Page 1" ("Scan Parameters")) -> ()
                n823 = property on="Address" class="VISAName"("Visible"=TRUE, "Disabled"=u8 0) -> ()  [unwired: 2 in, 2 out]
              }
              frame "AVS47B (RS232 interface)" {
                w1127 = u8 2 ("Disabled")
                n824 = local write "Scan Parameters"(enum32{"Page 1", "Page 2"}."Page 1" ("Scan Parameters")) -> ()
                n825 = property on="AVS_SPort" class="VISAName"("Visible"=TRUE, "Disabled"=u8 0) -> ()  [unwired: 2 in, 2 out]
                n826 = property on="Read AVS channels from" class="DigNum (strict)"("Disabled"=w1127) -> ()  [unwired: 2 in, 2 out]
                n827 = property on="Last Channel" class="DigNum (strict)"("Disabled"=w1127) -> ()  [unwired: 2 in, 2 out]
              }
              frame "AVS48" {
                w1131 = u8 2 ("Disabled")
                n828 = local write "Scan Parameters"(enum32{"Page 1", "Page 2"}."Page 1" ("Scan Parameters")) -> ()
                n829 = property on="AVS_SPort" class="VISAName"("Visible"=TRUE, "Disabled"=u8 0) -> ()  [unwired: 2 in, 2 out]
                n830 = property on="Read AVS channels from" class="DigNum (strict)"("Disabled"=w1131) -> ()  [unwired: 2 in, 2 out]
                n831 = property on="Last Channel" class="DigNum (strict)"("Disabled"=w1131) -> ()  [unwired: 2 in, 2 out]
              }
              frame "AVS Emulation" {
                n832 = local write "Scan Parameters"(enum32{"Page 1", "Page 2"}."Page 1" ("Scan Parameters")) -> ()
              }
              frame "Impedance Bridge" {
                w1138 = u8 2 ("Disabled")
                n833 = local write "Scan Parameters"(enum32{"Page 1", "Page 2"}."Page 2" ("Scan Parameters")) -> ()
                n834 = property on="Save Screen Data 2" class="Bool"("Visible"=TRUE, "Disabled"=u8 0) -> ()  [unwired: 2 in, 2 out]
                n835 = property on="Read AVS channels from" class="DigNum (strict)"("Disabled"=w1138) -> ()  [unwired: 2 in, 2 out]
                n836 = property on="Last Channel" class="DigNum (strict)"("Disabled"=w1138) -> ()  [unwired: 2 in, 2 out]
                n837 = property on="Stabilisation Delay" class="DigNum (strict)"("Disabled"=w1138) -> ()  [unwired: 2 in, 2 out]
                n838 = property on="Averages" class="DigNum (strict)"("Disabled"=w1138) -> ()  [unwired: 2 in, 2 out]
                n839 = property on="Delay Between Scans" class="DigNum (strict)"("Disabled"=w1138) -> ()  [unwired: 2 in, 2 out]
              }
              frame "Disabled", Default {
                w1140 = u8 2 ("Disabled")
                n840 = property on="Tab Control 5" class="TabCtl (strict)"("Disabled"=w1140) -> ()  [unwired: 2 in, 2 out]
                n841 = property on="Tab Control" class="TabCtl (strict)"("Disabled"=w1140) -> ()  [unwired: 2 in, 2 out]
              }
            }
          }
        }
      }
      event "AVS Runtime Settings.Plot type": Value Change {
        # "Iterate through first 10 pages (plots only)"
        # "Switch between RxTime and TxTime plots"
        n842 = event-data() -> ("NewVal"=w1149:enum16{"R vs Time", "T vs Time"})  [unwired: 1 in, 5 out]
        n843 = Equal To 0?(x=w1149) -> (x = 0?=w1148:bool)
        n844 = Select(t=u32 10532351, s=w1148, f=u32 16711680) -> (s? t:f=w1145:u32)
        n845 = property on="uPlots" class="Clust (strict)"() -> ("Controls[]"=w1143:refnum<vi>[])  [unwired: 2 in, 2 out]
        n846 = property on="Channel Controls" class="TabCtl (strict)"() -> ("Pages"=w1150:refnum<vi>[])  [unwired: 2 in, 2 out]
        n847 = for {
          N: 10 -> [_]
          tunnel: w1150 -> [w1160] mode=indexing
          tunnel: w1145 -> [w1153]
          tunnel: w1143 -> [w1151] mode=indexing
          # "!!NOTE:This routine assumes that graph is control #0 on page!!"
          n848 = property class="Page"(reference=w1160) -> ("ControlsOnPage"=w1158:refnum<vi>[])  [unwired: 1 in, 2 out]
          n849 = Type Cast(type=refnum<vi> refnum ("R-Plot 0"), x=w1151) -> (*(type *) &x=w1152:refnum<vi>)
          n850 = Index Array(array=w1158, index=0) -> (element=w1156:refnum<vi>)
          n851 = Type Cast(type=refnum<vi> refnum ("R-Plot 0"), x=w1156) -> (*(type *) &x=w1155:refnum<vi>)
          n852 = property class="XYGraph (strict)"(reference=w1152, "Plot.Plot Color"=w1153, "Plot.Fill/Pt. Color"=w1153) -> ()  [unwired: 1 in, 2 out]
          n853 = property class="XYGraph (strict)"(reference=w1155, "Plot.Plot Color"=w1153, "Plot.Fill/Pt. Color"=w1153) -> ()  [unwired: 1 in, 2 out]
        }
        n854 = property on="ResetPIDloop" class="TypRef (strict)"() -> ("Value"=w1142:refnum<user-event>)  [unwired: 2 in, 2 out]
        n855 = Generate User Event(user event=w1142, event data cluster="" ("event data")) -> ()  [unwired: 2 in, 2 out]
      }
      event "AVS Runtime Settings.Read AVS channels from", "AVS Runtime Settings.Last Channel": Value Change {
        # "Change enabled channels for the AVS bridge"
        n856 = event-data() -> ()  [unwired: 1 in, 6 out]
        n857 = local read "UpdateChannelInfo"() -> (w1162:refnum<user-event>)
        n858 = Generate User Event(user event=w1162, event data cluster=bool[] [] ("event data")) -> ()  [unwired: 2 in, 2 out]
      }
      event "AVS Runtime Settings.Filter graphs:": Value Change {
        # "Graph filtering controls"
        n859 = event-data() -> ("NewVal"=w1163:bool)  [unwired: 1 in, 5 out]
        n860 = call "IsDisabled.vi"("Enabled?"=w1163) -> ("Numeric"=w1164:i16)
        n861 = property on="Y_min" class="DigNum (strict)"("Disabled"=w1164) -> ()  [unwired: 2 in, 2 out]
        n862 = property on="Y_max" class="DigNum (strict)"("Disabled"=w1164) -> ()  [unwired: 2 in, 2 out]
      }
      event "Channel Controls": Value Change {
        # "Show hide bottom Tesistance/Temperature panel depending on the current tab page"
        n863 = event-data() -> ("NewVal"=w1165:T3)  [unwired: 1 in, 5 out]
        n864 = case shown="Default" w1165 {
          frame Default {
            n865 = property on="Mode Buttons" class="RadioBtnsControl (strict)"() -> ("Value"=w1166:T13)  [unwired: 2 in, 2 out]
            n866 = property on="Data History" class="TabCtl (strict)"("Value"=enum32{"History", "Settings"}."History" ("Data History")) -> ()  [unwired: 2 in, 2 out]
            n867 = property on="Mode Buttons" class="RadioBtnsControl (strict)"("Val(Sgnl)"=w1166) -> ()  [unwired: 2 in, 2 out]
          }
          frame "All" {
            n868 = property on="Data History" class="TabCtl (strict)"("Value"=enum32{"History", "Settings"}."Settings" ("Data History")) -> ()  [unwired: 2 in, 2 out]
          }
        }
      }
      event "Thermometer": Value Change {
        # "Calibration changed - update calibrations list"
        n869 = event-data() -> ()  [unwired: 1 in, 6 out]
        n870 = property on="Thermometer" class="Clust (strict)"() -> ("Controls[]"=w1171:refnum<vi>[])  [unwired: 2 in, 2 out]
        n871 = Array Size(array=w1171) -> (size(s)=w1172:i32)
        n872 = for {
          N: w1172 -> [_]
          tunnel: w1171 -> [w1176] mode=indexing
          tunnel: [w1173] -> w1170 mode=indexing
          w1175 = refnum<vi> refnum  # Ring
          n873 = Type Cast(type=w1175, x=w1176) -> (*(type *) &x=w1174:refnum<vi>)
          n874 = property class="Ring"(reference=w1174) -> ("RingText.Text"=w1173:string)  [unwired: 1 in, 2 out]
        }
        n875 = Array To Cluster(array=w1170) -> (cluster=→"CurCalibrations":T23)
      }
      event User Event; "Data logging": Value Change {
        # "Log file settings changed. Generate new log file name"
        n876 = event-data() -> ()  [unwired: 1 in, 3 out]
        n877 = local read "Data logging"() -> (w1184:T27)
        n878 = Unbundle By Name(w1184) -> ("Run description"=w1178:string, "Filenames suffix"=w1179:string, "AVS_Path"=w1185:path, "AVS_FName"=w1183:string, "CAL_FName"=w1182:string)
        n879 = local write "LogFileCreationTime"(timestamp(2742897600 s since 1904-01-01)) -> ()
        n880 = call "MGI Make String Filesafe.vi"("String In"=w1178) -> ("Filesafe String Out"=w1177:string)
        n881 = call "GeneratePaths.vi"("Filename Suffix"=w1179, "Run description"=w1177, "AVS_Path"=w1185, "AVS_FName"=w1183, "CAL_Path"=w1185, "CAL_FName"=w1182) -> ("Generated Log path"=w1181:path, "Generated Calib path"=w1180:path)  [unwired: 8 in]
        n882 = local write "Log path"(w1181) -> ()
        n883 = local write "Calib path"(w1180) -> ()
      }
      event "Convert": Mouse Down; "QuickR": Value Change {
        # "Quick convert R->T"
        n884 = event-data() -> ()  [unwired: 1 in, 4 out]
        n885 = property on="Select sensor 1" class="Ring (strict)"() -> ("Strings []"=w1189:string[], "Value"=w1190:u16)  [unwired: 2 in, 2 out]
        n886 = property on="AVS_CalFolder" class="Path"() -> ("Value"=w1187:path)  [unwired: 2 in, 2 out]
        n887 = Index Array(array=w1189, index=w1190) -> (element=w1188:string)
        n888 = call "SelectSensor-txt no ext.vi"("Path"=w1187, "Resistance"="QuickR", "Select sensor"=w1188) -> ("Temperature"=→"T7":dbl)  [unwired: 1 out]
      }
      event "T Sweep.Current": Value Change {
        # "Current/ Setpoint value is changed"
        n889 = event-data() -> ("NewVal"=→"I3_SetPnt":dbl)  [unwired: 1 in, 5 out]
        n890 = property on="ResetPIDloop" class="TypRef (strict)"() -> ("Value"=w1194:refnum<user-event>)  [unwired: 2 in, 2 out]
        n891 = Generate User Event(user event=w1194, event data cluster="" ("event data")) -> ()  [unwired: 2 in, 2 out]
      }
      event "Automode 2": Value Change {
        n892 = event-data() -> ("NewVal"=w1196:bool)  [unwired: 1 in, 5 out]
        n893 = case shown="True" w1196 {
          frame False {
          }
          frame True {
            # "Set timer to zero (01-01-1904) so the first point is set immediately, w/o wainting for time delay."
            # "If automatic mode is enabled- fire TempStabilized event to record current R,T,I values and start sweeping through TCS channels arrays"
            n894 = disable-structure shown="Disabled" {
              frame Disabled {
                n895 = Generate User Event(event data cluster="" ("event data")) -> ()  [unwired: 3 in, 2 out]
                "Time Old" <- 0.0 ("Timer")
              }
              frame Enabled {
              }
            }
          }
        }
      }
      event "CS Mode": Value Change {
        # "Changed Channel1 automatic mode"
        n896 = event-data() -> ()  [unwired: 1 in, 6 out]
        n897 = property on="CS Mode" class="Enum (strict)"() -> ("Value"=w1200:enum16{"Manual", "Automatic"})  [unwired: 2 in, 2 out]
        n898 = case shown="\"Automatic\"" w1200 {
          tunnel: [TRUE ("Automatic mode ON") FALSE ("Automatic mode ON")] -> w1199
          frame "Automatic" {
            w1208 = TRUE
            # "Set automatic mode currents equal to last manual values. Switch on the current sources."
            n899 = local read "I"() -> (w1217:dbl[])
            n900 = property on="ON" class="Bool (strict)"() -> ("Value"=w1212:bool)  [unwired: 2 in, 2 out]
            n901 = property on="ON" class="Bool (strict)"() -> ("Value"=w1211:bool)  [unwired: 2 in, 2 out]
            n902 = property on="ON" class="Bool (strict)"() -> ("Value"=w1210:bool)  [unwired: 2 in, 2 out]
            n903 = property on="ON" class="Bool (strict)"() -> ("Value"=w1209:bool)  [unwired: 2 in, 2 out]
            n904 = property on="FB on 2" class="Enum (strict)"() -> ("Value"=w1203:enum16{"0", "1", "2", "3"})  [unwired: 2 in, 2 out]
            n905 = Multiply(x=1000.0, y=w1217) -> (x*y=w1204:dbl[])
            n906 = Exclusive Or(1:w1212, 2:w1208) -> (0:w1216:bool)
            n907 = Exclusive Or(1:w1211, 2:w1208) -> (0:w1214:bool)
            n908 = Exclusive Or(1:w1210, 2:w1208) -> (0:w1213:bool)
            n909 = Exclusive Or(1:w1209, 2:w1208) -> (0:w1215:bool)
            n910 = Index Array(array=w1204, index=w1203) -> (element=w1202:dbl)
            n911 = local write "I_in"(w1204) -> ()
            n912 = property on="Toggle ON/OFF" class="Bool (strict)"("Value"=w1216) -> ()  [unwired: 2 in, 2 out]
            n913 = property on="Toggle ON/OFF" class="Bool (strict)"("Value"=w1214) -> ()  [unwired: 2 in, 2 out]
            n914 = property on="Toggle ON/OFF" class="Bool (strict)"("Value"=w1213) -> ()  [unwired: 2 in, 2 out]
            n915 = property on="Toggle ON/OFF" class="Bool (strict)"("Value"=w1215) -> ()  [unwired: 2 in, 2 out]
            n916 = property on="I_0" class="DigNum (strict)"("Value"=w1202) -> ()  [unwired: 2 in, 2 out]
            n917 = property on="TempStabilized" class="TypRef (strict)"() -> ("Value"=w1207:refnum<user-event>)  [unwired: 2 in, 2 out]
            n918 = Generate User Event(user event=w1207, event data cluster=FALSE ("event data")) -> ()  [unwired: 2 in, 2 out]
          }
          frame "Manual" {
            # "Set manual mode currents \nequal to last automode \nvalues."
            n919 = local read "I_in"() -> (w1219:dbl[])
            n920 = Index Array(array=w1219) -> (element #1=w1223:dbl, element #2=w1222:dbl, element #3=w1221:dbl, element #4=w1220:dbl)  [unwired: 4 in]
            n921 = property on="I0" class="DigNum (strict)"("Val(Sgnl)"=w1223) -> ()  [unwired: 2 in, 2 out]
            n922 = property on="I1" class="DigNum (strict)"("Val(Sgnl)"=w1222) -> ()  [unwired: 2 in, 2 out]
            n923 = property on="I2" class="DigNum (strict)"("Val(Sgnl)"=w1221) -> ()  [unwired: 2 in, 2 out]
            n924 = property on="I3" class="DigNum (strict)"("Val(Sgnl)"=w1220) -> ()  [unwired: 2 in, 2 out]
          }
        }
        "Automatic mode 1" <- w1199
        "Automatic mode 2" <- w1199
        "Automatic mode 3" <- w1199
        "Automatic mode 0" <- w1199
      }
      event "Next step": Value Change {
        # "Go to next step in CS auto mode."
        n925 = event-data() -> ()  [unwired: 1 in, 6 out]
        n926 = flat-sequence {
          frame #0 {
            n927 = Get Date/Time In Seconds() -> (seconds since 1Jan1904=w1225:timestamp)
            n928 = To Double Precision Float(number=w1225) -> (double precision float=w1226:dbl)
            n929 = local write "Time Old"(w1226) -> ()
          }
          frame #1 {
            n930 = property on="TempStabilized" class="TypRef (strict)"() -> ("Value"=w1228:refnum<user-event>)  [unwired: 2 in, 2 out]
            n931 = Generate User Event(user event=w1228, event data cluster=TRUE ("event data")) -> ()  [unwired: 2 in, 2 out]
          }
        }
      }
      event "Data logging.External VI path": Value Change {
        # "Set path for the external VI to call on TempStabilised event"
        n932 = event-data() -> ("NewVal"=w1230:path)  [unwired: 1 in, 5 out]
        n933 = vi-ref "OnTempStabilizedRef.vi"() -> (w1231:refnum<vi>)
        n934 = Open VI Reference(type specifier VI Refnum (for type only)=w1231, vi path=w1230) -> (vi reference=w1229:refnum<vi>)  [unwired: 4 in, 1 out]
        n935 = local write "vi reference"(w1229) -> ()
      }
      event "Autorange": Value Change {
        # "Disabled"
        n936 = event-data() -> ("NewVal"=w1232:bool)  [unwired: 1 in, 5 out]
        n937 = Boolean To (0,1)(Boolean=w1232) -> (0, 1=w1235:i16)
        n938 = Multiply(x=i16 2, y=w1235) -> (x*y=w1233:i16)
        n939 = property on="Ranges" class="Clust (strict)"("Disabled"=w1233) -> ()  [unwired: 2 in, 2 out]
      }
      event "Current source settings.CS type": Value Change {
        # "Set CS type"
        n940 = event-data() -> ("NewVal"=w1236:T36)  [unwired: 1 in, 5 out]
        n941 = flat-sequence {
          tunnel: w1236 -> [w1263]
          frame #0 {
            w1248 = u8 2 ("Disabled")
            w1243 = u8 0 ("Disabled")
            w1258 = TRUE ("Visible")
            n942 = control-ref of="Current indicators"() -> (w1244:refnum<vi>)
            n943 = control-ref of="I0"() -> (w1255:refnum<vi>)
            n944 = control-ref of="I1"() -> (w1247:refnum<vi>)
            n945 = control-ref of="C_I0"() -> (w1254:refnum<vi>)
            n946 = control-ref of="C_I1"() -> (w1246:refnum<vi>)
            n947 = control-ref of="I2"() -> (w1242:refnum<vi>)
            n948 = control-ref of="I3"() -> (w1241:refnum<vi>)
            n949 = control-ref of="CS Mode"() -> (w1245:refnum<vi>)
            n950 = control-ref of="Map Channel 0 to 2"() -> (w1253:refnum<vi>)
            n951 = property class="TabCtl (strict)"(reference=w1244, "Disabled"=w1243) -> ()  [unwired: 1 in, 2 out]
            n952 = property class="Clust (strict)"(reference=w1255, "Disabled"=w1243) -> ()  [unwired: 1 in, 2 out]
            n953 = property class="Clust (strict)"(reference=w1247, "Disabled"=w1243) -> ()  [unwired: 1 in, 2 out]
            n954 = property class="Clust (strict)"(reference=w1242, "Disabled"=w1243) -> ()  [unwired: 1 in, 2 out]
            n955 = property class="Clust (strict)"(reference=w1241, "Disabled"=w1243) -> ()  [unwired: 1 in, 2 out]
            n956 = property class="Clust (strict)"(reference=w1254, "Disabled"=w1243) -> ()  [unwired: 1 in, 2 out]
            n957 = property class="Clust (strict)"(reference=w1246, "Disabled"=w1243) -> ()  [unwired: 1 in, 2 out]
            n958 = property class="Enum (strict)"(reference=w1253, "Disabled"=w1243) -> ()  [unwired: 1 in, 2 out]
            n959 = property class="Enum (strict)"(reference=w1245, "Disabled"=w1243) -> ()  [unwired: 1 in, 2 out]
            n960 = control-ref of="TCS_Port"() -> (w1257:refnum<vi>)
            n961 = property on="Tab Control 2" class="TabCtl (strict)"() -> ("Pages"=w1237:refnum<vi>[])  [unwired: 2 in, 2 out]
            n962 = Index Array(array=w1237, index=1) -> (element=w1238:refnum<vi>)
            n963 = control-ref of="Toggle Gated"() -> (w1249:refnum<vi>)
            n964 = control-ref of="Toggle Gated"() -> (w1250:refnum<vi>)
            n965 = control-ref of="Toggle Gated"() -> (w1251:refnum<vi>)
            n966 = control-ref of="Toggle Gated"() -> (w1252:refnum<vi>)
            n967 = control-ref of="QCS/PCS Device"() -> (w1260:refnum<vi>)
            n968 = control-ref of="I0 output to"() -> (w1259:refnum<vi>)
            n969 = property class="Page"(reference=w1238, "PageVis"=TRUE ("Page Visible")) -> ()  [unwired: 1 in, 2 out]
            n970 = property class="Bool (strict)"(reference=w1249, "Disabled"=w1248) -> ()  [unwired: 1 in, 2 out]
            n971 = property class="Bool (strict)"(reference=w1250, "Disabled"=w1248) -> ()  [unwired: 1 in, 2 out]
            n972 = property class="Bool (strict)"(reference=w1251, "Disabled"=w1248) -> ()  [unwired: 1 in, 2 out]
            n973 = property class="Bool (strict)"(reference=w1252, "Disabled"=w1248) -> ()  [unwired: 1 in, 2 out]
            n974 = property class="DigNum (strict)"(reference=w1260, "Visible"=w1258) -> ()  [unwired: 1 in, 2 out]
            n975 = property class="Enum (strict)"(reference=w1259, "Visible"=w1258) -> ()  [unwired: 1 in, 2 out]
            n976 = property class="VISAName"(reference=w1257, "Visible"=FALSE) -> ()  [unwired: 1 in, 2 out]
          }
          frame #1 {
            n977 = case shown="\"QCS v1\"" w1263 {
              tunnel: [refnum<class "TCS.lvclass"> refnum ("TCS.lvclass") refnum<class "QCS.lvclass"> refnum ("QCS.lvclass") w1283 w1297 refnum<class "PCS.lvclass"> refnum ("PCS.lvclass")] -> w1262
              tunnel: [w1264 w1282 u16 255 ("Value") u16 255 ("Value") w1302] -> w1261
              frame "TCS" {
                w1267 = u8 2 ("Disabled")
                w1280 = u8 0 ("Disabled")
                n978 = control-ref of="TCS_Port"() -> (w1270:refnum<vi>)
                n979 = control-ref of="Toggle Gated"() -> (w1279:refnum<vi>)
                n980 = control-ref of="Toggle Gated"() -> (w1278:refnum<vi>)
                n981 = control-ref of="Toggle Gated"() -> (w1277:refnum<vi>)
                n982 = control-ref of="Toggle Gated"() -> (w1276:refnum<vi>)
                n983 = control-ref of="QCS/PCS Device"() -> (w1272:refnum<vi>)
                n984 = control-ref of="I0"() -> (w1275:refnum<vi>)
                n985 = control-ref of="C_I0"() -> (w1268:refnum<vi>)
                n986 = control-ref of="Map Channel 0 to 2"() -> (w1269:refnum<vi>)
                n987 = property class="Bool (strict)"(reference=w1279, "Disabled"=w1280) -> ()  [unwired: 1 in, 2 out]
                n988 = property class="Bool (strict)"(reference=w1278, "Disabled"=w1280) -> ()  [unwired: 1 in, 2 out]
                n989 = property class="Bool (strict)"(reference=w1277, "Disabled"=w1280) -> ()  [unwired: 1 in, 2 out]
                n990 = property class="Bool (strict)"(reference=w1276, "Disabled"=w1280) -> ()  [unwired: 1 in, 2 out]
                n991 = property class="Clust (strict)"(reference=w1268, "Disabled"=w1267) -> ()  [unwired: 1 in, 2 out]
                n992 = property class="Clust (strict)"(reference=w1275, "Disabled"=u8 2) -> ()  [unwired: 1 in, 2 out]
                n993 = property class="DigNum (strict)"(reference=w1272, "Visible"=FALSE) -> ()  [unwired: 1 in, 2 out]
                n994 = property class="VISAName"(reference=w1270, "Visible"=TRUE) -> ()  [unwired: 1 in, 2 out]
                n995 = property class="Enum (strict)"(reference=w1269, "Disabled"=w1267) -> ()  [unwired: 1 in, 2 out]
                n996 = property on="TCS_Port" class="VISAName"() -> ("Value"=w1265:refnum<visa-resource-name>)  [unwired: 2 in, 2 out]
                n997 = call "VISA to RS232 Port Nr.vi"("VISA Resource Name"=w1265) -> ("Port Number"=w1264:u8)  [unwired: 1 in]
              }
              frame "QCS v1" {
                n998 = property on="QCS/PCS Device" class="DigNum (strict)"() -> ("Value"=w1282:u16)  [unwired: 2 in, 2 out]
              }
              frame "CS Emulation" {
                w1283 = refnum<class "CS Emulation.lvclass"> refnum  # CS Emulation.lvclass
                n999 = control-ref of="QCS/PCS Device"() -> (w1286:refnum<vi>)
                n1000 = property class="DigNum (strict)"(reference=w1286, "Visible"=FALSE) -> ()  [unwired: 1 in, 2 out]
              }
              frame "Disabled", Default {
                w1287 = u8 2 ("Disabled")
                w1297 = refnum<class "CS Emulation.lvclass"> refnum  # CS Emulation.lvclass
                n1001 = control-ref of="Current indicators"() -> (w1296:refnum<vi>)
                n1002 = control-ref of="I0"() -> (w1291:refnum<vi>)
                n1003 = control-ref of="I1"() -> (w1290:refnum<vi>)
                n1004 = control-ref of="I2"() -> (w1289:refnum<vi>)
                n1005 = control-ref of="I3"() -> (w1288:refnum<vi>)
                n1006 = control-ref of="QCS/PCS Device"() -> (w1300:refnum<vi>)
                n1007 = property class="DigNum (strict)"(reference=w1300, "Visible"=FALSE) -> ()  [unwired: 1 in, 2 out]
                n1008 = property class="Clust (strict)"(reference=w1291, "Disabled"=w1287) -> ()  [unwired: 1 in, 2 out]
                n1009 = property class="Clust (strict)"(reference=w1290, "Disabled"=w1287) -> ()  [unwired: 1 in, 2 out]
                n1010 = property class="Clust (strict)"(reference=w1289, "Disabled"=w1287) -> ()  [unwired: 1 in, 2 out]
                n1011 = property class="Clust (strict)"(reference=w1288, "Disabled"=w1287) -> ()  [unwired: 1 in, 2 out]
                n1012 = property class="TabCtl (strict)"(reference=w1296, "Disabled"=w1287) -> ()  [unwired: 1 in, 2 out]
                n1013 = property on="Tab Control 2" class="TabCtl (strict)"() -> ("Pages"=w1295:refnum<vi>[])  [unwired: 2 in, 2 out]
                n1014 = Index Array(array=w1295, index=1) -> (element=w1294:refnum<vi>)
                n1015 = property class="Page"(reference=w1294, "PageVis"=FALSE ("Page Visible")) -> ()  [unwired: 1 in, 2 out]
              }
              frame "PCS (n.a.)" {
                w1303 = u8 2 ("Disabled")
                n1016 = control-ref of="I0"() -> (w1309:refnum<vi>)
                n1017 = control-ref of="I1"() -> (w1308:refnum<vi>)
                n1018 = control-ref of="C_I0"() -> (w1307:refnum<vi>)
                n1019 = control-ref of="C_I1"() -> (w1306:refnum<vi>)
                n1020 = control-ref of="CS Mode"() -> (w1305:refnum<vi>)
                n1021 = control-ref of="Map Channel 0 to 2"() -> (w1304:refnum<vi>)
                n1022 = property class="Clust (strict)"(reference=w1307, "Disabled"=w1303) -> ()  [unwired: 1 in, 2 out]
                n1023 = property class="Clust (strict)"(reference=w1306, "Disabled"=w1303) -> ()  [unwired: 1 in, 2 out]
                n1024 = property class="Clust (strict)"(reference=w1309, "Disabled"=w1303) -> ()  [unwired: 1 in, 2 out]
                n1025 = property class="Clust (strict)"(reference=w1308, "Disabled"=w1303) -> ()  [unwired: 1 in, 2 out]
                n1026 = property class="Enum (strict)"(reference=w1305, "Disabled"=w1303) -> ()  [unwired: 1 in, 2 out]
                n1027 = property class="Enum (strict)"(reference=w1304, "Disabled"=w1303) -> ()  [unwired: 1 in, 2 out]
                n1028 = property on="QCS/PCS Device" class="DigNum (strict)"() -> ("Value"=w1302:u16)  [unwired: 2 in, 2 out]
              }
            }
            "CS ref" <- w1262
            n1029 = property on="HW Address" class="DigNum (strict)"("Value"=w1261) -> ()  [unwired: 2 in, 2 out]
          }
        }
      }
      event "Current source settings.QCS/PCS Device": Value Change {
        # "Set CS port"
        n1030 = event-data() -> ("NewVal"=w1310:u16)  [unwired: 1 in, 5 out]
        n1031 = property on="CS type" class="Enum (strict)"() -> ("Value"=w1311:T36)  [unwired: 2 in, 2 out]
        n1032 = case shown="\"QCS v1\"" w1311 {
          tunnel: w1310 -> [_ w1314 _]
          frame Default {
          }
          frame "QCS v1" {
            n1033 = Variant To Data(type=u32 255 ("HW Address"), Variant=w1314) -> (data=w1312:u32)  [unwired: 1 in, 1 out]
            n1034 = property on="HW Address" class="DigNum (strict)"("Value"=w1312) -> ()  [unwired: 2 in, 2 out]
          }
          frame "CS Emulation" {
            n1035 = property on="HW Address" class="DigNum (strict)"("Value"=u32 255 ("HW Address")) -> ()  [unwired: 2 in, 2 out]
          }
        }
      }
      event "Current source settings.TCS_Port": Value Change {
        # "Set TCS port"
        n1036 = event-data() -> ("NewVal"=w1316:refnum<visa-resource-name>)  [unwired: 1 in, 5 out]
        n1037 = property on="CS type" class="Enum (strict)"() -> ("Value"=w1317:T36)  [unwired: 2 in, 2 out]
        n1038 = case shown="\"TCS\"" w1317 {
          tunnel: w1316 -> [w1320 _]
          frame "TCS" {
            n1039 = Type Cast(type=refnum<visa-resource-name> refnum ("Value"), x=w1320) -> (*(type *) &x=w1319:refnum<visa-resource-name>)
            n1040 = call "VISA to RS232 Port Nr.vi"("VISA Resource Name"=w1319) -> ("Port Number"=w1321:u8)  [unwired: 1 in]
            n1041 = property on="HW Address" class="DigNum (strict)"("Value"=w1321) -> ()  [unwired: 2 in, 2 out]
          }
          frame Default {
          }
        }
      }
      event "I3 as temp.I3 as temp 2": Value Change {
        # "Enable/disable the PID loop"
        n1042 = event-data() -> ("NewVal"=w1333:bool)  [unwired: 1 in, 5 out]
        n1043 = call "IsDisabled.vi"("Enabled?"=w1333) -> ("Numeric"=w1337:i16)
        n1044 = property on="ResetPIDloop" class="TypRef (strict)"() -> ("Value"=w1336:refnum<user-event>)  [unwired: 2 in, 2 out]
        n1045 = property on="PID setup 2" class="Clust (strict)"("Disabled"=w1337) -> ()  [unwired: 2 in, 2 out]
        n1046 = Generate User Event(user event=w1336, event data cluster="" ("event data")) -> ()  [unwired: 2 in, 2 out]
        n1047 = property on="FB on" class="Enum (strict)"() -> ("Value"=w1330:enum16{"Resistance", "Temperature"})  [unwired: 2 in, 2 out]
        n1048 = property on="FB on 2" class="Enum (strict)"() -> ("Value"=w1329:enum16{"0", "1", "2", "3"})  [unwired: 2 in, 2 out]
        n1049 = property on="I3 as temp 2" class="Bool (strict)"() -> ("Value"=w1323:bool)  [unwired: 2 in, 2 out]
        n1050 = Initialize Array(FALSE, 4 ("dimension size")) -> (w1325:bool[])
        n1051 = And(x=TRUE ("new element/subarray"), y=w1323) -> (x .and. y?=w1322:bool)
        n1052 = Index Array(array=string[] ["%#_g uA", "%#_g mK"], index=w1330) -> (element=w1332:string)
        n1053 = Replace Array Subset(array=w1325, new element=w1322, index=w1329) -> (w1328:bool[])
        n1054 = local write "T Channel"(w1328) -> ()
        n1055 = Select(t=w1332, s=w1333, f="%#_g uA") -> ()  [unwired: 1 out]
      }
      event "Load Data": Value Change {
        # "Load data from log files"
        n1056 = event-data() -> ()  [unwired: 1 in, 6 out]
        n1057 = property on="AVS_Path" class="Path"() -> ("Value"=w1340:path)  [unwired: 2 in, 2 out]
        n1058 = call "File Dialog4"("start path"=w1340) -> ("selected paths"=w1339:path[], "cancelled"=w1338:bool)  [unwired: 11 in, 2 out]
        n1059 = case shown="False" w1338 {
          tunnel: w1339 -> [w1354 _]
          frame False {
            n1060 = property on="AVS type" class="Enum (strict)"() -> ("Value"=w1344:T35)  [unwired: 2 in, 2 out]
            n1061 = for {
              tunnel: w1354 -> [w1381] mode=indexing
              shift-right: [w1379] -> w1351
              shift-left: string[][] [] ("all rows") -> [w1380]
              # "skip header (7 lines)"
              n1062 = call <vilib>:"Read From Spreadsheet File (string).vi"("file path (dialog if empty)"=w1381) -> ("all rows"=w1377:string[][])  [unwired: 6 in, 4 out]
              n1063 = Array Subset(array=w1377, index (row)=7 ("index")) -> (w1376:string[][])  [unwired: 3 in]
              n1064 = Insert Into Array(array=w1380, new element=w1376) -> (w1379:string[][])  [unwired: 2 in]
            }
            n1065 = case shown="Default" w1344 {
              tunnel: [2 ("index") 2 ("index")] -> w1343
              tunnel: [8 ("length") 10 ("length")] -> w1341
              tunnel: [10 ("index") 12 ("index")] -> w1342
              frame Default {
              }
              frame "Impedance Bridge" {
              }
            }
            n1066 = Index Array(array=w1351, index (col)=1 ("disabled index (col)")) -> (element=w1348:string[])  [unwired: 1 in]
            n1067 = Array Subset(array=w1351, index (col)=w1343, length (col)=w1341) -> (w1350:string[][])  [unwired: 2 in]
            n1068 = Array Subset(array=w1351, index (col)=w1342, length (col)=w1341) -> (w1349:string[][])  [unwired: 2 in]
            n1069 = Transpose 2D Array(2D array=w1350) -> (transposed array=w1346:string[][])
            n1070 = Transpose 2D Array(2D array=w1349) -> (transposed array=w1345:string[][])
            n1071 = for {
              tunnel: w1346 -> [w1373] mode=indexing
              tunnel: w1345 -> [w1372] mode=indexing
              tunnel: w1348 -> [w1374]
              tunnel: [w1371] -> w1347 mode=indexing
              # "Sort data by date and remove duplicate points"
              n1072 = Fract/Exp String To Number(string=w1373) -> (number=w1368:dbl[])  [unwired: 3 in, 1 out]
              n1073 = Fract/Exp String To Number(string=w1374) -> (number=w1370:dbl[])  [unwired: 3 in, 1 out]
              n1074 = Fract/Exp String To Number(string=w1372) -> (number=w1369:dbl[])  [unwired: 3 in, 1 out]
              n1075 = call "Sort 1D Array (DBL)__ogtk.vi"("Array in"=w1370) -> ("Sorted Pointers"=w1375:i32[], "Sorted Array out"=w1363:dbl[])  [unwired: 9 in]
              n1076 = call "Reorder 1D Array2 (DBL)__ogtk.vi"("indices"=w1375, "array"=w1368) -> ("reordered array"=w1367:dbl[])  [unwired: 9 in]
              n1077 = call "Reorder 1D Array2 (DBL)__ogtk.vi"("indices"=w1375, "array"=w1369) -> ("reordered array"=w1365:dbl[])  [unwired: 9 in]
              n1078 = call "Remove Duplicates from 1D Array (DBL)__ogtk.vi"("Input Array"=w1367) -> ("Output Array"=w1366:dbl[], "indices of removed elements"=w1361:i32[])
              n1079 = call "Delete Elements from 1D Array (DBL)__ogtk.vi"("indices"=w1361, "array"=w1365) -> ("array w/ subset deleted"=w1364:dbl[])  [unwired: 8 in, 1 out]
              n1080 = call "Delete Elements from 1D Array (DBL)__ogtk.vi"("indices"=w1361, "array"=w1363) -> ("array w/ subset deleted"=w1362:dbl[])  [unwired: 8 in, 1 out]
              n1081 = Bundle("Output Array"=w1366, "array w/ subset deleted"=w1364, "array w/ subset deleted"=w1362) -> (w1371:T49)  [unwired: 1 in]
            }
            n1082 = local write "Data"(w1347) -> ()
          }
          frame True {
          }
        }
      }
      event "Save Data": Value Change {
        # "Load data from log files"
        n1083 = event-data() -> ()  [unwired: 1 in, 6 out]
        n1084 = property on="AVS_Path" class="Path"() -> ("Value"=w1384:path)  [unwired: 2 in, 2 out]
        n1085 = call "File Dialog"("start path"=w1384) -> ("selected path"=w1382:path, "cancelled"=w1383:bool)  [unwired: 11 in, 2 out]
        n1086 = case shown="False" w1383 {
          tunnel: w1382 -> [w1389 _]
          frame False {
            (unwired) 30 ("dimension size")
            n1087 = local read "Data"() -> (w1390:cluster{"R":dbl[], "T":dbl[], "Time":dbl[]}[])
            n1088 = for {
              tunnel: w1390 -> [w1404] mode=indexing
              tunnel: [w1395] -> w1388 mode=indexing
              shift-right: [w1391] -> w1386
              shift-left: string[][] [] -> [w1392]
              n1089 = Unbundle By Name(w1404) -> ("Time"=w1401:dbl[], "R"=w1400:dbl[], "T"=w1396:dbl[])
              n1090 = property on="Data logging" class="Clust (strict)"() -> ("Value"=w1403:T27)  [unwired: 2 in, 2 out]
              n1091 = Unbundle By Name(w1403) -> ("Date/Time Format"=w1402:string)
              n1092 = Array Size(array=w1396) -> (size(s)=w1395:i32)
              n1093 = for {
                tunnel: w1402 -> [w1407]
                tunnel: [w1406] -> w1399 mode=indexing
                tunnel: w1401 -> [w1405] mode=indexing
                n1094 = Format Date/Time String(time format string (%c)=w1407, seconds (now)=w1405) -> (date/time string=w1406:string)  [unwired: 1 in]
              }
              n1095 = Number To Fractional String(number=w1400) -> (F-format string=w1398:string[])  [unwired: 3 in]
              n1096 = Number To Fractional String(number=w1396) -> (F-format string=w1397:string[])  [unwired: 3 in]
              n1097 = Build Array(w1399, w1398, w1397) -> (w1393:string[][])
              n1098 = Transpose 2D Array(2D array=w1393) -> (transposed array=w1394:string[][])
              n1099 = Build Array (concatenate)(w1392, w1394) -> (w1391:string[][])
            }
            n1100 = Array Max & Min(array=w1388) -> ()  [unwired: 4 out]
            n1101 = call "Write To Spreadsheet File (string) w Error.vi"("transpose? (no:F)"=FALSE, "2D data"=w1386, "file path (dialog if empty)"=w1389) -> ()  [unwired: 7 in, 2 out]
          }
          frame True {
          }
        }
      }
      event "Save Screen Data": Value Change {
        n1102 = event-data() -> ()  [unwired: 1 in, 6 out]
        n1103 = property on="AVS_Path" class="Path"() -> ("Value"=w1410:path)  [unwired: 2 in, 2 out]
        n1104 = call "File Dialog7"("start path"=w1410) -> ("selected path"=w1408:path, "cancelled"=w1409:bool)  [unwired: 11 in, 2 out]
        n1105 = case shown="False" w1409 {
          tunnel: w1408 -> [w1435 _]
          frame False {
            # "!!NOTE:This routine assumes that XY graph is \ncontrol #0 on tab page!!"
            n1106 = property on="Channel Controls" class="TabCtl (strict)"() -> ("Pages"=w1433:refnum<vi>[], "Value"=w1432:T3)  [unwired: 2 in, 2 out]
            n1107 = Index Array(array=w1433, index=w1432) -> (element=w1431:refnum<vi>)
            n1108 = property class="Page"(reference=w1431) -> ("ControlsOnPage"=w1428:refnum<vi>[])  [unwired: 1 in, 2 out]
            n1109 = control-ref of="R-Plot 0"() -> (w1426:refnum<vi>)
            n1110 = Index Array(array=w1428, index=0) -> (element=w1430:refnum<vi>)
            n1111 = Type Cast(type=w1426, x=w1430) -> (*(type *) &x=w1427:refnum<vi>)
            n1112 = property class="XYGraph (strict)"(reference=w1427) -> ("Value"=w1425:cluster{dbl[], dbl[]}, "XScale.Maximum"=w1424:dbl, "XScale.Minimum"=w1423:dbl)  [unwired: 1 in, 2 out]
            n1113 = Unbundle(w1425) -> (w1422:dbl[], w1421:dbl[])
            n1114 = call "MGI Threshold 1D Array Extended.vi"("Threshold Y"=w1424, "Y Value[]"=w1422) -> ("Extended Fractional Index"=w1412:dbl)  [unwired: 1 in]
            n1115 = call "MGI Threshold 1D Array Extended.vi"("Threshold Y"=w1423, "Y Value[]"=w1422) -> ("Extended Fractional Index"=w1411:dbl)  [unwired: 1 in]
            n1116 = Subtract(x=w1412, y=w1411) -> (x-y=w1434:dbl)
            n1117 = Array Subset(array=w1422, index=w1411, length=w1434) -> (w1416:dbl[])
            n1118 = Array Subset(array=w1421, index=w1411, length=w1434) -> (w1414:dbl[])
            n1119 = property on="Data logging" class="Clust (strict)"() -> ("Value"=w1418:T27)  [unwired: 2 in, 2 out]
            n1120 = Unbundle By Name(w1418) -> ("Date/Time Format"=w1417:string)
            n1121 = Number To Fractional String(number=w1414) -> (F-format string=w1413:string[])  [unwired: 3 in]
            n1122 = for {
              tunnel: w1417 -> [w1438]
              tunnel: [w1437] -> w1415 mode=indexing
              tunnel: w1416 -> [w1436] mode=indexing
              n1123 = Format Date/Time String(time format string (%c)=w1438, seconds (now)=w1436) -> (date/time string=w1437:string)  [unwired: 1 in]
            }
            n1124 = Build Array(w1415, w1413) -> (w1420:string[][])
            n1125 = call <vilib>:"Write To Spreadsheet File (string).vi"("transpose? (no:F)"=TRUE, "2D data"=w1420, "file path (dialog if empty)"=w1435) -> ()  [unwired: 5 in, 1 out]
          }
          frame True {
          }
        }
      }
      event "Currents changed": Value Change {
        # "New values for currents were entered by user/automode-> write new data to CS"
        n1126 = event-data() -> ()  [unwired: 1 in, 6 out]
        n1127 = local read "CS ref"() -> (w1443:refnum<class "CS.lvclass">)
        n1128 = property on="CS status" class="Clust (strict)"() -> ("Value"=w1440:errorcluster)  [unwired: 2 in, 2 out]
        n1129 = call-dynamic "Read.vi"("CS in"=w1443, "error in (no error)"=w1440, "Optional"=TRUE ("Unused")) -> ("CS out"=w1442:refnum<class "CS.lvclass">, "error out"=w1439:errorcluster)  [unwired: 11 in, 4 out]
        n1130 = local write "CS ref"(w1442) -> ()
        n1131 = property on="CS status" class="Clust (strict)"("Value"=w1439) -> ()  [unwired: 2 in, 2 out]
      }
      event "I0 output to": Value Change {
        # "Switch QCS channel 0 to aux output"
        n1132 = event-data() -> ("OldVal"=w1450:T29, "NewVal"=w1445:T29)  [unwired: 1 in, 4 out]
        n1133 = To Long Integer(number=w1445) -> (32bit integer=→"Map Channel 0 to 2":i32)
        n1134 = local read "CS ref"() -> (w1448:refnum<class "CS.lvclass">)
        n1135 = property on="CS status" class="Clust (strict)"() -> ("Value"=w1449:errorcluster)  [unwired: 2 in, 2 out]
        n1136 = call-dynamic "Switch Output Channel.vi"("error in (no error)"=w1449, "New Channel"=w1445, "Old Channel"=w1450, "CS in"=w1448) -> ("error out"=w1446:errorcluster, "CS out"=w1447:refnum<class "CS.lvclass">)  [unwired: 6 in]
        n1137 = local write "CS ref"(w1447) -> ()
        n1138 = property on="CS status" class="Clust (strict)"("Value"=w1446) -> ()  [unwired: 2 in, 2 out]
      }
      event "T Sweep.Start": Value Change {
        # "Setup and Start Current/Temperature sweep for CS channel 3"
        n1139 = event-data() -> ("CtlRef"=w1451:refnum<vi>, "NewVal"=w1452:bool)  [unwired: 1 in, 4 out]
        n1140 = case shown="False" w1452 {
          tunnel: w1451 -> [w1453 w1456]
          frame False {
            n1141 = property class="Bool (strict)"(reference=w1453, "Caption.Text"="Start") -> ()  [unwired: 1 in, 2 out]
          }
          frame True {
            n1142 = property on="Start value" class="DigNum (strict)"() -> ("Value"=w1457:dbl)  [unwired: 2 in, 2 out]
            n1143 = property class="Bool (strict)"(reference=w1456, "Caption.Text"="Stop") -> ()  [unwired: 1 in, 2 out]
            n1144 = property on="Current" class="DigNum (strict)"("Val(Sgnl)"=w1457) -> ()  [unwired: 2 in, 2 out]
          }
        }
      }
      event "T Sweep.I_next": Value Change {
        # "Go to next step in Current/Temperature sweep for CS channel 3"
        n1145 = event-data() -> ()  [unwired: 1 in, 6 out]
        n1146 = property on="I_next" class="Bool (strict)"("Value"=FALSE) -> ()  [unwired: 2 in, 2 out]
        n1147 = Get Date/Time In Seconds() -> (seconds since 1Jan1904=w1465:timestamp)
        n1148 = To Double Precision Float(number=w1465) -> (double precision float=w1466:dbl)
        n1149 = local write "Time Old"(w1466) -> ()
        n1150 = property on="Current" class="DigNum (strict)"() -> ("Value"=w1458:dbl)  [unwired: 2 in, 2 out]
        n1151 = property on="Step" class="DigNum (strict)"() -> ("Value"=w1463:dbl)  [unwired: 2 in, 2 out]
        n1152 = Add(x=w1458, y=w1463) -> (x+y=w1462:dbl)
        n1153 = property on="End value" class="DigNum (strict)"() -> ("Value"=w1461:dbl)  [unwired: 2 in, 2 out]
        n1154 = property on="Start value" class="DigNum (strict)"() -> ("Value"=w1460:dbl)  [unwired: 2 in, 2 out]
        n1155 = In Range and Coerce(upper limit=w1461, x=w1462, lower limit=w1460) -> (coerced(x)=w1459:dbl)  [unwired: 1 out]
        n1156 = property on="Current" class="DigNum (strict)"("Val(Sgnl)"=w1459) -> ()  [unwired: 2 in, 2 out]
      }
      event "T Sweep.I_prev": Value Change {
        # "Go to previous step in Current/Temperature sweep for CS channel 3"
        n1157 = event-data() -> ()  [unwired: 1 in, 6 out]
        n1158 = Get Date/Time In Seconds() -> (seconds since 1Jan1904=w1474:timestamp)
        n1159 = property on="I_prev" class="Bool (strict)"("Value"=FALSE) -> ()  [unwired: 2 in, 2 out]
        n1160 = To Double Precision Float(number=w1474) -> (double precision float=w1475:dbl)
        n1161 = local write "Time Old"(w1475) -> ()
        n1162 = property on="Current" class="DigNum (strict)"() -> ("Value"=w1468:dbl)  [unwired: 2 in, 2 out]
        n1163 = property on="Step" class="DigNum (strict)"() -> ("Value"=w1473:dbl)  [unwired: 2 in, 2 out]
        n1164 = Subtract(x=w1468, y=w1473) -> (x-y=w1472:dbl)
        n1165 = property on="End value" class="DigNum (strict)"() -> ("Value"=w1471:dbl)  [unwired: 2 in, 2 out]
        n1166 = property on="Start value" class="DigNum (strict)"() -> ("Value"=w1470:dbl)  [unwired: 2 in, 2 out]
        n1167 = In Range and Coerce(upper limit=w1471, x=w1472, lower limit=w1470) -> (coerced(x)=w1469:dbl)  [unwired: 1 out]
        n1168 = property on="Current" class="DigNum (strict)"("Val(Sgnl)"=w1469) -> ()  [unwired: 2 in, 2 out]
      }
      event "Reset PID", "PID setup 2.Integral Gain": Value Change {
        # "Reset the PID loop"
        n1169 = event-data() -> ()  [unwired: 1 in, 6 out]
        n1170 = property on="ResetPIDloop" class="TypRef (strict)"() -> ("Value"=w1477:refnum<user-event>)  [unwired: 2 in, 2 out]
        n1171 = Generate User Event(user event=w1477, event data cluster="" ("event data")) -> ()  [unwired: 2 in, 2 out]
      }
      event User Event {
        # "Reset the PID loop"
        n1172 = event-data() -> ()  [unwired: 1 in, 5 out]
        n1173 = local write "Error"(0.0 ("T_error")) -> ()
      }
      event "Minimize", "Minimize 2": Value Change {
        (unwired) 29 ("Splitter Position")
        (unwired) 534 ("Numeric 2")
        # "Shrink/restore the program window"
        # "726"
        # "222"
        # "1243"
        # "816"
        n1174 = event-data() -> ()  [unwired: 1 in, 6 out]
        n1175 = case shown="True" "Minimize" {
          tunnel: "Minimize 2" -> [_ w1506]
          frame True {
            (unwired) T35."Disabled" ("Value")
            n1176 = property on="CS type" class="Enum (strict)"() -> ("Value"=w1491:T36)  [unwired: 2 in, 2 out]
            n1177 = property on="AVS type" class="Enum (strict)"() -> ("Value"=w1486:T35)  [unwired: 2 in, 2 out]
            n1178 = Equal?(x=w1486, y=T35."Disabled" ("Value")) -> (x = y?=w1484:bool)
            n1179 = Equal?(x=w1491, y=T36."Disabled" ("Value")) -> (x = y?=w1490:bool)
            n1180 = property on="Data History" class="TabCtl (strict)"("Value"=enum32{"History", "Settings"}."History" ("Data History")) -> ()  [unwired: 2 in, 2 out]
            n1181 = Exclusive Or(1:w1484, 2:w1490) -> (0:w1483:bool)
            n1182 = property on="Mode Buttons" class="RadioBtnsControl (strict)"("Disabled"=u8 2, "Val(Sgnl)"=T13."No Selection" ("Value (Signaling)")) -> ()  [unwired: 2 in, 2 out]
            n1183 = property class="VI"() -> ("Front Panel.PanelBounds"=w1494:T50)  [unwired: 2 in, 2 out]
            n1184 = Select(t=i16 105 ("y"), s=w1483, f=i16 169 ("y")) -> (s? t:f=w1487:i16)
            n1185 = Unbundle By Name(w1494) -> ("Left"=w1500:i16, "Top"=w1497:i16)
            n1186 = property on="Splitter 3" class="Splitter"("Position"=29 ("Splitter Position")) -> (error out=w1485:errorcluster)  [unwired: 2 in, 1 out]
            n1187 = Add(x=i16 806 ("right"), y=w1500) -> (x+y=w1499:i16)
            n1188 = Add(x=w1497, y=w1487) -> (x+y=w1496:i16)
            n1189 = Bundle By Name(cluster=w1494, "Right"=w1499, "Bottom"=w1496) -> (w1501:T50)
            n1190 = case shown="False" w1484 {
              tunnel: w1485 -> [_ w1504]
              frame False {
              }
              frame True {
                n1191 = property on="Splitter 4" class="Splitter"(error in=w1504, "Position"=32 ("Splitter Position")) -> ()  [unwired: 1 in, 2 out]
              }
            }
            n1192 = property class="VI"("Front Panel.PanelBounds"=w1501) -> ()  [unwired: 2 in, 2 out]
          }
          frame False {
            n1193 = property class="VI"() -> ("Front Panel.PanelBounds"=w1513:T50)  [unwired: 2 in, 2 out]
            n1194 = property on="Channel Controls" class="TabCtl (strict)"() -> ("Value"=w1521:T3)  [unwired: 2 in, 2 out]
            n1195 = Unbundle By Name(w1513) -> ("Left"=w1519:i16, "Top"=w1517:i16)
            n1196 = property on="Channel Controls" class="TabCtl (strict)"("Val(Sgnl)"=w1521) -> ()  [unwired: 2 in, 2 out]
            n1197 = Select(t=i16 806 ("right"), s=w1506, f=i16 1233 ("right")) -> (s? t:f=w1510:i16)
            n1198 = Add(x=w1510, y=w1519) -> (x+y=w1518:i16)
            n1199 = Add(x=w1517, y=i16 704) -> (x+y=w1515:i16)
            n1200 = Bundle By Name(cluster=w1513, "Right"=w1518, "Bottom"=w1515) -> (w1520:T50)
            n1201 = property on="Mode Buttons" class="RadioBtnsControl (strict)"("Disabled"=u8 0) -> ()  [unwired: 2 in, 2 out]
            n1202 = property class="VI"("Front Panel.PanelBounds"=w1520) -> (error out=w1507:errorcluster)  [unwired: 2 in, 1 out]
            n1203 = property on="Splitter 3" class="Splitter"(error in=w1507, "Position"=559 ("Splitter Position")) -> (error out=w1511:errorcluster)  [unwired: 1 in, 1 out]
            n1204 = property on="Splitter 4" class="Splitter"(error in=w1511, "Position"=635 ("Splitter Position")) -> ()  [unwired: 1 in, 2 out]
          }
        }
        n1205 = property on="Splitter 2" class="Splitter"("Position"=805 ("Splitter Position")) -> ()  [unwired: 2 in, 2 out]
      }
      event "Copy to Clipboard": Value Change {
        # "Copy current values to the clipboard"
        n1206 = event-data() -> ()  [unwired: 1 in, 6 out]
        n1207 = property on="Data array" class="Arr (strict)"() -> ("Value"=w1526:dbl[])  [unwired: 2 in, 2 out]
        n1208 = property on="T_array" class="Arr (strict)"() -> ("Value"=w1525:dbl[])  [unwired: 2 in, 2 out]
        n1209 = Build Array(w1526, w1525) -> (w1524:dbl[][])
        n1210 = Transpose 2D Array(2D array=w1524) -> (transposed array=w1523:dbl[][])
        n1211 = Array To Spreadsheet String(delimiter (Tab)="\t", array=w1523, 3:"%.4g" ("format string")) -> (spreadsheet string=w1529:string)
        n1212 = invoke class="App" method="Clipboard.Write"("Param 0"=w1529) -> ()  [unwired: 3 in, 4 out]
      }
      event "Show PID graph?": Value Change {
        # "Display plots with the PID parameters vs time for debugging"
        n1213 = event-data() -> ("NewVal"=w1530:bool)  [unwired: 1 in, 5 out]
        n1214 = property on="Channel Controls" class="TabCtl (strict)"() -> ("Pages"=w1533:refnum<vi>[])  [unwired: 2 in, 2 out]
        n1215 = Reverse 1D Array(array=w1533) -> (reversed array=w1532:refnum<vi>[])
        n1216 = Index Array(array=w1532) -> (element=w1531:refnum<vi>)  [unwired: 1 in]
        n1217 = property class="Page"(reference=w1531, "PageVis"=w1530) -> ()  [unwired: 1 in, 2 out]
      }
      event "I0.uA", "I1.uA", "I2.uA", "I3.uA": Mouse Up {
        # "Show curent edit filed on double clicking the current indicator. Set the field to the actual current value."
        n1218 = event-data() -> ("Mods.Double Click"=w1535:bool, "CtlRef"=w1534:refnum<vi>)  [unwired: 1 in, 5 out]
        n1219 = case shown="True" w1535 {
          tunnel: w1534 -> [_ w1546]
          frame False {
          }
          frame True {
            w1542 = TRUE ("Visible")
            n1220 = property class="Str"(reference=w1546) -> ("Owner"=w1545:refnum<vi>)  [unwired: 1 in, 2 out]
            n1221 = control-ref of="uA 0"() -> (w1552:refnum<vi>)
            n1222 = control-ref of="uA 1"() -> (w1555:refnum<vi>)
            n1223 = control-ref of="uA 2"() -> (w1554:refnum<vi>)
            n1224 = control-ref of="uA 3"() -> (w1553:refnum<vi>)
            n1225 = control-ref of="I0"() -> (w1543:refnum<vi>)
            n1226 = control-ref of="I1"() -> (w1549:refnum<vi>)
            n1227 = control-ref of="I2"() -> (w1548:refnum<vi>)
            n1228 = control-ref of="I3"() -> (w1541:refnum<vi>)
            n1229 = property on="I" class="Arr (strict)"() -> ("Value"=w1540:dbl[])  [unwired: 2 in, 2 out]
            n1230 = Type Cast(type=w1541, x=w1545) -> (*(type *) &x=w1544:refnum<vi>)
            n1231 = Build Array(w1552, w1555, w1554, w1553) -> (w1551:refnum<vi>[])
            n1232 = Build Array(w1543, w1549, w1548, w1541) -> (w1547:refnum<vi>[])
            n1233 = Search 1D Array(1D array=w1547, element=w1544) -> (index of element=w1539:i32)  [unwired: 1 in]
            n1234 = Index Array(array=w1540, index=w1539) -> (element=w1538:dbl)
            n1235 = Index Array(array=w1551, index=w1539) -> (element=w1550:refnum<vi>)
            n1236 = Multiply(x=1000.0, y=w1538) -> (x*y=w1537:dbl)
            n1237 = property on="Property Node" class="DigNum (strict)"(reference=w1550, "Value"=w1537, "Visible"=w1542, "Key Focus"=w1542) -> ()  [unwired: 1 in, 2 out]
          }
        }
      }
      event "I0.current flows", "I1.current flows", "I2.current flows", "I3.current flows": Mouse Up {
        # "Toggle the current channel by double clickin on the \"On\" led in the current indicator."
        n1238 = event-data() -> ("CtlRef"=w1556:refnum<vi>, "Mods.Double Click"=w1557:bool)  [unwired: 1 in, 5 out]
        n1239 = case shown="True" w1557 {
          tunnel: w1556 -> [_ w1566]
          frame False {
          }
          frame True {
            n1240 = control-ref of="current flows"() -> (w1571:refnum<vi>)
            n1241 = control-ref of="current flows"() -> (w1570:refnum<vi>)
            n1242 = control-ref of="current flows"() -> (w1569:refnum<vi>)
            n1243 = control-ref of="current flows"() -> (w1568:refnum<vi>)
            n1244 = control-ref of="Toggle ON/OFF"() -> (w1565:refnum<vi>)
            n1245 = control-ref of="Toggle ON/OFF"() -> (w1563:refnum<vi>)
            n1246 = control-ref of="Toggle ON/OFF"() -> (w1562:refnum<vi>)
            n1247 = control-ref of="Toggle ON/OFF"() -> (w1564:refnum<vi>)
            n1248 = Build Array(w1571, w1570, w1569, w1568) -> (w1567:refnum<vi>[])
            n1249 = Build Array(w1565, w1563, w1562, w1564) -> (w1561:refnum<vi>[])
            n1250 = Search 1D Array(1D array=w1567, element=w1566) -> (index of element=w1560:i32)  [unwired: 1 in]
            n1251 = Index Array(array=w1561, index=w1560) -> (element=w1559:refnum<vi>)
            n1252 = property class="Bool (strict)"(reference=w1559, "Val(Sgnl)"=TRUE ("Value (Signaling)")) -> ()  [unwired: 1 in, 2 out]
          }
        }
      }
      event "uA 0", "uA 1", "uA 2", "uA 3": Value Change {
        w1573 = refnum<vi> refnum  # Numeric
        w1577 = refnum<vi> refnum  # Enum
        # "User has entered the current by double clicking on the current indicators at the bottom. \nSet range to \"Auto\" and interpret the entered value as [uA]"
        # "!!NOTE:This routine assumes that Current and Range are controls #2 & #3 in current control cluster"
        n1253 = event-data() -> ("CtlRef"=w1585:refnum<vi>, "NewVal"=w1572:u32)  [unwired: 1 in, 4 out]
        n1254 = control-ref of="C_I0"() -> (w1594:refnum<vi>)
        n1255 = control-ref of="C_I1"() -> (w1592:refnum<vi>)
        n1256 = control-ref of="C_I2"() -> (w1593:refnum<vi>)
        n1257 = control-ref of="C_I3"() -> (w1595:refnum<vi>)
        n1258 = control-ref of="uA 0"() -> (w1587:refnum<vi>)
        n1259 = control-ref of="uA 1"() -> (w1590:refnum<vi>)
        n1260 = control-ref of="uA 2"() -> (w1589:refnum<vi>)
        n1261 = control-ref of="uA 3"() -> (w1588:refnum<vi>)
        n1262 = Build Array(w1594, w1592, w1593, w1595) -> (w1591:refnum<vi>[])
        n1263 = Build Array(w1587, w1590, w1589, w1588) -> (w1586:refnum<vi>[])
        n1264 = Search 1D Array(1D array=w1586, element=w1585) -> (index of element=w1584:i32)  [unwired: 1 in]
        n1265 = Index Array(array=w1591, index=w1584) -> (element=w1583:refnum<vi>)
        n1266 = property class="Clust (strict)"(reference=w1583) -> ("Controls[]"=w1582:refnum<vi>[])  [unwired: 1 in, 2 out]
        n1267 = Index Array(array=w1582, index #1=3 ("index"), index #2=2 ("index")) -> (element #1=w1579:refnum<vi>, element #2=w1575:refnum<vi>)
        n1268 = Type Cast(type=w1573, x=w1575) -> (*(type *) &x=w1574:refnum<vi>)
        n1269 = Type Cast(type=w1577, x=w1579) -> (*(type *) &x=w1578:refnum<vi>)
        n1270 = property on="Property Node" class="Num"(reference=w1574, "Value"=w1572) -> ()  [unwired: 1 in, 2 out]
        n1271 = property on="Property Node" class="Enum"(reference=w1578, "Value"=T37."Auto") -> ()  [unwired: 1 in, 2 out]
      }
      event "Ranges": Value Change {
        # "If user has changed the exitation, update the AVS bridge settings."
        n1272 = event-data() -> ("NewVal"=w1597:T18)  [unwired: 1 in, 5 out]
        n1273 = property on="Exc&Ranges" class="Clust (strict)"() -> ("Value"=w1596:T9)  [unwired: 2 in, 2 out]
        n1274 = call "Combine Excitation&Range.vi"("Ranges"=w1597, "Exc&Ranges In"=w1596) -> ("Exc&Ranges Out"=w1598:T51)
        n1275 = property on="Exc&Ranges" class="Clust (strict)"("Value"=w1598) -> ()  [unwired: 2 in, 2 out]
      }
      event Panel Close? {
        # "Ask for confirmation is user is trying to close the program"
        n1276 = event-data() -> ()  [unwired: 1 in, 4 out]
        n1277 = Two Button Dialog(message="Are you sure you want to quit the program?") -> (T button?=w1600:bool)  [unwired: 2 in]
        n1278 = Not(x=w1600) -> (.not. x?=w1601:bool)
        n1279 = event-data("Discard?"=w1601) -> ()  [unwired: 1 in, 1 out]
      }
      event "Save config": Mouse Up {
        (unwired) T39."HKEY_CURRENT_USER" ("root key (HKEY_LOCAL_MACHINE) 2")
        # "Save parameters to the configuration file"
        n1280 = event-data() -> ()  [unwired: 1 in, 8 out]
        n1281 = control-ref of="CS Names"() -> (w1612:refnum<vi>)
        n1282 = control-ref of="AVS names"() -> (w1611:refnum<vi>)
        n1283 = control-ref of="CurCalibrations"() -> (w1605:refnum<vi>)
        n1284 = control-ref of="I3 as temp"() -> (w1603:refnum<vi>)
        n1285 = control-ref of="Automode Settings 2"() -> (w1602:refnum<vi>)
        n1286 = control-ref of="Active"() -> (w1604:refnum<vi>)
        n1287 = control-ref of="Bridge settings"() -> (w1618:refnum<vi>)
        n1288 = control-ref of="AVS Runtime Settings"() -> (w1619:refnum<vi>)
        n1289 = control-ref of="Current source settings"() -> (w1617:refnum<vi>)
        n1290 = control-ref of="Thermometer"() -> (w1620:refnum<vi>)
        n1291 = control-ref of="PID setup 2"() -> (w1621:refnum<vi>)
        n1292 = control-ref of="Data logging"() -> (w1616:refnum<vi>)
        n1293 = call "Current VIs Parent Directory__ogtk.vi"() -> ("Parent Directory (+ Relative)"=w1608:path)  [unwired: 5 in]
        n1294 = call "File Dialog3"("start path"=w1608, "pattern (all files)"="*.ini") -> ("selected path"=w1606:path)  [unwired: 10 in, 3 out]
        n1295 = Build Array(w1604, w1618, w1619, w1617, w1616, w1620, w1621, w1612, w1611, w1605, w1603, w1602) -> (w1614:refnum<vi>[])
        n1296 = call "Save Load Settings to File by Ref with path.vi"("Array of Cluster References"=w1614, "subkey"="SOFTWARE\\Leiden Cryogenics\\TC" ("subkey 2"), "Action"=enum8{"Load", "Save"}."Save", "error in (no error)"=w1610, "configuration file path"=w1606) -> ("error out"=w1609:errorcluster)  [unwired: 4 in]
      }
      event "Load config": Mouse Up {
        # "Load parameters from the configuration file"
        n1297 = event-data() -> ()  [unwired: 1 in, 8 out]
        n1298 = flat-sequence {
          tunnel: [w1646] -> w1631
          tunnel: w1627 -> [w1641]
          tunnel: [w1636] -> w1622
          tunnel: w1631 -> [w1662]
          tunnel: [w1662] -> w1630
          tunnel: [w1660] -> w1623
          tunnel: w1622 -> [w1660]
          tunnel: [w1667] -> w1629
          tunnel: w1630 -> [w1666]
          tunnel: [w1664] -> w1624
          tunnel: w1623 -> [w1664]
          tunnel: w1629 -> [w1673]
          tunnel: [w1673] -> w1628
          tunnel: [w1671] -> w1625
          tunnel: w1624 -> [w1671]
          tunnel: w1628 -> [w1676]
          tunnel: [w1675] -> w1626
          tunnel: w1625 -> [w1674]
          frame #0 {
            (unwired) T39."HKEY_CURRENT_USER" ("root key (HKEY_LOCAL_MACHINE) 2")
            n1299 = call "Current VIs Parent Directory__ogtk.vi"() -> ("Parent Directory (+ Relative)"=w1638:path)  [unwired: 5 in]
            n1300 = control-ref of="Active"() -> (w1634:refnum<vi>)
            n1301 = control-ref of="Bridge settings"() -> (w1647:refnum<vi>)
            n1302 = control-ref of="AVS Runtime Settings"() -> (w1643:refnum<vi>)
            n1303 = control-ref of="Current source settings"() -> (w1644:refnum<vi>)
            n1304 = control-ref of="Data logging"() -> (w1645:refnum<vi>)
            n1305 = control-ref of="PID setup 2"() -> (w1642:refnum<vi>)
            n1306 = control-ref of="CS Names"() -> (w1640:refnum<vi>)
            n1307 = control-ref of="AVS names"() -> (w1639:refnum<vi>)
            n1308 = control-ref of="CurCalibrations"() -> (w1635:refnum<vi>)
            n1309 = control-ref of="I3 as temp"() -> (w1633:refnum<vi>)
            n1310 = control-ref of="Automode Settings 2"() -> (w1632:refnum<vi>)
            n1311 = call "File Dialog2"("start path"=w1638, "pattern (all files)"="*.ini") -> ("selected path"=w1636:path)  [unwired: 10 in, 3 out]
            n1312 = Build Array(w1634, w1647, w1643, w1644, w1645, w1642, w1640, w1639, w1635, w1633, w1632) -> (w1649:refnum<vi>[])
            n1313 = call "Save Load Settings to File by Ref with path.vi"("Array of Cluster References"=w1649, "subkey"="SOFTWARE\\Leiden Cryogenics\\TC" ("subkey 2"), "Action"=enum8{"Load", "Save"}."Load", "error in (no error)"=w1641, "configuration file path"=w1636) -> ("error out"=w1651:errorcluster)  [unwired: 4 in]
            n1314 = disable-structure shown="Disabled" {
              disable-tunnel: w1651 -> [w1654 w1659]
              disable-tunnel: [w1652 w1659] -> w1646
              frame Disabled {
                n1315 = property on="AVS type" class="Enum (strict)"(error in=w1654) -> (error out=w1655:errorcluster, "Value"=w1657:T35)  [unwired: 1 in, 1 out]
                n1316 = Equal To 0?(x=w1657) -> (x = 0?=w1658:bool)
                n1317 = property on="Address" class="VISAName"(error in=w1655, "Visible"=w1658) -> (error out=w1656:errorcluster)  [unwired: 1 in, 1 out]
                n1318 = Not(x=w1658) -> (.not. x?=w1653:bool)
                n1319 = property on="AVS_SPort" class="VISAName"(error in=w1656, "Visible"=w1653) -> (error out=w1652:errorcluster)  [unwired: 1 in, 1 out]
              }
              frame Enabled {
              }
            }
          }
          frame #1 {
            n1320 = Wait (ms)(milliseconds to wait=250) -> ()  [unwired: 1 out]
          }
          frame #2 {
            n1321 = control-ref of="Thermometer"() -> (w1665:refnum<vi>)
            n1322 = control-ref of="CurCalibrations"() -> (w1663:refnum<vi>)
            n1323 = control-ref of="AVS_CalFolder"() -> (w1669:refnum<vi>)
            n1324 = control-ref of="Select sensor 1"() -> (w1670:refnum<vi>)
            n1325 = control-ref of="Select sensor 1"() -> (w1668:refnum<vi>)
            n1326 = call "ReloadCalibrations.vi"("error in (no error)"=w1666, "Quick convert sensors"=w1668, "CurCalibrations"=w1663, "Calibration files path"=w1669, "Channel1 sensors"=w1670, "Channels list"=w1665) -> ("error out"=w1667:errorcluster)  [unwired: 1 in]
          }
          frame #3 {
            n1327 = Wait (ms)(milliseconds to wait=250) -> ()  [unwired: 1 out]
          }
          frame #4 {
            n1328 = disable-structure shown="Enabled" {
              disable-tunnel: w1676 -> [w1679 w1687]
              disable-tunnel: [w1678 w1685] -> w1675
              disable-tunnel: w1674 -> [w1677 _]
              frame Enabled {
                (unwired) T39."HKEY_CURRENT_USER" ("root key (HKEY_LOCAL_MACHINE) 2")
                n1329 = control-ref of="Thermometer"() -> (w1682:refnum<vi>)
                n1330 = Build Array(w1682) -> (w1681:refnum<vi>[])
                n1331 = call "Save Load Settings to File by Ref with path.vi"("Array of Cluster References"=w1681, "subkey"="SOFTWARE\\Leiden Cryogenics\\TC" ("subkey 2"), "Action"=enum8{"Load", "Save"}."Load", "error in (no error)"=w1679, "configuration file path"=w1677) -> ("error out"=w1678:errorcluster)  [unwired: 4 in]
              }
              frame Disabled {
                n1332 = property on="UpdateCalibrations" class="TypRef (strict)"(error in=w1687) -> (error out=w1686:errorcluster, "Value"=w1688:refnum<user-event>)  [unwired: 1 in, 1 out]
                n1333 = Generate User Event(user event=w1688, event data cluster="" ("event data"), error in=w1686) -> (error out=w1685:errorcluster)  [unwired: 1 in, 1 out]
              }
            }
          }
        }
      }
      event "Save Screen Data 2": Value Change {
        # "Show parameters menu. (only for zBridge)"
        n1334 = event-data() -> ()  [unwired: 1 in, 6 out]
        n1335 = disable-structure shown="Enabled" {
          frame Enabled {
            w1693 = 0 ("Page")
            n1336 = local read "zConfig"() -> (w1689:path)
            n1337 = local read "zDll"() -> (w1690:path)
            n1338 = call "SetParFilePath.vi"("path"=w1689, "zDll"=w1690) -> ("error out"=w1691:errorcluster, "zDll out"=w1692:path)  [unwired: 8 in]
            n1339 = call "ParamMenu.vi"("error in (no error)"=w1691, "Subpage"=w1693, "Page"=w1693, "path in"=w1692) -> ()  [unwired: 6 in, 2 out]
          }
          frame Disabled {
            n1340 = local read "zConfig"() -> (w1696:path)
            n1341 = local read "zDll"() -> (w1694:path)
            n1342 = call "SetParFilePath.vi"("path"=w1696, "zDll"=w1694) -> ("zDll out"=w1695:path)  [unwired: 8 in, 1 out]
            n1343 = call "zBridgeSettings_1page.vi"("zDll"=w1695) -> ()  [unwired: 10 in, 1 out]
          }
        }
      }
      event "Edit Calibrations": Value Change {
        # "Show calibration files editor. Works with .cal and .cal2 files only"
        n1344 = event-data() -> ("NewVal"=w1705:T6)  [unwired: 1 in, 5 out]
        n1345 = Cluster To Array(cluster=w1705) -> (array=w1704:bool[])
        n1346 = local read "CurCalibrations"() -> (w1699:T23)
        n1347 = Search 1D Array(1D array=w1704, element=TRUE) -> (index of element=w1702:i32)  [unwired: 1 in]
        n1348 = Cluster To Array(cluster=w1699) -> (array=w1698:string[])
        n1349 = Index Array(array=w1698, index=w1702) -> (element=w1701:string)
        n1350 = property on="AVS_CalFolder" class="Path"() -> ("Value"=w1700:path)  [unwired: 2 in, 2 out]
        n1351 = call "Edit Calibration Coefficients.vi"("Calibration Name"=w1701, "Calibration folder"=w1700) -> ("Cancelled?"=w1697:bool)  [unwired: 1 out]
        n1352 = case shown="False" w1697 {
          frame False {
            n1353 = property on="UpdateCalibrations" class="TypRef (strict)"() -> ("Value"=w1707:refnum<user-event>)  [unwired: 2 in, 2 out]
            n1354 = Generate User Event(user event=w1707, event data cluster="" ("event data")) -> ()  [unwired: 2 in, 2 out]
          }
          frame True {
          }
        }
      }
      event "Edit calibration": Value Change {
        # "Show calibration files editor for quick convert R->T. Works with .cal and .cal2 files only"
        n1355 = event-data() -> ()  [unwired: 1 in, 6 out]
        n1356 = property on="Select sensor 1" class="Ring (strict)"() -> ("Strings []"=w1710:string[], "Value"=w1711:u16)  [unwired: 2 in, 2 out]
        n1357 = Index Array(array=w1710, index=w1711) -> (element=w1709:string)
        n1358 = property on="AVS_CalFolder" class="Path"() -> ("Value"=w1712:path)  [unwired: 2 in, 2 out]
        n1359 = call "Edit Calibration Coefficients.vi"("Calibration Name"=w1709, "Calibration folder"=w1712) -> ("Cancelled?"=w1708:bool)  [unwired: 1 out]
        n1360 = case shown="False" w1708 {
          frame False {
            n1361 = property on="UpdateCalibrations" class="TypRef (strict)"() -> ("Value"=w1714:refnum<user-event>)  [unwired: 2 in, 2 out]
            n1362 = Generate User Event(user event=w1714, event data cluster="" ("event data")) -> ()  [unwired: 2 in, 2 out]
          }
          frame True {
          }
        }
      }
      event "zBridge params.AVS Name 0", "zBridge params.AVS Name 1", "zBridge params.AVS Name 2", "zBridge params.AVS Name 3", "zBridge params.AVS Name 4", "zBridge params.AVS Name 5", "zBridge params.AVS Name 6", "zBridge params.AVS Name 7", "zBridge params.AVS Name 8", "zBridge params.AVS Name 9": Mouse Down {
        # "Show parameters menu for the channel by double clicking on \"Channel parameters\". (only for zBridge)"
        n1363 = event-data() -> ("CtlRef"=w1717:refnum<vi>, "Mods.Double Click"=w1716:bool, "PlatMods.Alt"=w1715:bool)  [unwired: 1 in, 5 out]
        n1364 = case shown="False" w1716 {
          tunnel: w1717 -> [w1720 w1725]
          tunnel: w1715 -> [_ w1724]
          frame True {
            n1365 = control-ref of="zBridge params"() -> (w1722:refnum<vi>)
            n1366 = property class="Clust (strict)"(reference=w1722) -> ("Controls[]"=w1721:refnum<vi>[])  [unwired: 1 in, 2 out]
            n1367 = Search 1D Array(1D array=w1721, element=w1720) -> (index of element=w1718:i32)  [unwired: 1 in]
            n1368 = local read "zDll"() -> (w1723:path)
            n1369 = call "ParamMenu.vi"("Subpage"=w1718, "Page"=0, "path in"=w1723) -> ()  [unwired: 7 in, 2 out]
          }
          frame False {
            n1370 = case shown="True" w1724 {
              tunnel: w1725 -> [_ w1728]
              frame False {
              }
              frame True {
                # "Show information window.\nTends to crash the acquisition!"
                n1371 = control-ref of="zBridge params"() -> (w1730:refnum<vi>)
                n1372 = property class="Clust (strict)"(reference=w1730) -> ("Controls[]"=w1729:refnum<vi>[])  [unwired: 1 in, 2 out]
                n1373 = local read "zDll"() -> (w1727:path)
                n1374 = Search 1D Array(1D array=w1729, element=w1728) -> (index of element=w1726:i32)  [unwired: 1 in]
                n1375 = call "Show Info Window.vi"("Data set number"=w1726, "zDll"=w1727) -> ()  [unwired: 8 in, 2 out]
              }
            }
          }
        }
      }
      event "Active.active Channel 0", "Active.active Channel 1", "Active.active Channel 2", "Active.active Channel 3", "Active.active Channel 4", "Active.active Channel 5", "Active.active Channel 6", "Active.active Channel 7", "Active.active Channel 8", "Active.active Channel 9": Mouse Down {
        # "Switch channels On/Off by double clicking on \"Active\" LED. (only for zBridge and AVS47B)"
        n1376 = event-data() -> ("CtlRef"=w1733:refnum<vi>, "Mods.Double Click"=w1731:bool)  [unwired: 1 in, 6 out]
        n1377 = property on="AVS type" class="Enum (strict)"() -> ("Value"=w1732:T35)  [unwired: 2 in, 2 out]
        n1378 = case shown="True" w1731 {
          tunnel: w1733 -> [_ w1735]
          tunnel: w1732 -> [_ w1739]
          frame False {
          }
          frame True {
            n1379 = control-ref of="Active"() -> (w1738:refnum<vi>)
            n1380 = property class="Clust (strict)"(reference=w1738) -> ("Controls[]"=w1736:refnum<vi>[])  [unwired: 1 in, 2 out]
            n1381 = property class="Bool (strict)"(reference=w1735) -> ("Value"=w1734:bool)  [unwired: 1 in, 2 out]
            n1382 = Search 1D Array(1D array=w1736, element=w1735) -> (index of element=w1737:i32)  [unwired: 1 in]
            n1383 = case shown="Default" w1739 {
              tunnel: w1737 -> [_ w1744 w1745]
              tunnel: w1736 -> [_ w1743 _]
              tunnel: w1734 -> [_ w1740 _]
              frame Default {
              }
              frame "AVS47B (RS232 interface)" {
                n1384 = Index Array(array=w1743, index=w1744) -> (element=w1742:refnum<vi>)
                n1385 = Not(x=w1740) -> (.not. x?=w1741:bool)
                n1386 = property class="Ctl"(reference=w1742, "Value"=w1741) -> ()  [unwired: 1 in, 2 out]
              }
              frame "Impedance Bridge" {
                w1747 = T52."Active" ("Enum")
                # "Invert Active flag"
                n1387 = local read "zDll"() -> (w1750:path)
                n1388 = call "GetByteParam.vi"("ParNo"=w1747, "SetNo"=w1745, "zDll"=w1750) -> ("return type"=w1749:u8)  [unwired: 6 in, 2 out]
                n1389 = Decrement(x=w1749) -> (x-1=w1748:i8)
                n1390 = Absolute Value(x=w1748) -> (abs(x)=w1746:i8)
                n1391 = call "SetByteParam.vi"("SetNo"=w1745, "ParNo"=w1747, "Data"=w1746, "zDll"=w1750) -> ()  [unwired: 6 in, 2 out]
              }
            }
          }
        }
      }
      event "Small R.R1 2", "Small R.R1 2", "Small R.R1 2", "Small R.R1 2", "Small R.R1 2", "Small R.R1 2", "Small R.R1 2", "Small R.R1 2", "Small R.R1 2", "Small R.R1 2", "Small T.R1", "Small T.R1", "Small T.R1", "Small T.R1", "Small T.R1", "Small T.R1", "Small T.R1", "Small T.R1", "Small T.R1", "Small T.R1": Mouse Down {
        n1392 = event-data() -> ()  [unwired: 1 in, 8 out]
      }
      event "PID setup 2.FB on 2": Value Change {
        n1393 = event-data() -> ("NewVal"=w1753:enum16{"0", "1", "2", "3"})  [unwired: 1 in, 5 out]
        n1394 = property on="ResetPIDloop" class="TypRef (strict)"() -> ("Value"=w1762:refnum<user-event>)  [unwired: 2 in, 2 out]
        n1395 = Generate User Event(user event=w1762, event data cluster="" ("event data")) -> ()  [unwired: 2 in, 2 out]
        n1396 = property on="I3 as temp 2" class="Bool (strict)"() -> ("Value"=w1755:bool)  [unwired: 2 in, 2 out]
        n1397 = Initialize Array(FALSE, 4 ("dimension size")) -> (w1757:bool[])
        n1398 = And(x=TRUE ("new element/subarray"), y=w1755) -> (x .and. y?=w1754:bool)
        n1399 = Replace Array Subset(array=w1757, new element=w1754, index=w1753) -> (→"T Channel":bool[])
        n1400 = Index Array(array=string[] ["%#_g uA", "%#_g mK"], index=w1753) -> ()  [unwired: 1 out]
      }
      event "AVS names": Value Change {
        # "Update channel names on the small bottom panel when the names are changed."
        n1401 = event-data() -> ("NewVal"=→"AVS names small":T5)  [unwired: 1 in, 5 out]
      }
      event "I_list": Value Change {
        n1402 = event-data() -> ("NewVal"=w1767:dbl[][])  [unwired: 1 in, 5 out]
        n1403 = local read "I_list_idx"() -> (w1766:i32)
        n1404 = Decrement(x=w1766) -> (x-1=w1765:i32)
        n1405 = Array Size(array=w1767) -> (size(s)=w1769:i32[])
        n1406 = Index Array(array=w1769) -> (element=→"I_list_idx_max":i32)  [unwired: 1 in]
        n1407 = Index Array(array=w1767, index (row)=w1765) -> (element=→"I_list[i]":dbl[])  [unwired: 1 in]
      }
      event "I_list": Shortcut Menu Activation? {
        n1408 = event-data() -> ()  [unwired: 1 in, 7 out]
        n1409 = event-data() -> ()  [unwired: 2 in, 1 out]
      }
      event "I_list": Shortcut Menu Selection (App) {
        n1410 = event-data() -> ("ItemTag"=w1770:string)  [unwired: 1 in, 7 out]
        n1411 = case shown="\"APP_SC_COPY_DATA\"" w1770 {
          frame Default {
          }
          frame "APP_SC_PASTE_DATA" {
            n1412 = invoke class="App" method="Clipboard.Read"() -> ("Read Clipbrd"=w1773:string)  [unwired: 3 in, 2 out]
            n1413 = Spreadsheet String To Array(format string="%d", spreadsheet string=w1773) -> (array=w1771:dbl[][])  [unwired: 2 in]
            n1414 = local write "I_list"(w1771) -> ()
          }
          frame "APP_SC_COPY_DATA" {
            n1415 = local read "I_list"() -> (w1776:dbl[][])
            n1416 = Array To Spreadsheet String(array=w1776, 3:"%d" ("format string")) -> (spreadsheet string=w1774:string)  [unwired: 1 in]
            n1417 = invoke class="App" method="Clipboard.Write"("Param 0"=w1774) -> ()  [unwired: 3 in, 4 out]
          }
        }
      }
      event "I_tofirst": Value Change {
        n1418 = event-data() -> ("OldVal"=w1777:bool)  [unwired: 1 in, 5 out]
        n1419 = local write "I_tofirst"(w1777) -> ()
        n1420 = property on="I_list_idx" class="DigNum (strict)"("Val(Sgnl)"=1 ("Value (Signaling)")) -> ()  [unwired: 2 in, 2 out]
      }
      event "I_next": Value Change {
        n1421 = event-data() -> ("OldVal"=w1779:bool)  [unwired: 1 in, 5 out]
        n1422 = local write "I_next"(w1779) -> ()
        n1423 = local read "I_list_idx"() -> (w1781:i32)
        n1424 = Increment(x=w1781) -> (x+1=w1780:i32)
        n1425 = property on="I_list_idx" class="DigNum (strict)"("Val(Sgnl)"=w1780) -> ()  [unwired: 2 in, 2 out]
      }
      event "I_prev": Value Change {
        n1426 = event-data() -> ("OldVal"=w1782:bool)  [unwired: 1 in, 5 out]
        n1427 = local write "I_prev"(w1782) -> ()
        n1428 = local read "I_list_idx"() -> (w1784:i32)
        n1429 = Decrement(x=w1784) -> (x-1=w1783:i32)
        n1430 = property on="I_list_idx" class="DigNum (strict)"("Val(Sgnl)"=w1783) -> ()  [unwired: 2 in, 2 out]
      }
      event "I_Clear": Value Change {
        n1431 = event-data() -> ()  [unwired: 1 in, 6 out]
        n1432 = flat-sequence {
          frame #0 {
            n1433 = local write "I_list"(dbl[][] [] ("I_list")) -> ()
          }
          frame #1 {
            n1434 = property on="I_tofirst" class="Bool (strict)"("Val(Sgnl)"=TRUE ("Value (Signaling)")) -> ()  [unwired: 2 in, 2 out]
          }
        }
      }
      event "I_list_idx": Value Change {
        w1808 = 10  # Lines to scroll
        n1435 = event-data() -> ("NewVal"=w1791:i32)  [unwired: 1 in, 5 out]
        n1436 = Array Size(array="I_list") -> (size(s)=w1794:i32[])
        n1437 = Index Array(array=w1794) -> (element=w1792:i32)  [unwired: 1 in]
        n1438 = Get Date/Time In Seconds() -> (seconds since 1Jan1904=w1788:timestamp)
        n1439 = local write "I_list_idx_max"(w1792) -> ()
        n1440 = To Double Precision Float(number=w1788) -> (double precision float=w1787:dbl)
        n1441 = local write "Time Old"(w1787) -> ()
        n1442 = In Range and Coerce(upper limit=w1792, x=w1791, lower limit=1) -> (coerced(x)=w1789:i32)  [unwired: 1 out]
        "I_list_idx" <- w1789
        n1443 = Decrement(x=w1789) -> (x-1=w1790:i32)
        n1444 = Initialize Array(FALSE, w1808) -> (w1809:bool[])
        n1445 = Index Array(array="I_list", index (row)=w1790) -> (element=w1811:dbl[])  [unwired: 1 in]
        n1446 = local write "I_list[i]"(w1811) -> ()
        n1447 = Subtract(x=w1790, y=w1808) -> (x-y=w1798:i32)
        n1448 = Increment(x=w1798) -> (x+1=w1797:i32)
        n1449 = Decrement(x=w1808) -> (x-1=w1806:i32)
        n1450 = In Range and Coerce(upper limit=inf, x=w1797, lower limit=0) -> (coerced(x)=w1796:dbl)  [unwired: 1 out]
        n1451 = In Range and Coerce(upper limit=w1806, x=w1790, lower limit=0) -> (coerced(x)=w1803:i32)  [unwired: 1 out]
        n1452 = control-ref of="I_list"() -> (w1801:refnum<vi>)
        n1453 = Build Array(w1796, 0 ("element")) -> (w1802:dbl[])
        n1454 = Replace Array Subset(array=w1809, new element=TRUE ("new element/subarray"), index=w1803) -> (→"I_selection":bool[])
        n1455 = property class="Arr (strict)"(reference=w1801, "Index Values"=w1802) -> ()  [unwired: 1 in, 2 out]
      }
      event "Save to file": Value Change {
        n1456 = event-data() -> ()  [unwired: 1 in, 6 out]
        n1457 = call "File Dialog6"() -> ("selected path"=w1814:path, "cancelled"=w1813:bool)  [unwired: 12 in, 2 out]
        n1458 = case shown="False" w1813 {
          tunnel: w1814 -> [w1815 _]
          frame False {
            n1459 = local read "I_list"() -> (w1817:dbl[][])
            n1460 = call <vilib>:"Write To Spreadsheet File (DBL).vi"("format (%.3f)"="%.1f", "2D data"=w1817, "file path (dialog if empty)"=w1815) -> ()  [unwired: 5 in, 1 out]
          }
          frame True {
          }
        }
      }
      event "Load from file": Value Change {
        n1461 = event-data() -> ()  [unwired: 1 in, 6 out]
        n1462 = call "File Dialog5"() -> ("selected path"=w1818:path, "cancelled"=w1819:bool)  [unwired: 12 in, 2 out]
        n1463 = case shown="False" w1819 {
          tunnel: w1818 -> [w1820 _]
          frame False {
            n1464 = call <vilib>:"Read From Spreadsheet File (DBL).vi"("file path (dialog if empty)"=w1820) -> ("all rows"=w1821:dbl[][])  [unwired: 6 in, 4 out]
            n1465 = local write "I_list"(w1821) -> ()
          }
          frame True {
          }
        }
      }
      event "Write to log": Value Change {
        n1466 = event-data() -> ()  [unwired: 1 in, 6 out]
        n1467 = property on="TempStabilized" class="TypRef (strict)"() -> ("Value"=w1823:refnum<user-event>)  [unwired: 2 in, 2 out]
        n1468 = Generate User Event(user event=w1823, event data cluster=FALSE ("event data")) -> ()  [unwired: 2 in, 2 out]
      }
      event "Set Color": Value Change {
        n1469 = event-data() -> ()  [unwired: 1 in, 6 out]
        n1470 = property on="ColorBox" class="TabCtl (strict)"("Visible"=TRUE) -> ()  [unwired: 2 in, 2 out]
      }
      event "ColorBox": Mouse Move {
        n1471 = event-data() -> ("Coords"=w1827:T48)  [unwired: 1 in]
        n1472 = call <vilib>:"Picture to Pixmap.vi"("picture"="Colors") -> ("image data"=w1833:T47)  [unwired: 9 in, 1 out]
        n1473 = property on="Colors" class="Pict"() -> ("Position"=w1826:T53)  [unwired: 2 in, 2 out]
        n1474 = call <vilib>:"Unflatten Pixmap.vi"("image data"=w1833) -> ("24-bit pixmap"=w1828:u32[][])  [unwired: 4 in, 6 out]
        n1475 = Subtract(x=w1827, y=w1826) -> (x-y=w1831:T48)
        n1476 = Unbundle(w1831) -> ("Horizontal"=w1830:i32, "Vertical"=w1829:i32)
        n1477 = Index Array(array=w1828, index (row)=w1829, index (col)=w1830) -> (element=→"Color":u32)
      }
      event "ColorBox": Mouse Down {
        n1478 = event-data() -> ()  [unwired: 1 in, 8 out]
        n1479 = property on="ColorBox" class="TabCtl (strict)"("Visible"=FALSE) -> ()  [unwired: 2 in, 2 out]
      }
    }
    "General" <- w21
  }
  n1480 = while {
    stop <- w1835 stop-if-true
    # "Main loop"
    n1481 = property on="start 2" class="Bool (strict)"() -> ("Value"=w1837:bool)  [unwired: 2 in, 2 out]
    n1482 = Wait (ms)(milliseconds to wait=u32 200) -> ()  [unwired: 1 out]
    n1483 = case shown="True" w1837 {
      frame False {
        n1484 = Wait (ms)(milliseconds to wait=u32 250) -> ()  [unwired: 1 out]
      }
      frame True {
        n1485 = while {
          i -> [w1849]
          stop <- "Stop" stop-if-true
          # "AVS/zBridge read-out"
          n1486 = case shown="False" "Pause" {
            tunnel: w1849 -> [w1856 _]
            frame False {
              # "for the first measurement set Stab.Time=12 s to do autoranging"
              n1487 = property on="AVS Runtime Settings" class="Clust (strict)"() -> ("Value"=w1873:T17)  [unwired: 2 in, 2 out]
              n1488 = Unbundle By Name(w1873) -> ("Stabilisation Delay"=w1864:dbl, "Averages"=w1857:u16, "Last Channel"=w1872:i8, "Read AVS channels from"=w1871:i8)
              n1489 = local read "Active"() -> (w1854:T12)
              n1490 = property on="AVS type" class="Enum (strict)"() -> ("Value"=w1869:T35)  [unwired: 2 in, 2 out]
              n1491 = call "Split Exc&Range.vi"("Excitations 2"="Exc&Ranges") -> ("Excitations"=w1861:T18, "Ranges"=w1855:T54)  [unwired: 4 in]
              n1492 = property on="AVS VISA session" class="VISAName"() -> ("Value"=w1870:refnum<visa-resource-name>)  [unwired: 2 in, 2 out]
              n1493 = Cluster To Array(cluster=w1854) -> (array=w1853:bool[])
              n1494 = call "If First Iteration.vi"("Iteration"=w1856, "Value In"=w1864, "Default"=12.0) -> ("Value Out"=w1863:dbl)
              n1495 = case shown="\"Impedance Bridge\"" w1869 {
                tunnel: w1870 -> [w1883 w1894 _ _ _ _]
                tunnel: w1863 -> [w1879 w1897 w1899 w1909 _ _]
                tunnel: w1857 -> [w1880 w1896 _ _ _ _]
                tunnel: w1872 -> [w1881 w1892 _ _ _ _]
                tunnel: w1871 -> [w1882 w1893 _ _ _ _]
                tunnel: w1861 -> [w1884 w1888 _ _ _ _]
                tunnel: [w1875 w1887 errorcluster {"status"=FALSE, "code"=0, "source"=""} ("error out") errorcluster {"status"=FALSE, "code"=0, "source"=""} ("error out") w1929 errorcluster {"status"=FALSE, "code"=0, "source"=""} ("error out")] -> w1860
                tunnel: w1855 -> [w1877 w1890 w1904 w1910 w1930 w1934]
                tunnel: "Autorange" -> [w1878 w1891 _ _ _ _]
                tunnel: [w1876 w1889 w1904 w1910 w1930 w1934] -> w1852
                tunnel: [w1874 w1886 dbl[] [] ("Data array") w1908 w1921 dbl[] [] ("Data array")] -> w1858
                tunnel: w1853 -> [_ w1885 _ _ _ _]
                frame "AVS47A (GPIB interface)" {
                  # "AVS 47 (GPIB)"
                  n1496 = call "AVS_do_single_scan.vi"("AVS Port"=w1883, "Stabilization Delay"=w1879, "Autorange"=w1878, "Number of Averages"=w1880, "Last Channel"=w1881, "First Channel"=w1882, "Excitations"=w1884, "Ranges"=w1877) -> ("error out"=w1875:errorcluster, "R"=w1874:dbl[], "Ranges"=w1876:T55)  [unwired: 3 in, 2 out]
                }
                frame "AVS47B (RS232 interface)" {
                  # "AVS 47B (RS232)"
                  n1497 = Type Cast(type=refnum<visa-resource-name> refnum ("dup VISA session"), x=w1894) -> (*(type *) &x=w1898:refnum<visa-resource-name>)
                  n1498 = call "Scanner.vi"("STABILIZATION  DELAY"=w1897, "FIRST CH TO SCAN"=w1893, "LAST CH TO SCAN"=w1892, "Autorange"=w1891, "AVERAGE COUNT"=w1896, "Excitation"=w1888, "Range"=w1890, "VISA resource"=w1898, "array"=w1885) -> ("RI"=w1886:dbl[], "Range out"=w1889:T56, "error out 2"=w1887:errorcluster)  [unwired: 1 in, 3 out]
                }
                frame "AVS48" {
                  n1499 = Multiply(x=w1899, y=u32 1000 ("milliseconds to wait")) -> (x*y=w1900:dbl)
                  n1500 = Wait (ms)(milliseconds to wait=w1900) -> ()  [unwired: 1 out]
                  n1501 = call "AVS48 Single Scan.vi"() -> ()  [unwired: 12 in]
                }
                frame "AVS Emulation" {
                  n1502 = local read "I_in"() -> (w1906:dbl[])
                  n1503 = Multiply(x=w1909, y=u32 1000 ("milliseconds to wait")) -> (x*y=w1918:dbl)
                  n1504 = Wait (ms)(milliseconds to wait=w1918) -> ()  [unwired: 1 out]
                  n1505 = Index Array(array=w1906, index=3) -> ()  [unwired: 1 out]
                  n1506 = property on="I" class="Arr (strict)"() -> ("Value"=w1917:dbl[])  [unwired: 2 in, 2 out]
                  n1507 = Multiply(x=1000.0, y=w1917) -> (x*y=w1912:dbl[])
                  n1508 = Index Array(array=w1912, index #1=2 ("index"), index #2=3 ("index")) -> (element #1=w1913:dbl, element #2=w1914:dbl)
                  n1509 = call "AVS Emulate.vi"("I_mc"=w1914, "I_still"=w1913, "Sampling time"=w1909) -> ("R"=w1908:dbl[])  [unwired: 1 out]
                }
                frame "Impedance Bridge" {
                  n1510 = local read "Bridge status"() -> (w1922:errorcluster)
                  n1511 = local read "zDll"() -> (w1931:path)
                  n1512 = call "Read Data from Single Channel.vi"("error in (no error)"=w1922, "zDll"=w1931) -> ("error out"=w1929:errorcluster, "Value"=w1926:dbl, "Scan parameters/Error string"=→"zBridge params/Error":string, "Set number"=w1927:u8, "Error code"=→"Error code":u8, "Unit"=→"Unit":string, "Scan Parameters"=→"Scan Parameters":cluster{string, "Freq":dbl, "V_exc":dbl})  [unwired: 3 in]
                  "zBridge set nr." <- w1927
                  n1513 = Replace Array Subset(array="Data array", new element=w1926, index=w1927) -> (w1921:dbl[])
                }
                frame "Disabled", Default {
                }
              }
              "Bridge status" <- w1860
              n1514 = property on="Delay" class="DigNum (strict)"() -> ("Value"=w1868:u32)  [unwired: 2 in, 2 out]
              n1515 = property on="Data array" class="Arr (strict)"("Val(Sgnl)"=w1858) -> ()  [unwired: 2 in, 2 out]
              n1516 = property on="Ranges" class="Clust (strict)"("Val(Sgnl)"=w1852) -> ()  [unwired: 2 in, 2 out]
              n1517 = Multiply(x=u32 1000, y=w1868) -> (x*y=w1867:u32)
              n1518 = Wait (ms)(milliseconds to wait=w1867) -> ()  [unwired: 1 out]
            }
            frame True {
            }
          }
        }
        n1519 = while {
          stop <- w1936 stop-if-true
          (unwired) errorcluster {"status"=FALSE, "code"=0, "source"=""} ("Value")
          # "Current source control"
          n1520 = property on="CS status" class="Clust (strict)"() -> ("Value"=w1935:errorcluster)  [unwired: 2 in, 2 out]
          n1521 = stacked-sequence {
            seq-local: [w1964 _ _ _] -> [_ w1973 _ _]
            seq-local: [w1963 _ _ _] -> [_ w1972 _ _]
            seq-local: [_ w1973 _ _] -> [_ _ w1983 _]
            seq-local: [_ w1971 _ _] -> [_ _ w1982 _]
            tunnel: w1935 -> [w1962 _ _ _]
            frame #0 {
              # "Write 0 instead of the actual \ncurrent value to log if there \nis no current flow."
              # "Read current CS status"
              n1522 = local read "CS ref"() -> (w1952:refnum<class "CS.lvclass">)
              n1523 = property on="TCS port" class="Ring (strict)" props=["Value"]() -> ()  [unwired: 2 in, 3 out]
              n1524 = call-dynamic "Read.vi"("CS in"=w1952, "error in (no error)"=w1962, "Optional"=FALSE) -> ("CS out"=w1964:refnum<class "CS.lvclass">, "I0"=w1955:T57, "I1"=w1956:T57, "I2"=w1957:T57, "I3"=w1958:T57, "error out"=w1963:errorcluster)  [unwired: 11 in]
              n1525 = Unbundle By Name(w1955) -> ("Current (string)"=w1950:string, "I?"=w1949:bool)
              n1526 = Unbundle By Name(w1956) -> ("Current (string)"=w1965:string, "I?"=w1948:bool)
              "Current1flow" <- w1948
              n1527 = Unbundle By Name(w1957) -> ("Current (string)"=w1953:string, "I?"=w1947:bool)
              n1528 = Unbundle By Name(w1958) -> ("Current (string)"=w1966:string, "I?"=w1946:bool)
              n1529 = call "CS Data Converter.vi"("CS Data"=w1955) -> ("CS Indicator"=→"I0":T58)
              n1530 = call "CS Data Converter.vi"("CS Data"=w1956) -> ("CS Indicator"=→"I1":T58)
              n1531 = call "CS Data Converter.vi"("CS Data"=w1957) -> ("CS Indicator"=→"I2":T58)
              n1532 = call "CS Data Converter.vi"("CS Data"=w1958) -> ("CS Indicator"=→"I3":T58)
              n1533 = Fract/Exp String To Number(string=w1950) -> (number=w1954:dbl)  [unwired: 3 in, 1 out]
              n1534 = Fract/Exp String To Number(string=w1965) -> (number=w1961:dbl)  [unwired: 3 in, 1 out]
              n1535 = Fract/Exp String To Number(string=w1953) -> (number=w1960:dbl)  [unwired: 3 in, 1 out]
              n1536 = Fract/Exp String To Number(string=w1966) -> (number=w1959:dbl)  [unwired: 3 in, 1 out]
              n1537 = Build Array(w1949, w1948, w1947, w1946) -> (w1945:bool[])
              n1538 = Not(x=w1945) -> (.not. x?=w1941:bool[])
              n1539 = Build Array(w1954, w1961, w1960, w1959) -> (w1944:dbl[])
              "I" <- w1944
              n1540 = for {
                tunnel: w1941 -> [w1970] mode=indexing
                tunnel: w1944 -> [w1969] mode=indexing
                tunnel: dbl[] [0.0, 0.0, 0.0, 0.0] ("t") -> [w1968] mode=indexing
                tunnel: [w1967] -> w1942 mode=indexing
                n1541 = Select(t=w1968, s=w1970, f=w1969) -> (s? t:f=w1967:dbl)
              }
              "Actual I" <- w1942
            }
            frame #1 {
              n1542 = Wait (ms)(milliseconds to wait=100) -> ()  [unwired: 1 out]
              n1543 = call <vilib>:"Clear Errors.vi"("error in (no error)"=w1972) -> ("error out"=w1971:errorcluster)  [unwired: 5 in, 1 out]
            }
            frame #2 {
              # "Only send data to CS if\nnew value was entered"
              # "Set CS status"
              n1544 = call "CS OnOff & Gated and Current & Range.vi"("I in"="C_I0") -> ("OnOff & Gated"=w1994:T59, "Current & Range"=w1979:T60, "I out"=w1987:T61)  [unwired: 2 in]
              n1545 = call "CS OnOff & Gated and Current & Range.vi"("I in"="C_I1") -> ("OnOff & Gated"=w1993:T59, "Current & Range"=w1978:T60, "I out"=w1984:T61)  [unwired: 2 in]
              n1546 = call "CS OnOff & Gated and Current & Range.vi"("I in"="C_I2") -> ("OnOff & Gated"=w1990:T59, "Current & Range"=w1977:T60, "I out"=w1985:T61)  [unwired: 2 in]
              n1547 = call "CS OnOff & Gated and Current & Range.vi"("I in"="C_I3") -> ("OnOff & Gated"=w1989:T59, "Current & Range"=w1976:T60, "I out"=w1986:T61)  [unwired: 2 in]
              n1548 = local write "C_I0"(w1987) -> ()
              n1549 = local write "C_I1"(w1984) -> ()
              n1550 = local write "C_I2"(w1985) -> ()
              n1551 = local write "C_I3"(w1986) -> ()
              n1552 = local read "I_in"() -> (w1975:dbl[])
              n1553 = Equal To 0?(x="CS Mode") -> (x = 0?=w1980:bool)
              n1554 = call "CS_set_channels.vi"("CS in"=w1983, "Current & Range0"=w1979, "Current & Range1"=w1978, "Current & Range 2"=w1977, "Current & Range3"=w1976, "error out"=w1982, "I 2"=w1975, "Auto?"=w1980) -> ("CS.lvclass out"=w1999:refnum<class "CS.lvclass">, "Current Changed?"=w1996:bool, "error out 2"=w2000:errorcluster)  [unwired: 9 in]
              n1555 = call-dynamic "Set Mode.vi"("CS.lvclass in"=w1999, "On&G 0"=w1994, "On&G 1"=w1993, "On&G 2"=w1990, "On&G 3"=w1989, "error in (no error)"=w2000) -> ("CS.lvclass out"=w1997:refnum<class "CS.lvclass">, "error out"=w1998:errorcluster)  [unwired: 12 in]
              n1556 = case shown="False" w1996 {
                selector: w1996 -> [_ w2001]
                frame False {
                }
                frame True {
                  n1557 = property on="Currents changed" class="Bool (strict)"("Val(Sgnl)"=w2001) -> ()  [unwired: 2 in, 2 out]
                }
              }
              n1558 = local write "CS ref"(w1997) -> ()
              n1559 = property on="CS status" class="Clust (strict)"("Value"=w1998) -> ()  [unwired: 2 in, 2 out]
            }
            frame #3 {
              n1560 = Wait (ms)(milliseconds to wait=100) -> ()  [unwired: 1 out]
            }
          }
          n1561 = local read "Stop"() -> (w1936:bool)
        }
        n1562 = while {
          stop <- w1841 stop-if-true
          # "zBridge status read-out"
          n1563 = property on="AVS type" class="Enum (strict)"() -> ("Value"=w1839:T35)  [unwired: 2 in, 2 out]
          n1564 = case shown="\"Impedance Bridge\"" w1839 {
            frame Default {
            }
            frame "Impedance Bridge" {
              n1565 = local read "Bridge status"() -> (w1846:errorcluster)
              n1566 = local read "zDll"() -> (w1847:path)
              n1567 = call "ScanStatus.vi"("error in (no error)"=w1846, "zDll"=w1847) -> ("error out"=w1845:errorcluster, "Status"=w1843:i32, "Channel"=w1844:i32)  [unwired: 7 in]
              n1568 = local write "Bridge status"(w1845) -> ()
              n1569 = call "zBridge Format Status.vi"("Status"=w1843, "Channel"=w1844) -> ("Status"=→"Status":T62, "Active channel"=→"Active channel":T63)  [unwired: 2 in]
            }
          }
          n1570 = Wait (ms)(milliseconds to wait=u32 200) -> ()  [unwired: 1 out]
          n1571 = local read "Stop"() -> (w1841:bool)
        }
      }
    }
    n1572 = local read "Stop"() -> (w1835:bool)
  }
  n1573 = disable-structure shown="Disabled" {
    frame Disabled {
      w2007 = string[] ["Paste Data from Clipboard"] ("item names")
      (unwired) enum32{"Page 1"}."Page 1" ("Tab Control 4")
      n1574 = local read "Scan Parameters"() -> ()  [unwired: 1 out]
      n1575 = local read "Active"() -> ()  [unwired: 1 in]
      n1576 = property class="XYGraph (strict)" props=["YScale", "Mapping Mode"]() -> ()  [unwired: 2 in, 3 out]
      n1577 = Insert Menu Items(4:4, 7:w2007, 8:w2007) -> ()  [unwired: 3 in, 3 out]
      n1578 = property on="ON" class="Boolean (strict)"() -> ("Value"=w2014:bool)  [unwired: 2 in, 2 out]
      n1579 = control-ref of="Active"() -> ()  [unwired: 1 out]
      n1580 = Exclusive Or(1:w2014, 2:TRUE ("x")) -> (0:w2013:bool)
      n1581 = property on="Toggle ON/OFF" class="Bool (strict)"("Value"=w2013) -> ()  [unwired: 2 in, 2 out]
      n1582 = control-ref of="I_list"() -> (w2009:refnum<vi>)
      n1583 = property on="ResetPIDloop" class="TypRef (strict)"() -> ("Value"=w2019:refnum<user-event>)  [unwired: 2 in, 2 out]
      n1584 = property class="Arr (strict)"(reference=w2009) -> ("Index Values"=w2010:u32[])  [unwired: 1 in, 2 out]
      n1585 = Generate User Event(user event=w2019, event data cluster="" ("event data")) -> ()  [unwired: 2 in, 2 out]
      n1586 = Index Array(array=w2010) -> (element=w2011:u32)  [unwired: 1 in]
      n1587 = property on="Tab Control 2" class="TabCtl (strict)"() -> ("Pages"=w2015:refnum<vi>[])  [unwired: 2 in, 2 out]
      n1588 = property on="I_list_idx" class="DigNum (strict)"("Val(Sgnl)"=w2011) -> ()  [unwired: 2 in, 2 out]
      n1589 = Index Array(array=w2015, index=1) -> (element=w2016:refnum<vi>)
      n1590 = Generate User Event(event data cluster="" ("event data")) -> ()  [unwired: 3 in, 2 out]
      n1591 = property class="Page"(reference=w2016, "PageVis"=TRUE ("Page Visible")) -> ()  [unwired: 1 in, 2 out]
      n1592 = local read "Error"() -> ()  [unwired: 1 out]
      n1593 = local read "Int"() -> ()  [unwired: 1 out]
      n1594 = local read item#-1() -> ()  [unwired: 1 out]
      n1595 = Initialize Array(0.0 ("element"), 4 ("dimension size")) -> (w2003:dbl[])
      n1596 = call <userlib>:"MGI Get Slope at Point.vi"() -> ()  [unwired: 11 in, 1 out]
      n1597 = local write "I_in"(w2003) -> ()
      n1598 = call "Write To Spreadsheet File (string) w Error.vi"() -> ()  [unwired: 10 in, 2 out]
    }
    frame Enabled {
    }
  }
  n1599 = control-ref of="Automode Settings 2"() -> ()  [unwired: 1 out]
  n1600 = property on="I3_SP" class="DigNum (strict)" props=["Value"]() -> ()  [unwired: 2 in, 3 out]
